vi "Laundry Tool (Commecial2) Main.vi"() -> ()   [LabVIEW 2021]
uses:
  Common/LabVIEW GEA2 Toolkit/GEA3/type defs/Data In.ctl
  Common/LabVIEW GEA2 Toolkit/GEA3/type defs/Source_Destination.ctl
  Common/LabVIEW GEA2 Toolkit/GEA3/type defs/Data Type.ctl
  Common/LabVIEW GEA2 Toolkit/GEA3/type defs/ERD Read Data In.ctl
  Laundry Tool Support/type defs/Programming.ctl
  Laundry Tool Support/type defs/Flash_Results.ctl
  Laundry Tool Support/type defs/Valves.ctl
  Laundry Tool Support/type defs/Cycle Control.ctl
  Laundry Tool Support/type defs/Motor Control.ctl
  Laundry Tool Support/type defs/MotorProfile.ctl
  Laundry Tool Support/type defs/Relays.ctl
  Laundry Tool Support/type defs/Select _Graph.ctl
  Laundry Tool Support/type defs/ERD_Graph.ctl
  Laundry Tool Support/type defs/ERD_Always_Show.ctl
  Laundry Tool Support/type defs/Redundant.ctl
  Laundry Tool Support/type defs/Algorithms.ctl
  Laundry Tool Support/type defs/ATC_Data.ctl
  Laundry Tool Support/type defs/OOB_Kicks_Brass.ctl
  Laundry Tool Support/type defs/Fault_Buffer_Status.ctl
  Common/GEA2 Script/typedefs/Script Info.ctl
  Laundry Tool Support/type defs/Diagnostics_Table.ctl
  Laundry Tool Support/type defs/Cycle_Diag_Buffer_Status.ctl
  Automation/Product Specific/Clothes Care/TL27/Product Testcode/VALEW/Fault Codes/subVIs/Snap_Input.ctl
  Automation/Product Specific/Clothes Care/TL27/Product Testcode/VALEW/Fault Codes/subVIs/Snap_Selection.ctl
  Dryer Tool (Commercial 2)/JL Dryer Tool Support/type defs/ERD_RJ45.ctl
  Dryer Tool (Commercial 2)/JL Dryer Tool Support/type defs/ERD_Commercial_Laundry.ctl
  Laundry Tool Support/type defs/BootloaderVersion.ctl
  Laundry Tool Support/type defs/Version.ctl
  Laundry Tool Support/type defs/ERD_Data_Loop_Control.ctl
  Laundry Tool Support/type defs/ERD_Loop_States.ctl
  Laundry Tool Support/type defs/Error_Command.ctl
  Laundry Tool Support/type defs/DAQ_States.ctl
  Common/GExplorer Support/typedefs/GExplorer_Data_Cluster.ctl
  Laundry Tool Support/type defs/Cont_Send_States.ctl
  Common/LabVIEW GEA2 Toolkit/GEA3/type defs/Data Out.ctl
  Laundry Tool Support/type defs/All_Bundled_Data.ctl
  Laundry Tool Support/type defs/Brass Matrix.ctl
  Laundry Tool Support/type defs/CSV_File_String_Arrays.ctl
  Laundry Tool Support/type defs/Fault Table Array.ctl
  Laundry Tool Support/type defs/Fault_Table_Info.ctl
  Common/LabVIEW GEA2 Toolkit/GEA3/type defs/ERD Write Data In.ctl
  Laundry Tool Support/type defs/DAQ_Control_Command.ctl
  Laundry Tool Support/type defs/ERD_Loop_Control_Command.ctl
  Laundry Tool Support/type defs/GEA2_Control_Command.ctl
  <vilib>/DAQmx/read.llb/DAQmx Read (Digital 1D Bool NChan 1Samp 1Line).vi
  <vilib>/DAQmx/read.llb/DAQmx Read (Digital 1D U8 1Chan NSamp).vi
  <vilib>/DAQmx/write.llb/DAQmx Write (Digital Bool 1Line 1Point).vi
  <vilib>/DAQmx/read.llb/DAQmx Read (Counter U32 1Chan 1Samp).vi
  <vilib>/DAQmx/write.llb/DAQmx Write (Analog 1D DBL NChan 1Samp).vi
  <vilib>/DAQmx/write.llb/DAQmx Write (Digital 1D Bool NChan 1Samp 1Line).vi
  Common/LabVIEW GEA2 Toolkit/GEA3/advanced/GEA2 Message Received Event Handler.vi
  <vilib>/DAQmx/create/channels.llb/DAQmx Create Channel (DO-Digital Output).vi
  <vilib>/DAQmx/create/channels.llb/DAQmx Create Channel (DI-Digital Input).vi
  <vilib>/DAQmx/configure/timing.llb/DAQmx Timing (Sample Clock).vi
  <vilib>/DAQmx/create/channels.llb/DAQmx Create Channel (CO-Pulse Generation-Frequency).vi
  <vilib>/DAQmx/configure/timing.llb/DAQmx Timing (Implicit).vi
  <vilib>/DAQmx/create/channels.llb/DAQmx Create Channel (CI-Count Edges).vi
  <vilib>/DAQmx/create/channels.llb/DAQmx Create Channel (AO-Voltage-Basic).vi
  <vilib>/DAQmx/miscellaneous.llb/DAQmx Fill In Error Info.vi
  D:/Common/LabVIEW GEA2 Toolkit/source/GEA3 DLL Source/GeaCommunication.dll
  Common/LabVIEW GEA2 Toolkit/source/GEA3 DLL Source/GeaCommunication.dll
  <resource>/objmgr/daqmx.rc
  Common/LabVIEW GEA2 Toolkit/GEA3/library/GEA2_Toolkit.lvlib
  Automation/Product Specific/Clothes Care/TLMB 2019/Projects/TLMB.lvlib
panel:
  in  "EndofCycle":bool
  in  "Board Index":u8=1 max=3 step=1
  in  "Rate":u32
  out "Boolean":bool
  out "String":string="Shutdown"
  in  "Data ON":bool=TRUE
  out "ERD_Always Show":T1
  in  "Stop":bool
  out "Fault Status":bool
  out "Log Rate (ms)":u32=68
  in  "Reset":bool
  in  "LEUI Launch":bool
  in  "HEUI Launch":bool
  in  "Tab Control":T2(tab)=enum."Scripting"
  in  "Phase.Authorized":bool
  in  "Phase.Reserved":bool
  in  "Phase.Idle":bool
  out "Personality Set":u8=1
  in  "?":u8
  in  "Set Personality":bool
  out "CSV File Log Path":path=path "D:/Laundry/FilesTemp/vvxc_[02_11_22_p. m.] [11_30_2021].csv"
  out "RJ45":T3
  out "Commercial_Laundry":T4
  out "Boot Loader Version":T5
  out "Application Version":T6
  in  "Write ERD List":T8(array[cluster])=[{"ERD Number"=0, "Data Type"=enum."string", "Data"=""}] {"ERD Number" format="%.0x"}
  in  "Write ERD":bool
  in  "Read ERD":bool
  in  "Read ERD List":T9[](array[typedef])=[{"ERD Number"=0, "Data Type"=enum."string"}] {"ERD Number" format="%.0x"}
  out "Read ERD Data Out":cluster{"ERD Number":u16, "Data":string}[](array[cluster]) {"ERD Number" format="%.0x"}
  in  "GEA Inputs":T10={"Source"=228, "Destination"=192} {"Destination" format="%.0x"; "Source" format="%.0x"}
  in  "IncrementPrice":T11 {"SANITIZE" min=0.0 max=9.75 step=0.25; "TOWELS" min=0.0 max=9.75 step=0.25; "COLORS" min=0.0 max=9.75 step=0.25; "WHITES" min=0.0 max=9.75 step=0.25; "DELICATES" min=0.0 max=9.75 step=0.25; "SPEED WASH" min=0.0 max=9.75 step=0.25}
  in  "SetIncrementPrices":bool
  in  "BasePrices":T11 {"SANITIZE" min=0.0 max=9.75 step=0.25; "TOWELS" min=0.0 max=9.75 step=0.25; "COLORS" min=0.0 max=9.75 step=0.25; "WHITES" min=0.0 max=9.75 step=0.25; "DELICATES" min=0.0 max=9.75 step=0.25; "SPEED WASH" min=0.0 max=9.75 step=0.25}
  in  "Set Price":bool
  in  "Send Button":bool
  in  "GEA2 Send":T12={"Source"=228, "Destination"=192, "Command"=0, "Message"=""} {"Command" format="%02x"; "Destination" format="%02x"; "Source" format="%02x"}
  in  "Msg Rate (ms)":u32=1000 min=50 step=50
  in  "Start Send":bool
  in  "Save Log":bool
  in  "GEA2 Log Length":i32=100000
  out "GEA2 Log":string
  in  "Clear":bool
  in  "Filter Log":bool
  in  "Cmd":string
  in  "Filter Data":bool
  in  "Programming":T13={"Program"=FALSE, "File Path"=path "", "Program Ind"=FALSE, "Result"=9, "Reset Board"=FALSE, "Enter Bootloader"=FALSE} {"Result" items=["ImageRejected", "BoardNotFound", "UnableToGetGeaConfiguration", "WriteToFlashNotAllowed", "ImageDownloadedSuccessfully", "ImagePresent", "WriteToFlashFailed", "EraseFailed", "CrcFailed", ""]}
  in  "Programming Destination Address":u8=35 format="%.0x"
  in  "ERD Graphing ON":bool
  out "ERD Graph  Ind":T15
  in  "ERD Graph Cntrl":T17={"ERD 3"={"ERD #"=61636, "Data Type"=enum."uint16_t", "Scaler"=32}, "ERD 2"={"ERD #"=61636, "Data Type"=enum."uint16_t", "Scaler"=32}, "ERD 1, ERD 2, & ERD3"={"ERD #"=61636, "Data Type"=enum."uint16_t", "Scaler"=32}} {"ERD 1, ERD 2, & ERD3"."Scaler" min=1; "ERD 1, ERD 2, & ERD3"."ERD #" format="%.0x"; "ERD 2"."Scaler" min=1; "ERD 2"."ERD #" format="%.0x"; "ERD 3"."Scaler" min=1; "ERD 3"."ERD #" format="%.0x"}
  in  "Graphing ON":bool
  in  "Select Graph":T18=enum."All Loads"
  out "Motor Current 2":dbl(graph)
  out "ERD 3":dbl(graph)
  out "ERD 2":dbl(graph)
  out "ERD 1":dbl(graph)
  out "Basket Speed 2":u16[][](graph)
  out "Temp 2":dbl(graph)
  out "Tub Gallons 2":dbl(graph)
  out "Pressure 3":dbl(graph)
  in  "OOB Kicks":T19
  out "All Loads":u16[][](graph)=[[0, 100, 200, 300, 400, 500, 600, 700, 800]]
  in  "Save Fault Log":bool
  in  "Clear Fault Table Buffer":bool
  in  "Clear Fault Seq Buffer":bool
  in  "Fault ON":bool
  out "Fault Table Buffer":string[][](table)
  out "Fault Sequence Buffer":string
  out "Seq Buffer Status":T20
  out "Table Buffer Status":T20
  in  "Clear Snapshots":bool
  in  "Get Snapshot Status":bool
  in  "Get Snapshot":bool
  in  "Select Snapshot":T21
  out "Fault Snapshots":T22
  out "Current Index":u16
  out "Count":u16
  out "Overwrite Count":u16
  out "Board Serial":string
  out "Board SKU":string
  in  "Get Board SKU and Serial":bool
  in  "Value":string
  in  "Register":string
  out "Value":string
  in  "Get Accel Reg":bool
  in  "Register":string
  in  "Set Accel Reg":bool
  in  "Relays":T23
  in  "Motor Profile":T24={"Start Profile"=FALSE, "Profile Selection"=14, "Stop Profile"=FALSE, "Pause Profile"=FALSE, "Resume Profile"=FALSE, "Select Profile"=FALSE}
  in  "Test Mode":cluster{"Exit Test Mode":bool}
  in  "LED Control":T25
  in  "Motor Control":T26 {"Amplitude (%)\n-CCW +CW" min=-100 max=100 step=5; "Acceleration" min=-400 max=400 step=10; "Motor Profile Mode" items=["Closed Loop", "Not Implemented", "Open Loop ", "Open Loop Angle ", "Coasting", "Braking", "Idle"]; "Speed (RPM)" min=-800 max=800 step=10}
  in  "Mode Shift":T27
  in  "Recirculation Pump":T28
  in  "Drain Pump":T29
  in  "Lid Lock":T30
  in  "Cycle Control":T31
  in  "Valve Control":T32
  in  "Save Cycle History Log":bool
  in  "Clear Cycle Buffer":bool
  out "Cycle Buffer Status":T33
  in  "Get Cycle History":bool
  out "Diagnostics Table":T34
  out "Redundant Micro":T35
  out "Algorithm Data":T36
  out "ATC Data":T37
  in  "ADC Info Button":bool
  out "Motor Current ADC":u16
  out "Pressure ADC":u16
  out "Temp ADC":u16
  in  "HE/LE ?":enum16{"HE", "LE"}(ring)
  in  "LL (M - A)":bool=TRUE
  in  "Lid Lock Feedback":bool
  in  "MS (M - A)":bool=TRUE
  out "DAQ Status":string="Exit"
  out "Drain Pump":bool
  out "Mode Shift":bool
  out "Recirc Pump":bool
  out "Cold Valve":bool
  out "Hot Valve":bool
  out "Spray/Rinse Valve":bool
  out "Fabric SoftValve":bool
  in  "AC Power":bool=TRUE
  in  "Mode Shift FB":bool
  in  "Lid Status":bool
  in  "Pressure":dbl(slide) min=0.0 max=5.0 step=0.5 scale=0.0..5.0 scale format="%#_3g"
  in  "Motor Current":dbl(slide)=2.5 min=0.0 max=5.0 step=0.5 scale=0.0..5.0 scale format="%#_3g"
  in  "Turn On DAQ":bool
  out "DAQ On?":bool
  in  "Basket RPM":dbl=1.0 min=1.0 max=800.0 step=5.0
  in  "Temperature":dbl(slide)=2.5 min=0.0 max=5.0 step=0.5 scale=0.0..5.0 scale format="%#_3g"
  out "Triac CW":bool
  out "Traic CCW":bool
  out "CCW":u32
  out "CW":u32
  in  "Script Log Path":path
  in  "Run Script":bool
  out "Script Pass/Fail?":bool
  out "Script Report Text":string
  in  "stop script":bool
  in  "Script Path":path
  out "Script Info":T38 {"Overall Script File Progress" scale=0.0..1.0; "Elapsed time (s)" format="%#.1f"; "Current Script Progress" scale=0.0..1.0}
  out "Script Error Out":errorcluster
  in  "ERD always show":T39(array[cluster])=[{"Boolean"=TRUE, "ERD Number"=61596, "ERD Name"="Erd_MC_WaterValvesActualState", "Data Type"=enum."string"}, {"Boolean"=TRUE, "ERD Number"=61551, "ERD Name"="Erd_MC_LidSwitchState", "Data Type"=enum."string"}, {"Boolean"=TRUE, "ERD Number"=61594, "ERD Name"="Erd_MC_DrainPumpActualState", "Data Type"=enum."string"}, {"Boolean"=TRUE, "ERD Number"=8236, "ERD Name"="Erd_Drive_SpeedSensorBasket", "Data Type"=enum."string"}, {"Boolean"=TRUE, "ERD Number"=8235, "ERD Name"="Erd_Drive_MotorTargetBasketSpeed", "Data Type"=enum."string"}, {"Boolean"=TRUE, "ERD Number"=65314, "ERD Name"="Erd_Drive_ModeShiftActualState", "Data Type"=enum."string"}, {"Boolean"=TRUE, "ERD Number"=61636, "ERD Name"="Erd_Drive_DCBusVoltageAd", "Data Type"=enum."string"}, {"Boolean"=TRUE, "ERD Number"=61546, "ERD Name"="Erd_CurrentCalibratedPressureInchesH2o", "Data Type"=enum."string"}, {"Boolean"=TRUE, "ERD Number"=61549, "ERD Name"="Erd_MC_TargetInGallonsx100", "Data Type"=enum."string"}, {"Boolean"=TRUE, "ERD Number"=61545, "ERD Name"="Erd_MC_CurrentTubInGallonsx100", "Data Type"=enum."string"}, {"Boolean"=TRUE, "ERD Number"=61611, "ERD Name"="Erd_Drive_LoadCurrentRms", "Data Type"=enum."string"}, {"Boolean"=TRUE, "ERD Number"=61544, "ERD Name"="Erd_MC_WetLoadGallons", "Data Type"=enum."string"}, {"Boolean"=TRUE, "ERD Number"=61555, "ERD Name"="Erd_MC_LidLockActualState", "Data Type"=enum."string"}, {"Boolean"=TRUE, "ERD Number"=61617, "ERD Name"="Erd_Drive_MotorMode", "Data Type"=enum."string"}, {"Boolean"=TRUE, "ERD Number"=61623, "ERD Name"="Erd_Drive_CycleEngineActualState", "Data Type"=enum."string"}, {"Boolean"=TRUE, "ERD Number"=8379, "ERD Name"="Erd_WaterTemperatureOption", "Data Type"=enum."string"}, {"Boolean"=TRUE, "ERD Number"=8382, "ERD Name"="Erd_SoilLevelOption", "Data Type"=enum."string"}, {"Boolean"=TRUE, "ERD Number"=8213, "ERD Name"="Erd_Remote_SoilLevelOption", "Data Type"=enum."string"}] {"ERD Number" format="%x"}
  in  "Basic ERDs":T39(array[cluster])=[{"Boolean"=FALSE, "ERD Number"=56, "ERD Name"="Erd_BootLoaderVersion", "Data Type"=enum."string"}, {"Boolean"=TRUE, "ERD Number"=8192, "ERD Name"="Erd_Remote_MachineState", "Data Type"=enum."string"}, {"Boolean"=TRUE, "ERD Number"=65280, "ERD Name"="Erd_Personality", "Data Type"=enum."string"}, {"Boolean"=TRUE, "ERD Number"=65356, "ERD Name"="Erd_Rj45LockedAtLeastOnce", "Data Type"=enum."string"}, {"Boolean"=TRUE, "ERD Number"=2, "ERD Name"="Erd_UnitSerialNumber", "Data Type"=enum."string"}, {"Boolean"=TRUE, "ERD Number"=8350, "ERD Name"="Erd_CommercialLaundryStatusExternal", "Data Type"=enum."string"}, {"Boolean"=TRUE, "ERD Number"=8351, "ERD Name"="Erd_CommercialLaundryStatus", "Data Type"=enum."string"}, {"Boolean"=TRUE, "ERD Number"=8397, "ERD Name"="Erd_RJ45WriteAccessReques", "Data Type"=enum."string"}, {"Boolean"=TRUE, "ERD Number"=8398, "ERD Name"="Erd_RJ45WriteAccessActual", "Data Type"=enum."string"}] {"ERD Number" format="%x"}
  in  "GEA Inputs 2":T10={"Source"=229, "Destination"=192} {"Destination" format="%.0x"; "Source" format="%.0x"}
  in  "Wifi State":T40(ring)
  in  "Set Wifi State(ERD 6003)":bool
  in  "Turn on Wifi":bool
  in  "Turn off Wifi":bool
  out "Wifi Network State":string
  out "Wifi Password":string
  out "Wifi Network Name":string
  out "Mac Address":string
  in  "Get Wifi Data":bool
  out "Error Out":errorcluster
  in  "Error In":errorcluster
  # "Ver. 1.2"
  # "Simular pago con aplicación 209E phase"
  # "Personality"
  # "Set Base Prices"
  # "Set Increment Prices"
  # "Must input a valid ERD# and Data Type\nDO NOT Leave Blank \nIf no scaler use value of 01"
  # "Accelermeter Registers"
  # "Wet Load Size"
  # "Dry Load Size"
  # "OOB"
  # "Wifi State is Writing to ERD 6003 and communicating with the wifi board directly.  It will remain in the state you wrote it to until another command is recieved. \n\nOnly Write to invalid if you are testing the board in Invalid state."
  # "After turning on Wifi , wait about 30 seconds and press the Get Wifi Data button.  Network state should be 1, apmode.\n\nAll this is doing is Writing the ERD 0xF115 Service Request to request connect, or disconnect."
  # "Contact:\n\nChris Schwalm\nChristopher.Schwalm@geappliances.com"
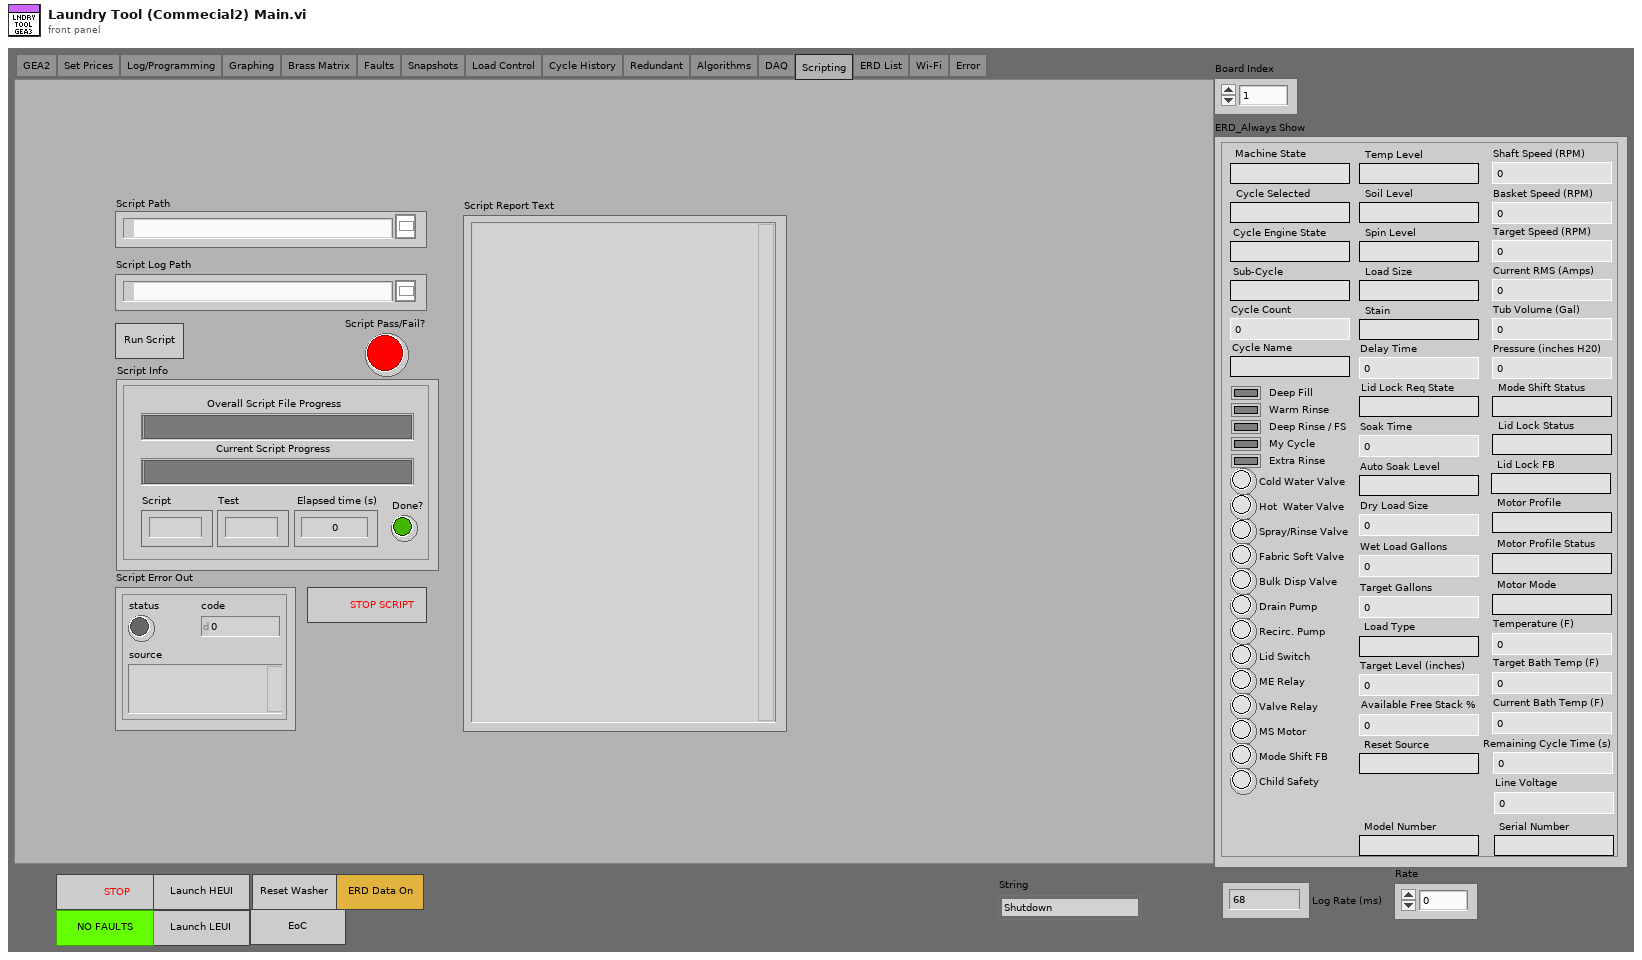
[diagram p1: front panel]
types:
  T1 = typedef "ERD_Always_Show.ctl" = cluster{"Basket Speed (RPM)":u16, "Machine State":string, "Tub Volume (Gal)":dbl, "Pressure (inches H20)":dbl, "Lid Switch ":bool, "Current RMS (Amps)":dbl, "Cycle Selected":string, "Lid Lock Status":string, "Mode Shift Status":string, "Spray/Rinse Valve":bool, "Fabric Soft Valve":bool, "Drain Pump":bool, "Recirc. Pump":bool, "Cycle Engine State":string, "Hot  Water Valve":bool, "Cold Water Valve":bool, "Motor Profile":string, "Motor Profile Status":string, "Motor Mode":string, "ME Relay":bool, "Cycle Count":u32, "Deep Rinse / FS":bool, "My Cycle":bool, "Soil Level":string, "Spin Level":string, "Stain":string, "Temp Level":string, "Load Size":string, "Delay Time":u16, "Soak Time":u16, "Deep Fill":bool, "Warm Rinse":bool, "Auto Soak Level":string, "Extra Rinse":bool, "Wet Load Gallons":dbl, "Target Gallons":dbl, "Sub-Cycle":string, "Load Type":string, "Target Level (inches)":dbl, "Valve Relay":bool, "Dry Load Size":dbl, "Shaft Speed (RPM) ":u16, "MS Motor":bool, "Mode Shift FB":bool, "Target Bath Temp (F)":dbl, "Temperature (F)":dbl, "Current Bath Temp (F)":dbl, "Lid Lock FB":string, "Lid Lock Req State":string, "Remaining Cycle Time (s)":u32, "Available Free Stack %":u8, "Child Safety":bool, "Target Speed (RPM)":u16, "Reset Source":string, "Line Voltage":dbl, "Cycle Name":string, "Bulk Disp Valve":bool, "Model Number":string, "Serial Number":string}
  T2 = enum32{"GEA2", "Set Prices", "Log/Programming", "Graphing", "Brass Matrix", "Faults", "Snapshots", "Load Control", "Cycle History", "Redundant", "Algorithms", "DAQ", "Scripting", "ERD List", "Wi-Fi", "Error"}
  T3 = typedef "ERD_RJ45.ctl" = cluster{"Write Access Actual":string, "Write Access Request":string, "LockedAtLeastOnce":string}
  T4 = typedef "ERD_Commercial_Laundry.ctl" = cluster{"Session":string, "Phase":string, "Appliance Type":string, "Cycle Selected":string, "Platform Type":string, "Retry Signal":string, "Session Ext":string, "Phase Ext":string, "Appliance Type Ext":string, "Cycle Selected Ext":string, "Platform Type Ext":string, "Retry Signal Ext":string}
  T5 = typedef "BootloaderVersion.ctl" = cluster{"UI BL Version":string, "MC BL Version":string}
  T6 = typedef "Version.ctl" = cluster{"Build Number":string, "Build Hash ":string, "Application Version":string, "Parametric Version":string, "UI App Version":string}
  T7 = typedef "Data Type.ctl" = enum16{"string", "boolean", "uint8_t", "uint16_t", "uint32_t", "uint64_t", "int8_t", "int16_t", "int32_t", "int64_t"}
  T8 = cluster{"ERD Number":u16, "Data Type":T7, "Data":string}[]
  T9 = typedef "ERD Read Data In.ctl" = cluster{"ERD Number":u16, "Data Type":enum16{"string", "boolean", "uint8_t", "uint16_t", "uint32_t", "uint64_t", "int8_t", "int16_t", "int32_t", "int64_t"}}
  T10 = typedef "Source_Destination.ctl" = cluster{"Source":u8, "Destination":u8}
  T11 = cluster{"SPEED WASH":dbl, "DELICATES":dbl, "WHITES":dbl, "COLORS":dbl, "TOWELS":dbl, "SANITIZE":dbl}
  T12 = typedef "Data In.ctl" = cluster{"Source":u8, "Destination":u8, "Command":u8, "Message":string}
  T13 = typedef "Programming.ctl" = cluster{"Program":bool, "File Path":path, "Program Ind":bool, "Result":T14, "Reset Board":bool, "Enter Bootloader":bool}
  T14 = typedef "Flash_Results.ctl" = i32
  T15 = cluster{"ERD Value 1":dbl, "ERD Value 2":dbl, "ERD Value 3":dbl}
  T16 = typedef "ERD_Graph.ctl" = cluster{"ERD #":u16, "Data Type":T7, "Scaler":u32}
  T17 = cluster{"ERD 3":T16, "ERD 2":T16, "ERD 1, ERD 2, & ERD3":T16}
  T18 = typedef "Select _Graph.ctl" = enum16{"Temperature (F)", "Basket Speed (RPM)", "Tub Volume (Gal)", "Pressure (in H2O)", "Current RMS (Amps)", "ERD 1", "ERD 2", "ERD 3", "All Loads"}
  T19 = typedef "OOB_Kicks_Brass.ctl" = cluster{"OOB in Accel":bool, "OOB in S-S":bool, "Redist Req":bool, "Suds Abtmt Req":bool}
  T20 = typedef "Fault_Buffer_Status.ctl" = cluster{"Current Index":u16, "Count":u16, "Overwrite Count":u16}
  T21 = typedef "Snap_Selection.ctl" = enum16{"SnapShot Record 0 - E10F", "Snapshot Record 1 - E110", "Snapshot Record 2 - E111", "Snapshot Record 3 - E112", "Snapshot Record 4 - E113", "Snapshot Record 5 - E114", "Snapshot Record 6 - E115", "Snapshot Record 7 - E116", "Snapshot Record 8 - E117", "Snapshot Record 9 - E118"}
  T22 = typedef "Snap_Input.ctl" = cluster{"Fault ID":string, "Cycle Count":u32, "Cycle ID":string, "Time Stamp":u32, "Stuck Key Mask":string, "Machine State":string, "Subcycle State":string, "Hot Valve":string, "Cold Valve":string, "Spray Valve":string, "Fabric Softener Valve":string, "Bulk Valve":string, "Drain Pump State":string, "Lid Lock Actual":string, "Lid Lock Request":string, "Lid Switch State":string, "ModeShift Feeback":string, "Recirc Pump State":string, "Modeshift Requested":string, "Modeshift Actual":string, "Motor Mode":string, "Target Speed":u16, "Target Accel":u16, "Current RMS(AMPS)":dbl, "Line Voltage":dbl, "Target Gallons":dbl, "Tub Volume (Gal)":dbl, "Hot Gallons":dbl, "Cold Gallons":dbl, "Target Level (Inches)":dbl, "Pressure (Inches H20) ":dbl, "Pressure Calibration":dbl, "OOB Accel":i32, "OOB Jerk":i32, "OOB SS":i32, "OOB Folding":i32, "Accelerometer Peak":i16, "Accelerometer Base":i16, "Accel Points":u8, "SS Points":u8, "Deep Fill Option":string, "WoD Option":string, "Basket Speed":u16}
  T23 = typedef "Relays.ctl" = cluster{"Relays ON":bool, "Relays OFF":bool}
  T24 = typedef "MotorProfile.ctl" = cluster{"Start Profile":bool, "Profile Selection":u8, "Stop Profile":bool, "Pause Profile":bool, "Resume Profile":bool, "Select Profile":bool}
  T25 = cluster{"ALL LEDs ON":bool, "ALL LEDs OFF":bool, "Reset LEDs":bool}
  T26 = typedef "Motor Control.ctl" = cluster{"Speed (RPM)":i16, "Motor Profile Mode":u16, "Acceleration":i16, "Angle (Degrees)":i16, "Amplitude (%)\n-CCW +CW":i16, "Start Motor":bool, "Stop Motor":bool}
  T27 = cluster{"Shift to Agitate":bool, "Shift to Spin":bool, "Disable":bool}
  T28 = cluster{"Recirc Pump ON":bool, "Recirc Pump OFF":bool, "Reset Recirc Pump":bool}
  T29 = cluster{"Drain Pump ON":bool, "Drain Pump OFF":bool, "Reset Drain Pump":bool}
  T30 = cluster{"Lock Lid":bool, "Unlock Lid":bool, "Reset Lock":bool}
  T31 = typedef "Cycle Control.ctl" = cluster{"Start Cycle":bool, "Cycle Selection":u8, "Stop Cycle":bool, "Pause Cycle":bool, "Resume Cycle":bool, "Select Cycle":bool}
  T32 = typedef "Valves.ctl" = cluster{"Cold Valve":bool, "SprayRinse Valve":bool, "FabricSoftener Valve":bool, "Valves ON":bool, "Valves OFF":bool, "Hot Valve ":bool, "Bulk Dispense Valve":bool}
  T33 = typedef "Cycle_Diag_Buffer_Status.ctl" = cluster{"Current Index":u16, "Count":u16, "Overwrite Count":u16}
  T34 = typedef "Diagnostics_Table.ctl" = string[][]
  T35 = typedef "Redundant.ctl" = cluster{"Version":string, "Personality":u8, "Pressure ":dbl, "Shaft Speed":u16, "Modeshift Feedback":string, "Lid Switch":bool, "Lid Lock":bool, "Triac Enable":bool, "Drain Pump":bool, "Lid Lock Motor Speed Safety Interlock":bool, "Flood Condition State":bool, "Lid Open Fault State":bool, "Access To Moving Parts State":bool, "Heartbeat":bool, "Motor Enable":bool, "Lid Unlock Fault State":bool}
  T36 = typedef "Algorithms.ctl" = cluster{"Wet Load Gal":dbl, "Target Gallons":dbl, "Load Type":string, "Load Size":string, "Coast Time":u16, "Ramp Time":u16, "Ramp  Speed":u16, "Ramp Avg Current":dbl, "OOB Redist Req":bool, "OOB Detected in S-S":bool, "Folding in Accel":i32, "Max Jerk in Accel":i32, "Max Jerk in S-S":i32, "OOB Detected in Accel":bool, "Partial Coast Time":u16, "Dry Load Size":dbl, "Ramp Line Voltage ":dbl, "Coast Line Voltage":dbl, "Suds Abatement Req ":bool}
  T37 = typedef "ATC_Data.ctl" = cluster{"Current Tub Gallons":dbl, "Hot Gallons":dbl, "Cold Gallons":dbl, "Target Gallons":dbl, "Current Water Temp":dbl, "Target Level":dbl, "Target Bath Temp":dbl, "Current Bath Temp ":dbl, "Cold Inlet Temp":dbl, "Hot Inlet Temp":dbl, "Warm Inlet Temp":dbl, "Hot Seg Valve Time":u16, "Cold Seg Valve Time ":u16, "User Temp Level":string, "Segment Gallons":dbl}
  T38 = typedef "Script Info.ctl" = cluster{"Overall Script File Progress":dbl, "Current Script Progress":dbl, "Script":string, "Test":string, "Elapsed time (s)":dbl, "Done?":bool}
  T39 = cluster{"Boolean":bool, "ERD Number":u16, "ERD Name":string, "Data Type":enum16{"string", "boolean", "uint8_t", "uint16_t", "uint32_t", "uint64_t"}}[]
  T40 = enum16{"0 - OFF", "1 - App Mode", "2 - Connecting", "3 - Connected", "4 - Connected Off", "5 - Scanning", "6 - Reconnecting", "255 - Invalid"}
  T41 = typedef "All_Bundled_Data.ctl" = cluster{"Software MC":T6, "ERD_Always Show":T1, "Personality Set":u8, "Brass Matrix":T42, "CSV File String Arrays":T43, "Redundant Micro":T35, "Algorithm Data":T36, "ATC Data":T37, "Fault Table Array ":T44, "RJ45":T3, "Commercial_Laundry":T4, "Boot Loader Version":T5}
  T42 = typedef "Brass Matrix.ctl" = cluster{"Shaft Speed":u16, "Folding":i32, "Jerk":i32, "Basket Speed":u16, "Target Speed":u16, "Peak Signal":u8, " Peak Magnitude":dbl, "Folding in Accel":i32, "Max Jerk in Accel":i32, "Max Jerk in S-S":i32, "Motor Profile Status":string, "Motor Profile":string, "OOB Redist Req":bool, "OOB Detected in S-S":bool, "OOB Detected in Accel":bool, "Suds Abatement Req ":bool, "Peak Dir":bool, "Peak Vector":dbl, "S-S Points":u8, "Points":u8, "Jerk Delta":i32}
  T43 = typedef "CSV_File_String_Arrays.ctl" = cluster{"ERD Number Array":string[], "ERD Name Array":string[], "ERD Converted String Data":string[]}
  T44 = typedef "Fault Table Array.ctl" = T45[]
  T45 = typedef "Fault_Table_Info.ctl" = cluster{"Cycle Count":u32, " Runtime (min) ":u32, "Fault Status":string, "Fault ID":string, "Fault Count":u16}
  T46 = typedef "Cont_Send_States.ctl" = enum16{"Run", "Shutdown"}
  T47 = typedef "GExplorer_Data_Cluster.ctl" = cluster{"Data":variant, "State":enum16{"Add to Log", "Clear", "Shutdown"}}
  T48 = typedef "DAQ_States.ctl" = enum16{"Wait for Init", "Rename Devices", "Verify Hardware", "Initialize", "Run", "Shutdown", "Exit"}
  T49 = typedef "ERD_Data_Loop_Control.ctl" = cluster{"Data":variant, "State":T50}
  T50 = typedef "ERD_Loop_States.ctl" = enum16{"Init", "Get Version", "Build ERD Read List", "Read ERDs", "Update UI", "Update Graphs", "Read Faults", "Log Data", "Pause", "Brass Logging", "Shutdown"}
  T51 = typedef "Error_Command.ctl" = enum16{"Initialize", "Handle Errors", "Report Errors"}
  T52 = typedef "ERD Write Data In.ctl" = cluster{"ERD Number":u16, "Data Type":T7, "Data":string}
  T53 = enum8{"Enabled", "Disabled", "Disabled and Grayed Out"}
  T54 = typedef "GEA2_Control_Command.ctl" = enum16{"Initialize", "Shutdown"}
  T55 = typedef "ERD_Loop_Control_Command.ctl" = enum16{"Initialize", "Shutdown"}
  T56 = typedef "DAQ_Control_Command.ctl" = enum16{"Initialize", "Shutdown", "Exit"}
  T57 = typedef "Data Out.ctl" = cluster{"Source":u8, "Destination":u8, "Command":u8, "Length":u8, "CRC":u16, "Message":string}
  T58 = cluster{"ERD Data Out[0]":cluster{"ERD Number":u16, "Data":string}, "ERD Data Out[1]":cluster{"ERD Number":u16, "Data":string}, "ERD Data Out[2]":cluster{"ERD Number":u16, "Data":string}, "ERD Data Out[3]":cluster{"ERD Number":u16, "Data":string}, "ERD Data Out[4]":cluster{"ERD Number":u16, "Data":string}, "ERD Data Out[5]":cluster{"ERD Number":u16, "Data":string}, "ERD Data Out[6]":cluster{"ERD Number":u16, "Data":string}, "ERD Data Out[7]":cluster{"ERD Number":u16, "Data":string}, "ERD Data Out[8]":cluster{"ERD Number":u16, "Data":string}}
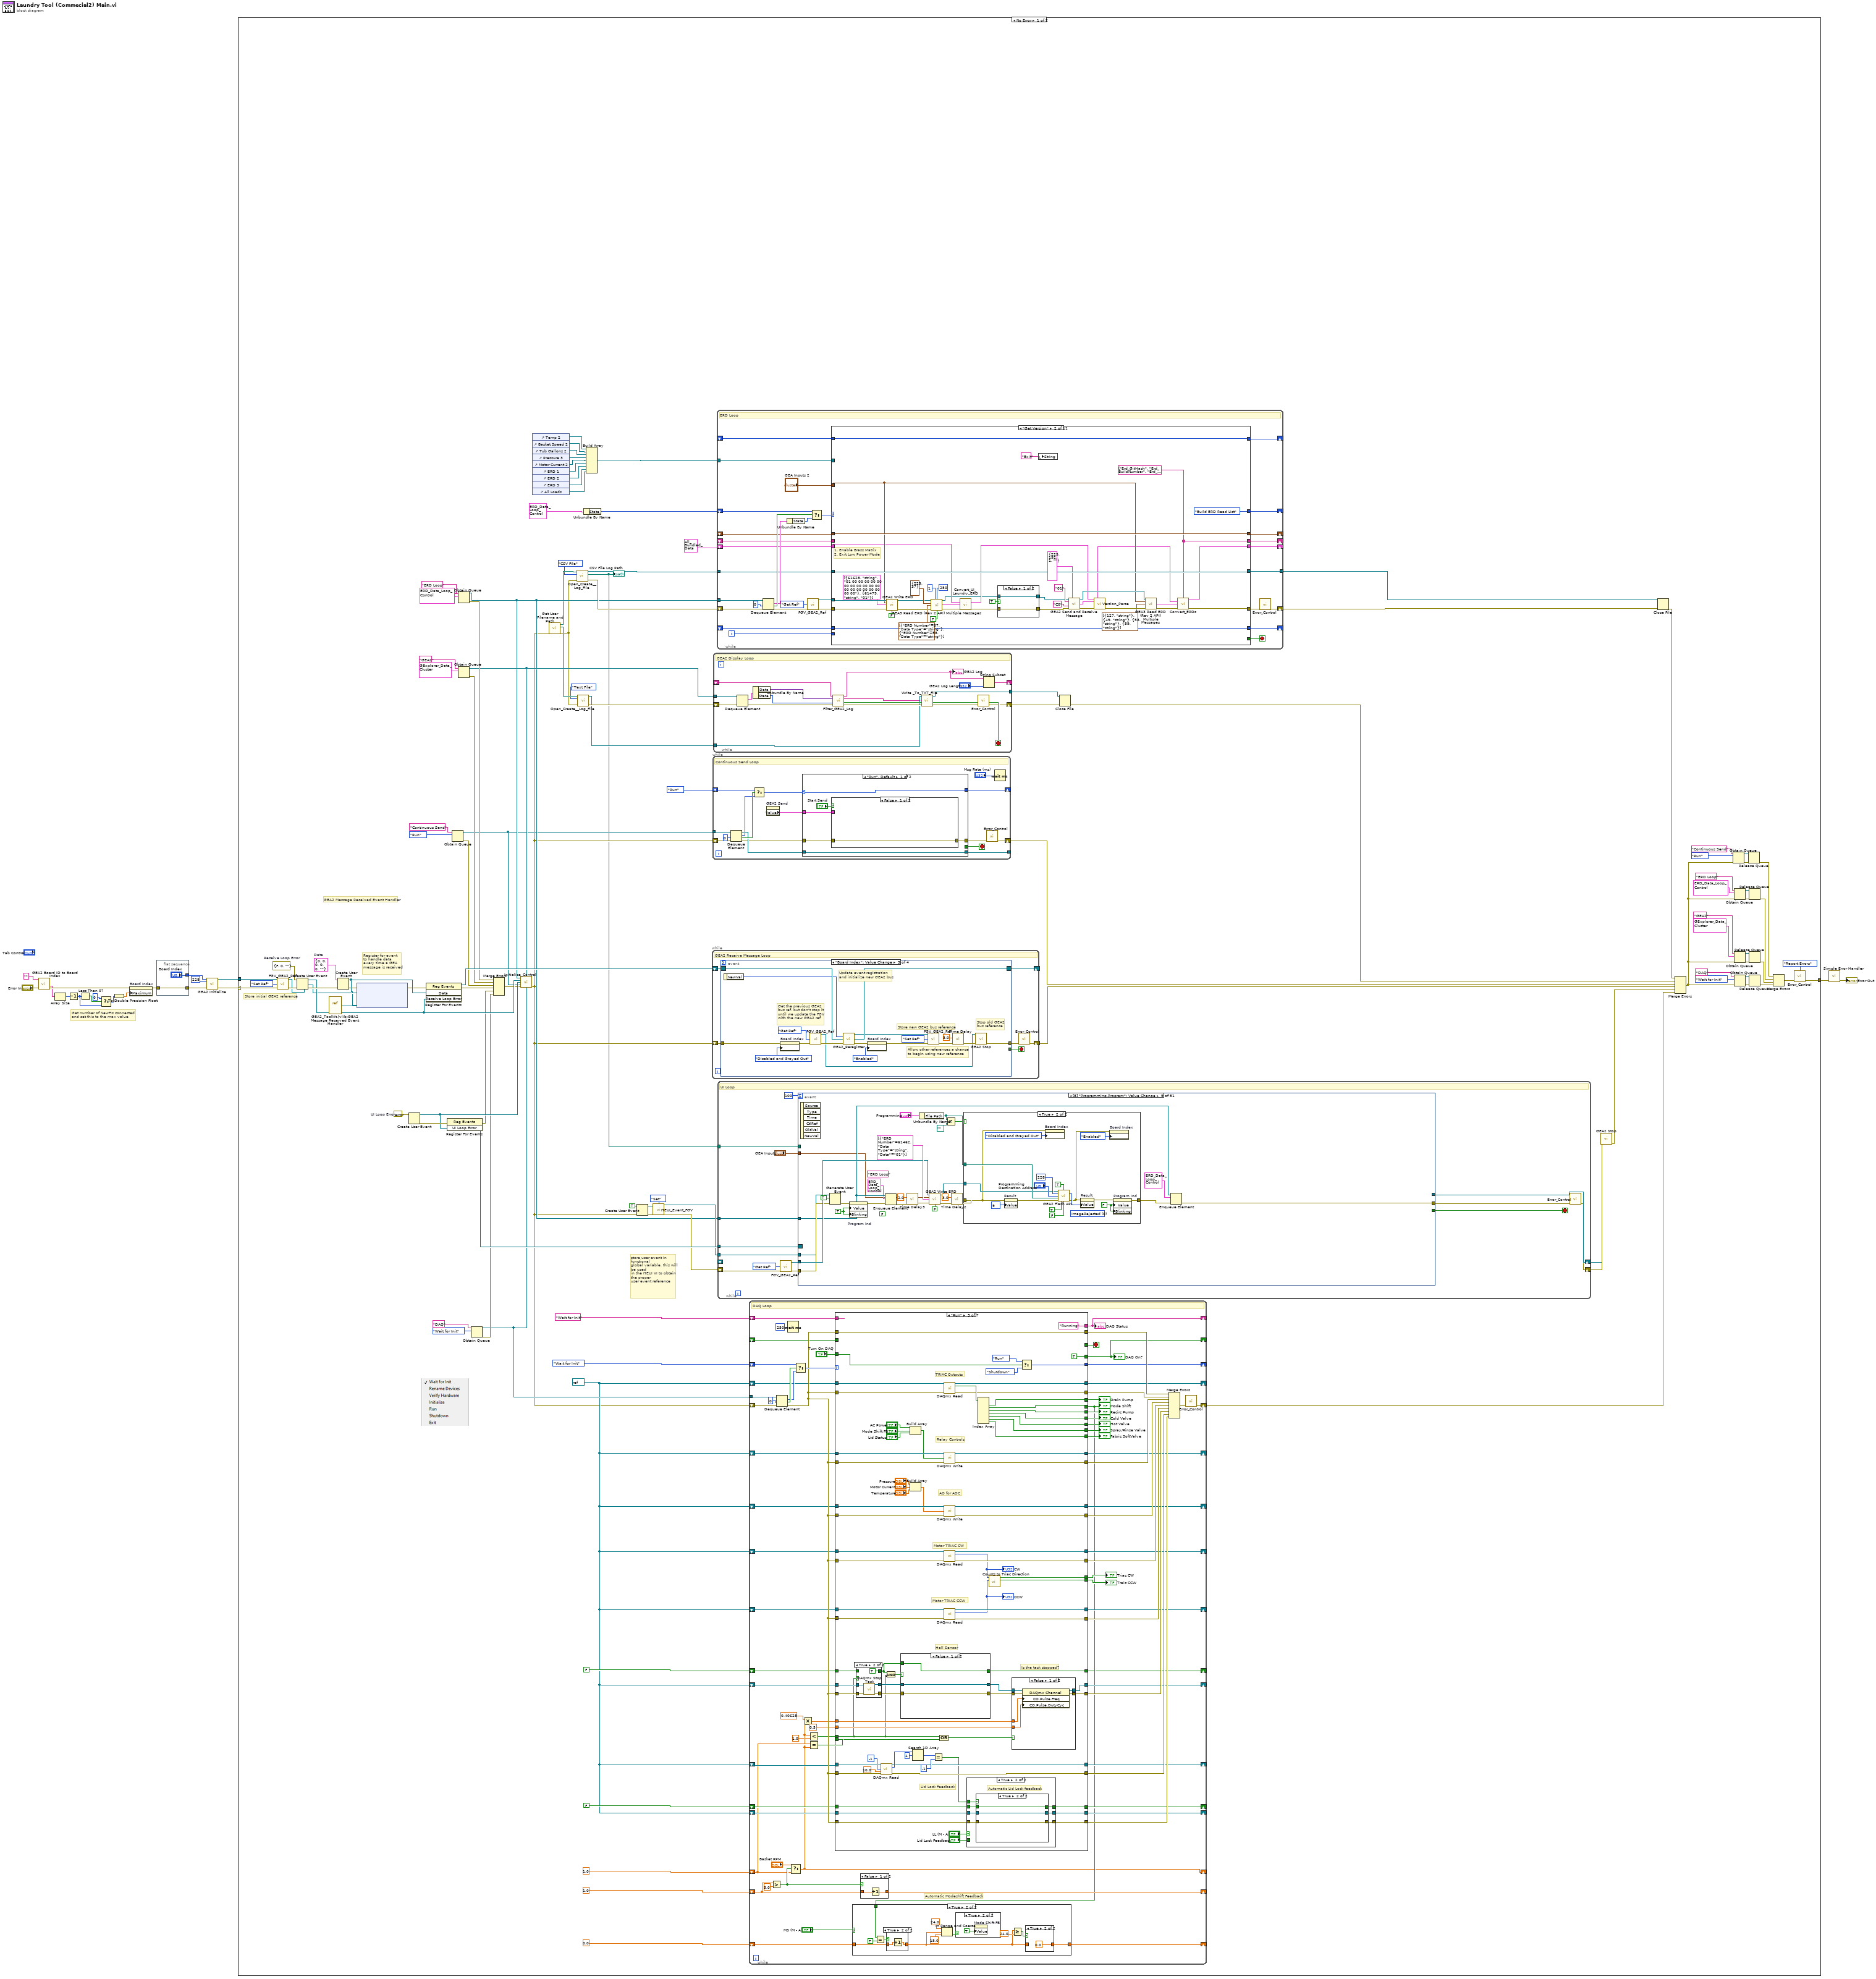
[diagram p0: block diagram]
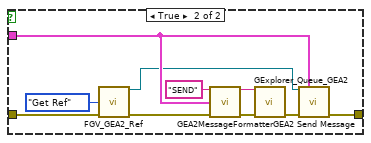
[diagram p2: hidden frame]
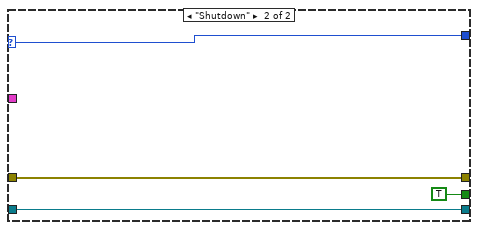
[diagram p3: hidden frame]
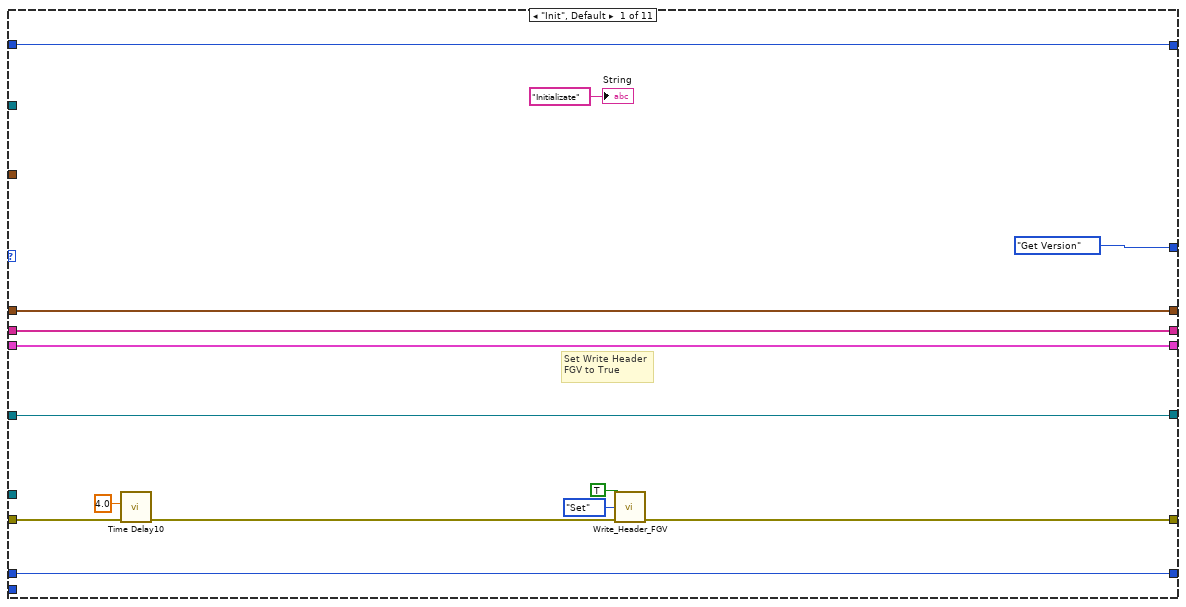
[diagram p4: hidden frame]
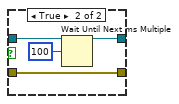
[diagram p5: hidden frame]
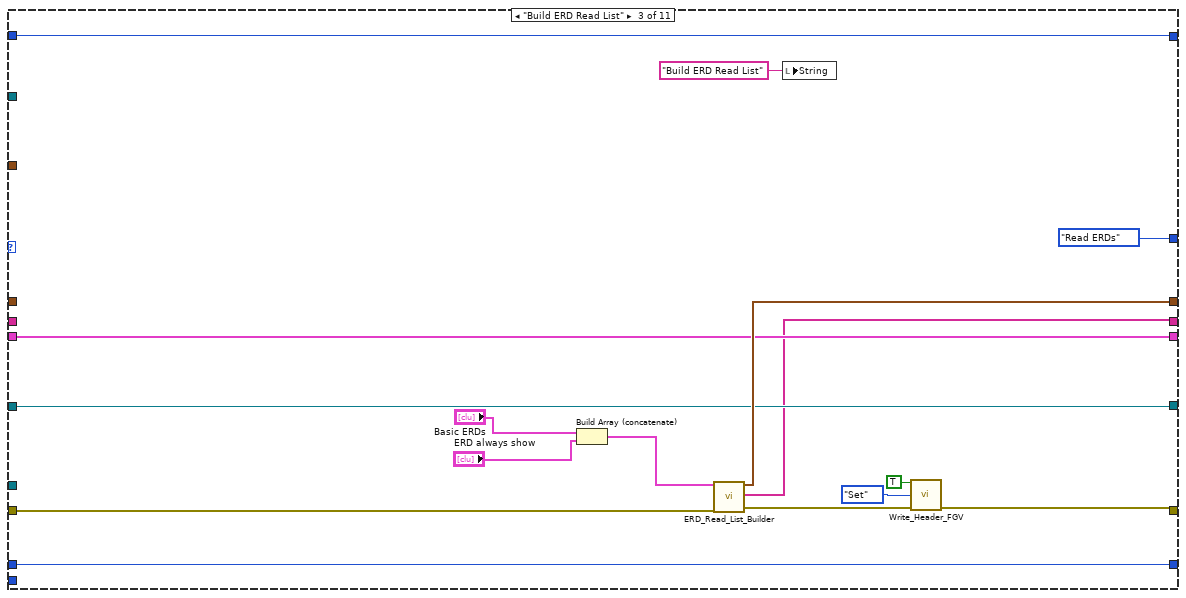
[diagram p6: hidden frame]
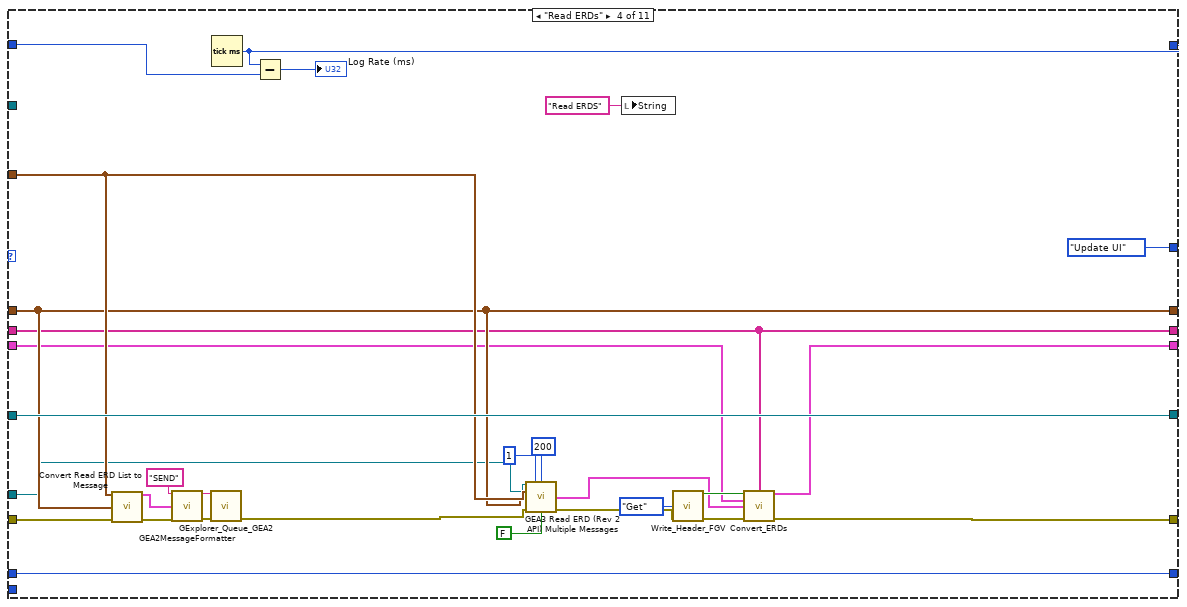
[diagram p7: hidden frame]
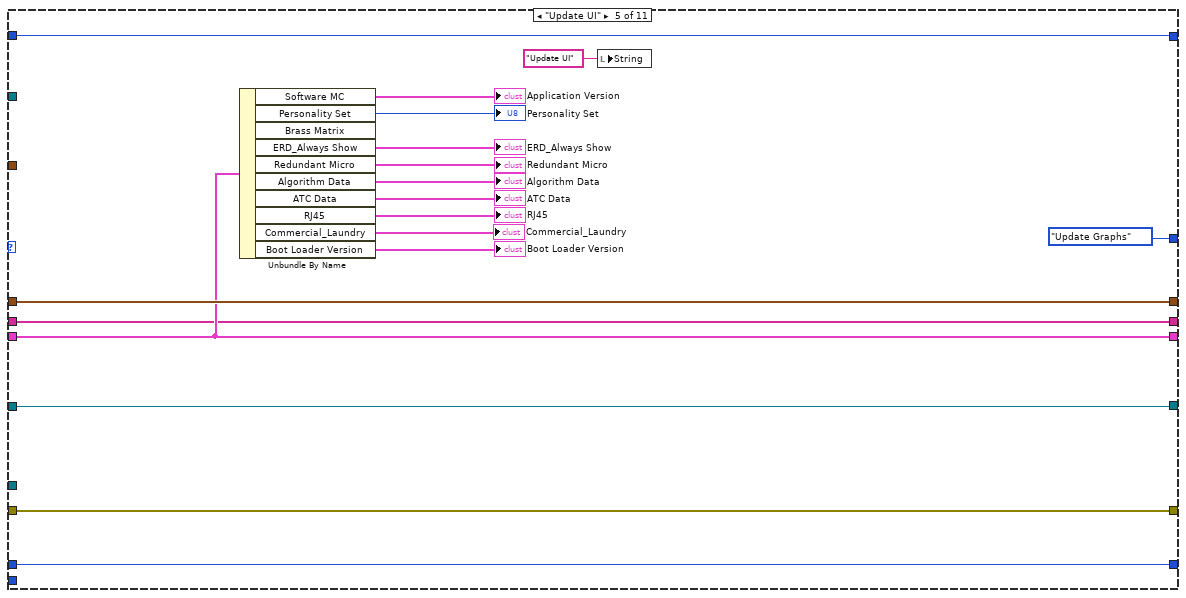
[diagram p8: hidden frame]
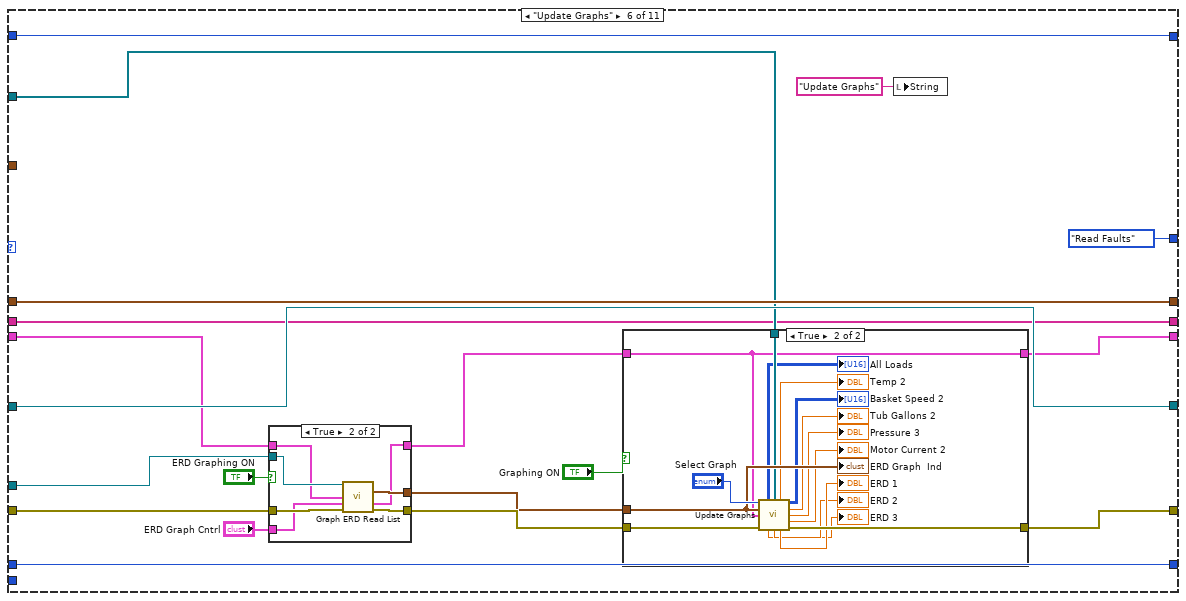
[diagram p9: hidden frame]
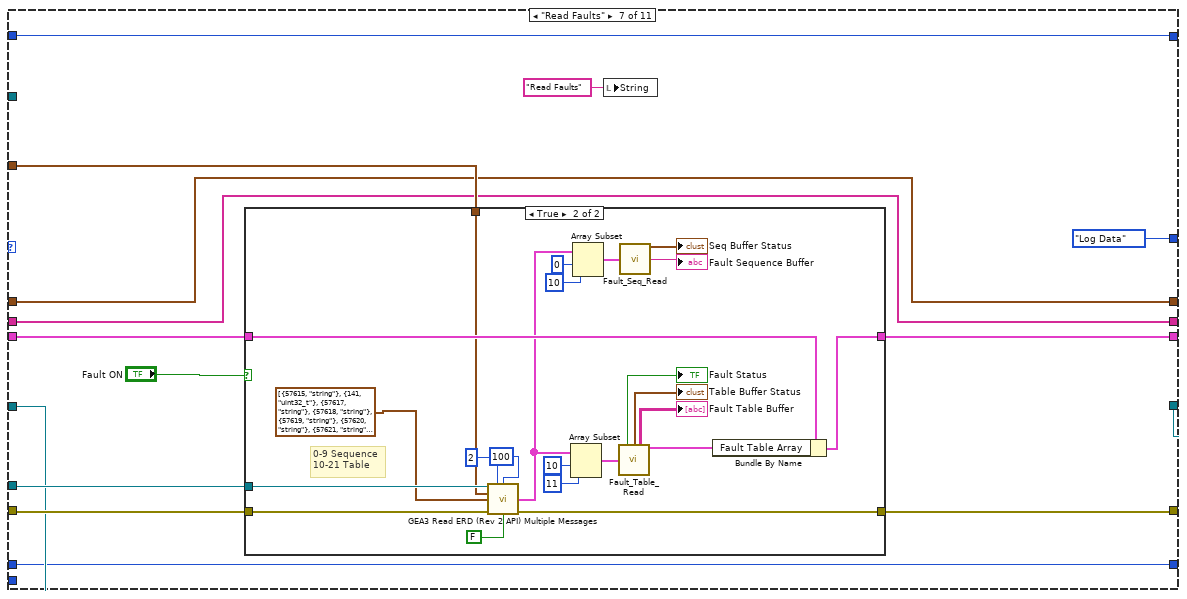
[diagram p12: hidden frame]
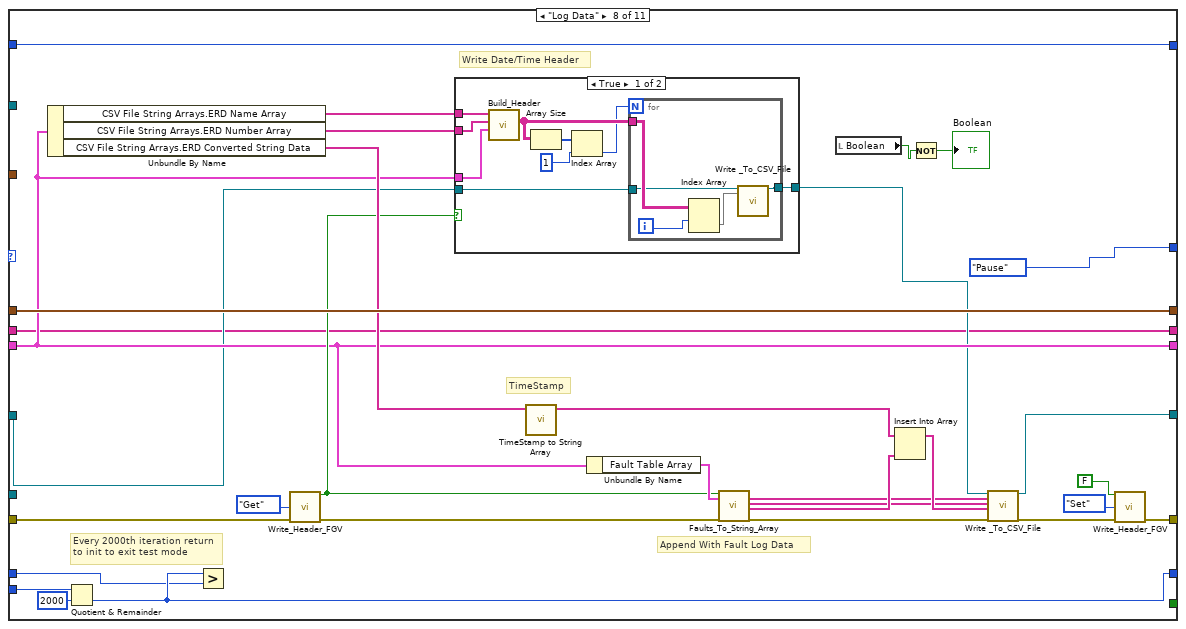
[diagram p14: hidden frame]
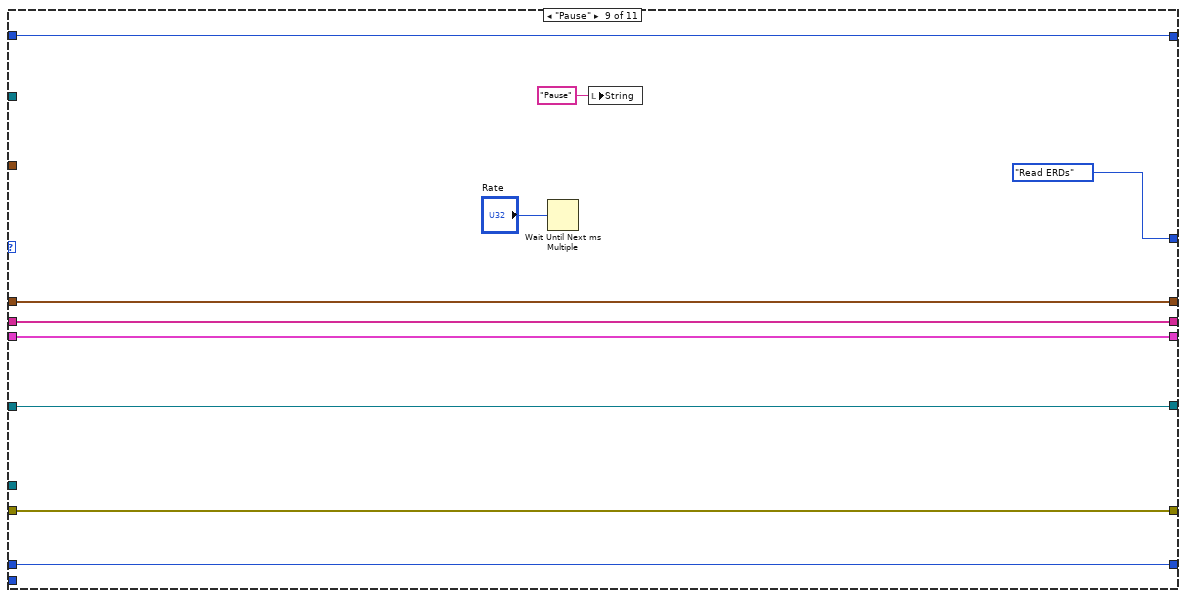
[diagram p16: hidden frame]
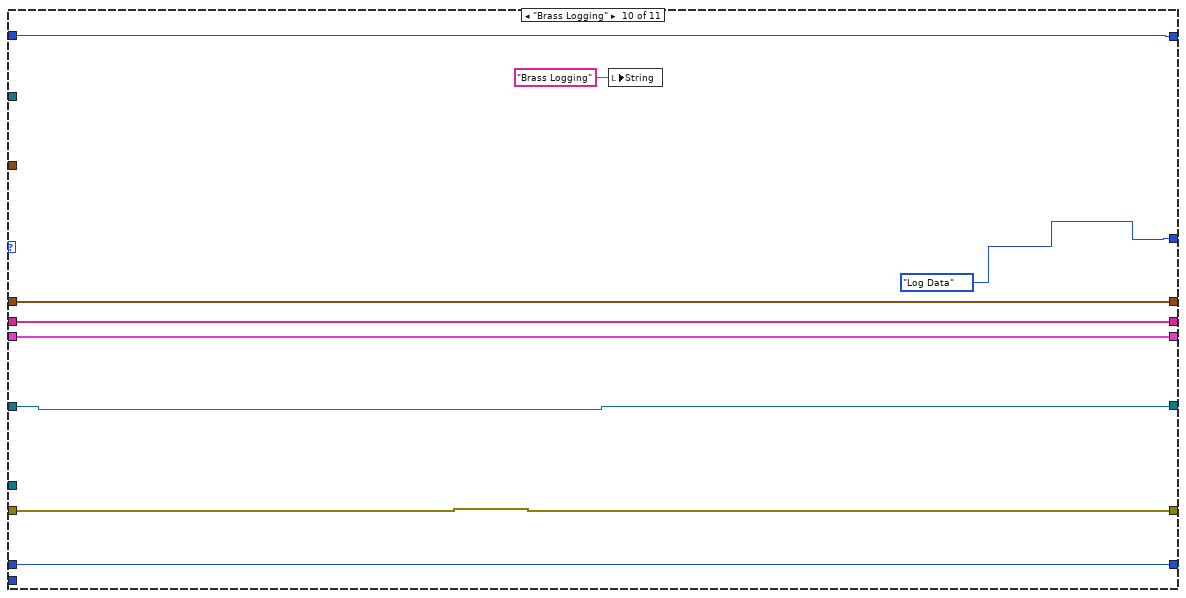
[diagram p17: hidden frame]
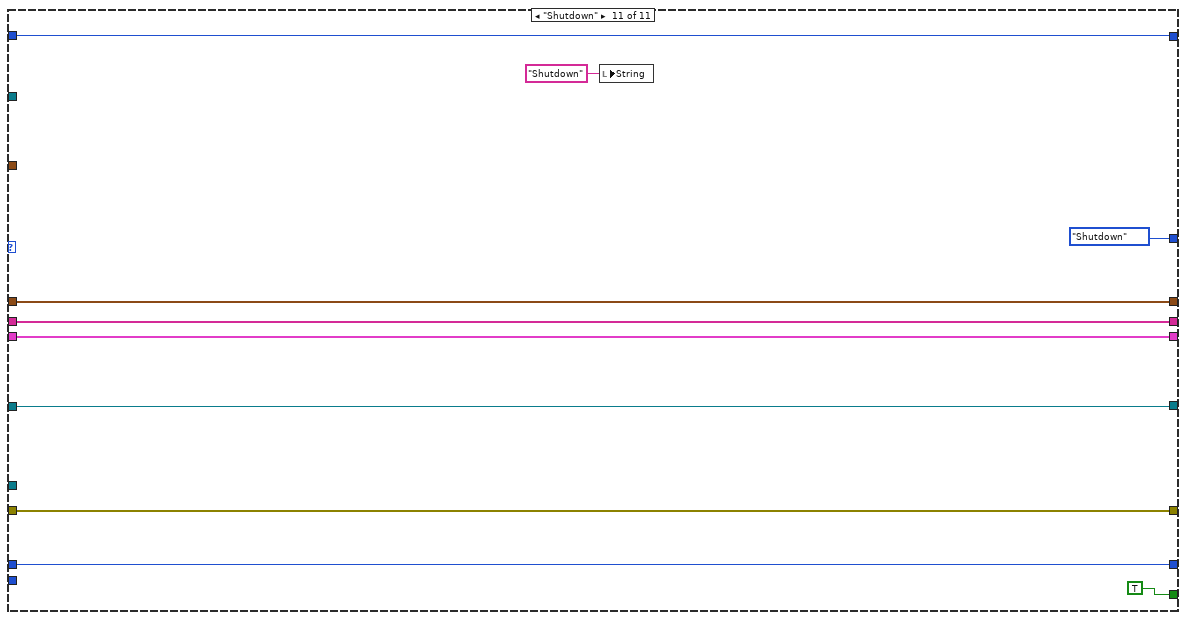
[diagram p18: hidden frame]
diagram:
  # "Get number of NewFIs connected\nand set this to the max value"
  n1 = call "GEA2 Board ID to Board Index.vi"("Board ID"="", "Error In"="Error In") -> ("Boards Found"=w5:string[], "Error Out"=w14:errorcluster)  [unwired: 9 in, 3 out]
  n2 = Array Size(array=w5) -> (size(s)=w10:i32)
  n3 = Decrement(x=w10) -> (x-1=w8:i32)
  n4 = Less Than 0?(x=w8) -> (x < 0?=w9:bool)
  n5 = Select(t=0, s=w9, f=w8) -> (s? t:f=w6:i32)
  n6 = To Double Precision Float(number=w6) -> (double precision float=w4:dbl)
  n7 = property on="Board Index" class="DigNum (strict)"(error in=w14, "Maximum"=w4) -> (error out=w12:errorcluster)  [unwired: 1 in, 1 out]
  n8 = flat-sequence {
    tunnel: ["Board Index"] -> w1
    tunnel: w12 -> [w19]
    tunnel: [w19] -> w11
    frame #0 {
    }
  }
  n9 = call "GEA2 Initialize.vi"("Board Index"=w1, "Source Address"=u8 228, "error in"=w11) -> ("GEA2 Reference Out"=w17:refnum<k24>, "error out"=w16:errorcluster)  [unwired: 10 in, 1 out]
  n10 = case shown="No Error" w16 {
    selector: w16 -> [w90 w2695]
    tunnel: w17 -> [w88 _]
    tunnel: [w92 w2695] -> w3
    frame No Error {
      w41 = errorcluster {"status"=FALSE, "code"=0, "source"=""}  # Receive Loop Error
      w42 = T57 {"Source"=0, "Destination"=0, "Command"=0, "Length"=0, "CRC"=0, "Message"=""}  # Data
      w57 = refnum<k21> refnum ("task out")
      w126 = errorcluster {"status"=FALSE, "code"=0, "source"=""}  # UI Loop Error
      # "GEA2 Message Received Event Handler"
      # "store user event in functional\nglobal variable, this will be used\nin the HEUI VI to obtain the proper\nuser event reference"
      # "Store initial GEA2 reference"
      # "Register for event\nto handle data\nevery time a GEA\nmessage is received"
      n11 = call "FGV_GEA2_Ref.vi"("GEA2 Reference In"=w88, "Action"=enum16{"Set Ref", "Get Ref"}."Set Ref", "Error In"=w90) -> ("GEA2 Reference Out"=w28:refnum<k24>, "Error Out"=w89:errorcluster)  [unwired: 11 in]
      n12 = Create User Event(user event datatype=w41, error in=w89) -> (user event=w127:refnum<user-event>, error out=w128:errorcluster)
      n13 = vi-ref "GEA2_Toolkit.lvlib:GEA2 Message Received Event Handler.vi"() -> (w27:refnum<vi>)
      n14 = Create User Event(user event datatype=w42, error in=w128) -> (user event=w26:refnum<user-event>, error out=w24:errorcluster)
      n15 = node(w24, w28, w27, w26) -> (w25:errorcluster)  [unwired: 1 in, 1 out]
      n16 = Create User Event(user event datatype=w126) -> (user event=w115:refnum<user-event>, error out=w125:errorcluster)  [unwired: 1 in]
      n17 = register-events(error in=w25, w26, w127) -> (reference out=w124:refnum<event-registration>, error out=w97:errorcluster)  [unwired: 1 in]
      n18 = register-events(error in=w125, w115) -> (reference out=w106:refnum<event-registration>, error out=w96:errorcluster)  [unwired: 1 in]
      n19 = Obtain Queue(name (unnamed)="Continuous Send", element data type=Cont_Send_States."Run" ("State")) -> (queue out=w43:refnum<queue>, error out=w48:errorcluster)  [unwired: 3 in, 1 out]
      n20 = Obtain Queue(name (unnamed)="ERD Loop", element data type=T49 {"Data"=variant, "State"=enum."Read ERDs"} ("Data")) -> (queue out=w77:refnum<queue>, error out=w93:errorcluster)  [unwired: 3 in, 1 out]
      n21 = Obtain Queue(name (unnamed)="GEA2", element data type=T47 {"Data"=variant, "State"=enum."Add to Log"} ("Data")) -> (queue out=w78:refnum<queue>, error out=w98:errorcluster)  [unwired: 3 in, 1 out]
      n22 = Obtain Queue(name (unnamed)="DAQ", element data type=DAQ_States."Wait for Init" ("States")) -> (queue out=w65:refnum<queue>, error out=w95:errorcluster)  [unwired: 3 in, 1 out]
      n23 = Merge Errors(w93, w98, w48, w97, w96, w95) -> (w94:errorcluster)
      n24 = call "Initialize_Control.vi"("ERD Loop"=w77, "GEA2"=w78, "Receive Loop"=w127, "UI Loop Error"=w115, "Cont Send"=w43, "Error In"=w94, "DAQ"=w65) -> ("Error Out"=w29:errorcluster)  [unwired: 8 in]
      n25 = control-ref of="Temp 2"() -> (w67:refnum<vi>)
      n26 = control-ref of="Basket Speed 2"() -> (w68:refnum<vi>)
      n27 = control-ref of="Tub Gallons 2"() -> (w69:refnum<vi>)
      n28 = control-ref of="Pressure 3"() -> (w70:refnum<vi>)
      n29 = control-ref of="Motor Current 2"() -> (w74:refnum<vi>)
      n30 = control-ref of="ERD 1"() -> (w73:refnum<vi>)
      n31 = control-ref of="ERD 2"() -> (w71:refnum<vi>)
      n32 = control-ref of="ERD 3"() -> (w72:refnum<vi>)
      n33 = control-ref of="All Loads"() -> (w30:refnum<vi>)
      n34 = call "Get User Filename and Path.vi"("error in (no error)"=w29) -> ("error out"=w32:errorcluster, "TXT File Path"=w38:path, "CSV File Path"=w40:path)  [unwired: 8 in]
      n35 = call "Open_Create__Log_File.vi"("File Path Control"=w40, "Enum"=enum16{"CSV File", "Text File"}."CSV File", "Error In"=w32) -> ("refnum out"=w75:refnum<file>, "File Path"=w22:path, "Error Out"=w86:errorcluster)  [unwired: 10 in]
      "CSV File Log Path" <- w22
      n36 = call "Open_Create__Log_File.vi"("File Path Control"=w38, "Enum"=enum16{"CSV File", "Text File"}."Text File", "Error In"=w32) -> ("refnum out"=w37:refnum<file>, "Error Out"=w39:errorcluster)  [unwired: 10 in, 1 out]
      n37 = Unbundle By Name(T49 {"Data"=variant, "State"=enum."Init"} ("Data")) -> ("State"=w21:T50)
      n38 = Build Array(w67, w68, w69, w70, w74, w73, w71, w72, w30) -> (w66:refnum<vi>[])
      n39 = Create User Event(user event datatype=TRUE ("Bool"), error in=w29) -> (user event=w83:refnum<user-event>, error out=w84:errorcluster)
      n40 = call "HEUI_Event_FGV.vi"("Event In"=w83, "Action"=enum16{"Get", "Set"}."Set", "Error In"=w84) -> ("Event Out"=w80:refnum<user-event>, "Error Out"=w81:errorcluster)  [unwired: 11 in]
      n41 = while "GEA2 Receive Message Loop" {
        shift-right: [w2651] -> w131
        shift-left: w29 -> [w2652]
        shift-right: [w2648] -> _
        shift-left: w124 -> [w2653]
        stop <- w2650 stop-if-true
        # "GEA2 Receive Message Loop"
        n42 = event shown="[2] \"Board Index\": Value Change" {
          selector: w2653 -> [w2666 w2671 w2686 w2692]
          dyn-events: [w2666 w2671 w2682 w2692] -> w2648
          timeout: _ -> [_ _ _ _]
          tunnel: w2652 -> [w2656 w2673 w2689 w2694]
          tunnel: [w2655 w2673 w2675 w2694] -> w2649
          tunnel: [FALSE TRUE _ TRUE] -> w2650
          event User Event {
            n43 = event-data() -> ("Source"=w2669:u8, "Destination"=w2665:u8, "Command"=w2664:u8, "Message"=w2668:string)  [unwired: 1 in]
            n44 = Bundle By Name(cluster=T12 {"Source"=0, "Destination"=0, "Command"=0, "Message"=""} ("GEA2 Data In"), "Source"=w2669, "Destination"=w2665, "Command"=w2664, "Message"=w2668) -> (w2654:T12)
            n45 = call "GEA2 Log Filter.vi"("Filter Log"="Filter Log", "Filter Data"="Filter Data", "GEA2 Msg"=w2654, "Cmd to Filter"="Cmd", "error in (no error)"=w2656) -> ("error out"=w2662:errorcluster)  [unwired: 10 in]
            n46 = call "FGV_GEA2_Ref.vi"("Action"=enum16{"Set Ref", "Get Ref"}."Get Ref", "Error In"=w2662) -> ("GEA2 Reference Out"=w2660:refnum<k24>, "Error Out"=w2661:errorcluster)  [unwired: 12 in]
            n47 = call "ACK Subscriptions Publications.vi"("GEA2 Reference In"=w2660, "GEA2 Msg"=w2654, "error in (no error)"=w2661) -> ("error out"=w2655:errorcluster)  [unwired: 11 in, 1 out]
          }
          event User Event {
            n48 = event-data() -> ()  [unwired: 1 in, 1 out]
          }
          event "Board Index": Value Change {
            # "Stop old GEA2\nbus reference"
            # "Allow other references a chance\nto begin using new reference"
            # "Store new GEA2 bus reference"
            # "Update event registration\nand initialize new GEA2 bus"
            # "Get the previous GEA2\nbus ref, but don't stop it\nuntil we update the FGV\nwith the new GEA2 ref"
            n49 = event-data() -> ("NewVal"=w2685:u8)  [unwired: 1 in]
            n50 = property on="Board Index" class="DigNum (strict)"(error in=w2689, "DisabledEnum"=T53."Disabled and Grayed Out" ("Disabled")) -> (error out=w2690:errorcluster)  [unwired: 1 in, 1 out]
            n51 = call "FGV_GEA2_Ref.vi"("Action"=enum16{"Set Ref", "Get Ref"}."Get Ref", "Error In"=w2690) -> ("GEA2 Reference Out"=w2674:refnum<k24>, "Error Out"=w2687:errorcluster)  [unwired: 12 in]
            n52 = call "GEA2_Reregister.vi"("Board Index"=w2685, "Event Registration In"=w2686, "Error In"=w2687) -> ("GEA2 Reference Out"=w2680:refnum<k24>, "Event Registration Out"=w2682:refnum<event-registration>, "Error Out"=w2683:errorcluster)  [unwired: 9 in, 1 out]
            n53 = property on="Board Index" class="DigNum (strict)"(error in=w2683, "DisabledEnum"=T53."Enabled" ("Disabled")) -> (error out=w2681:errorcluster)  [unwired: 1 in, 1 out]
            n54 = call "FGV_GEA2_Ref.vi"("GEA2 Reference In"=w2680, "Action"=enum16{"Set Ref", "Get Ref"}."Set Ref", "Error In"=w2681) -> ("Error Out"=w2677:errorcluster)  [unwired: 11 in, 1 out]
            n55 = call "Time Delay"("error in (no error)"=w2677, "Delay Time (s)"=3.0) -> ("error out"=w2676:errorcluster)  [unwired: 9 in]
            n56 = call "GEA2 Stop.vi"("GEA2 Reference In"=w2674, "Error In"=w2676) -> ("Error Out"=w2675:errorcluster)  [unwired: 13 in]
          }
          event "Stop": Value Change {
            n57 = event-data() -> ()  [unwired: 1 in, 6 out]
          }
        }
        n58 = call "Error_Control.vi"("Error In"=w2649) -> ("Error Out"=w2651:errorcluster)  [unwired: 14 in]
      }
      n59 = while "Continuous Send Loop" {
        shift-right: [w145] -> _
        shift-left: Cont_Send_States."Run" ("State") -> [w144]
        tunnel: w43 -> [w146]
        tunnel: [w139] -> _
        shift-right: [w137] -> w47
        shift-left: w29 -> [w148]
        stop <- w147 stop-if-true
        # "Continuous Send Loop"
        n60 = Dequeue Element(queue=w146, timeout in ms (-1)=0, error in (no error)=w148) -> (queue out=w140:refnum<queue>, element=w133:T46, timed out?=w141:bool, error out=w136:errorcluster)
        n61 = Select(t=w144, s=w141, f=w133) -> (s? t:f=w143:T46)
        n62 = property on="GEA2 Send" class="Clust (strict)"() -> ("Value"=w135:T12)  [unwired: 2 in, 2 out]
        n63 = case shown="\"Run\", Default" w143 {
          selector: w143 -> [w152 w167]
          tunnel: w136 -> [w154 w169]
          tunnel: [w153 w169] -> w138
          tunnel: [_ TRUE] -> w147
          tunnel: [w152 w167] -> w145
          tunnel: w140 -> [w151 w166]
          tunnel: [w151 w166] -> w139
          tunnel: w135 -> [w150 _]
          frame "Run", Default {
            n64 = case shown="False" "Start Send" {
              tunnel: w154 -> [w155 w158]
              tunnel: [w155 w162] -> w153
              tunnel: w150 -> [_ w160]
              frame False {
              }
              frame True {
                n65 = call "FGV_GEA2_Ref.vi"("Action"=enum16{"Set Ref", "Get Ref"}."Get Ref", "Error In"=w158) -> ("GEA2 Reference Out"=w156:refnum<k24>, "Error Out"=w157:errorcluster)  [unwired: 12 in]
                n66 = call "GEA2MessageFormatter.vi"("Prefix(Send/Recv)"="SEND", "GEA2 Data In"=w160, "Error In"=w157) -> ("Output String"=w161:string, "Error Out"=w165:errorcluster)  [unwired: 11 in]
                n67 = call "GExplorer_Queue_GEA2.vi"("Output String"=w161, "error in (no error)"=w165) -> ("error out"=w163:errorcluster)  [unwired: 13 in]
                n68 = call "GEA2 Send Message.vi"("GEA2 Reference In"=w156, "Input Data"=w160, "Error In"=w163) -> ("Error Out"=w162:errorcluster)  [unwired: 11 in, 1 out]
              }
            }
          }
          frame "Shutdown" {
          }
        }
        n69 = call "Error_Control.vi"("Error In"=w138) -> ("Error Out"=w137:errorcluster)  [unwired: 14 in]
        n70 = Wait (ms)(milliseconds to wait="Msg Rate (ms)") -> ()  [unwired: 1 out]
      }
      n71 = while "GEA2 Display Loop" {
        tunnel: w78 -> [w493]
        shift-right: [w491] -> _
        shift-left: _ -> [w496]
        shift-right: [w492] -> w105
        shift-left: w39 -> [w500]
        tunnel: w37 -> [w487]
        tunnel: [w485] -> w35
        stop <- w494 stop-if-true
        # "GEA2 Display Loop"
        n72 = Dequeue Element(queue=w493, error in (no error)=w500) -> (element=w499:T47, error out=w495:errorcluster)  [unwired: 1 in, 2 out]
        n73 = Unbundle By Name(w499) -> ("Data"=w497:variant, "State"=w498:enum16{"Add to Log", "Clear", "Shutdown"})
        n74 = call "Filter_GEA2_Log.vi"("GEA2 Log"=w496, "Data"=w497, "State"=w498, "error in (no error)"=w495) -> ("GEA2 Log"=w484:string, "Latest Message"=w486:string, "Shutdown"=w494:bool, "error out"=w488:errorcluster)  [unwired: 8 in]
        "GEA2 Log" <- w484
        n75 = call "Write _To_TXT_File.vi"("refnum"=w487, "text"=w486, "error in"=w488) -> ("refnum out"=w485:refnum<file>, "error out"=w489:errorcluster)  [unwired: 10 in, 1 out]
        n76 = call "Error_Control.vi"("Error In"=w489) -> ("Error Out"=w492:errorcluster)  [unwired: 14 in]
        n77 = String Subset(string=w484, length (rest)="GEA2 Log Length") -> (substring=w491:string)  [unwired: 1 in]
      }
      n78 = while "Periodic ERD Query Loop" {
        shift-right: [w196] -> w55
        shift-left: w86 -> [w198]
        tunnel: w77 -> [w199]
        shift-right: [w193] -> _
        shift-left: _ -> [w192]
        shift-right: [w186] -> _
        shift-left: _ -> [w185]
        tunnel: w75 -> [w184]
        tunnel: [w183] -> w53
        shift-right: [w182] -> _
        shift-left: T41 {"Software MC"={"Build Number"="", "Build Hash "="", "Application Version"="", "Parametric Version"="", "UI App Version"=""}, "ERD_Always Show"={"Basket Speed (RPM)"=0, "Machine State"="", "Tub Volume (Gal)"=0.0, "Pressure (inches H20)"=0.0, "Lid Switch "=FALSE, "Current RMS (Amps)"=0.0, "Cycle Selected"="", "Lid Lock Status"="", "Mode Shift Status"="", "Spray/Rinse Valve"=FALSE, "Fabric Soft Valve"=FALSE, "Drain Pump"=FALSE, "Recirc. Pump"=FALSE, "Cycle Engine State"="", "Hot  Water Valve"=FALSE, "Cold Water Valve"=FALSE, "Motor Profile"="", "Motor Profile Status"="", "Motor Mode"="", "ME Relay"=FALSE, "Cycle Count"=0, "Deep Rinse / FS"=FALSE, "My Cycle"=FALSE, "Soil Level"="", "Spin Level"="", "Stain"="", "Temp Level"="", "Load Size"="", "Delay Time"=0, "Soak Time"=0, "Deep Fill"=FALSE, "Warm Rinse"=FALSE, "Auto Soak Level"="", "Extra Rinse"=FALSE, "Wet Load Gallons"=0.0, "Target Gallons"=0.0, "Sub-Cycle"="", "Load Type"="", "Target Level (inches)"=0.0, "Valve Relay"=FALSE, "Dry Load Size"=0.0, "Shaft Speed (RPM) "=0, "MS Motor"=FALSE, "Mode Shift FB"=FALSE, "Target Bath Temp (F)"=0.0, "Temperature (F)"=0.0, "Current Bath Temp (F)"=0.0, "Lid Lock FB"="", "Lid Lock Req State"="", "Remaining Cycle Time (s)"=0, "Available Free Stack %"=0, "Child Safety"=FALSE, "Target Speed (RPM)"=0, "Reset Source"="", "Line Voltage"=0.0, "Cycle Name"="", "Bulk Disp Valve"=FALSE, "Model Number"="", "Serial Number"=""}, "Personality Set"=0, "Brass Matrix"={"Shaft Speed"=0, "Folding"=0, "Jerk"=0, "Basket Speed"=0, "Target Speed"=0, "Peak Signal"=0, " Peak Magnitude"=0.0, "Folding in Accel"=0, "Max Jerk in Accel"=0, "Max Jerk in S-S"=0, "Motor Profile Status"="", "Motor Profile"="", "OOB Redist Req"=FALSE, "OOB Detected in S-S"=FALSE, "OOB Detected in Accel"=FALSE, "Suds Abatement Req "=FALSE, "Peak Dir"=FALSE, "Peak Vector"=0.0, "S-S Points"=0, "Points"=0, "Jerk Delta"=0}, "CSV File String Arrays"={"ERD Number Array"=[], "ERD Name Array"=[], "ERD Converted String Data"=[]}, "Redundant Micro"={"Version"="", "Personality"=0, "Pressure "=0.0, "Shaft Speed"=0, "Modeshift Feedback"="", "Lid Switch"=FALSE, "Lid Lock"=FALSE, "Triac Enable"=FALSE, "Drain Pump"=FALSE, "Lid Lock Motor Speed Safety Interlock"=FALSE, "Flood Condition State"=FALSE, "Lid Open Fault State"=FALSE, "Access To Moving Parts State"=FALSE, "Heartbeat"=FALSE, "Motor Enable"=FALSE, "Lid Unlock Fault State"=FALSE}, "Algorithm Data"={"Wet Load Gal"=0.0, "Target Gallons"=0.0, "Load Type"="", "Load Size"="", "Coast Time"=0, "Ramp Time"=0, "Ramp  Speed"=0, "Ramp Avg Current"=0.0, "OOB Redist Req"=FALSE, "OOB Detected in S-S"=FALSE, "Folding in Accel"=0, "Max Jerk in Accel"=0, "Max Jerk in S-S"=0, "OOB Detected in Accel"=FALSE, "Partial Coast Time"=0, "Dry Load Size"=0.0, "Ramp Line Voltage "=0.0, "Coast Line Voltage"=0.0, "Suds Abatement Req "=FALSE}, "ATC Data"={"Current Tub Gallons"=0.0, "Hot Gallons"=0.0, "Cold Gallons"=0.0, "Target Gallons"=0.0, "Current Water Temp"=0.0, "Target Level"=0.0, "Target Bath Temp"=0.0, "Current Bath Temp "=0.0, "Cold Inlet Temp"=0.0, "Hot Inlet Temp"=0.0, "Warm Inlet Temp"=0.0, "Hot Seg Valve Time"=0, "Cold Seg Valve Time "=0, "User Temp Level"="", "Segment Gallons"=0.0}, "Fault Table Array "=[], "RJ45"={"Write Access Actual"="", "Write Access Request"="", "LockedAtLeastOnce"=""}, "Commercial_Laundry"={"Session"="", "Phase"="", "Appliance Type"="", "Cycle Selected"="", "Platform Type"="", "Retry Signal"="", "Session Ext"="", "Phase Ext"="", "Appliance Type Ext"="", "Cycle Selected Ext"="", "Platform Type Ext"="", "Retry Signal Ext"=""}, "Boot Loader Version"={"UI BL Version"="", "MC BL Version"=""}} ("All_Bundled_Data_Brass Out") -> [w181]
        tunnel: w66 -> [w180]
        shift-right: [w178] -> _
        shift-left: _ -> [w177]
        shift-right: [w174] -> _
        shift-left: _ -> [w173]
        shift-right: [w171] -> _
        shift-left: w21 -> [w170]
        i -> [w179]
        stop <- w195 stop-if-true
        # "ERD Loop"
        n79 = Dequeue Element(queue=w199, timeout in ms (-1)=0, error in (no error)=w198) -> (element=w187:T49, timed out?=w190:bool, error out=w197:errorcluster)  [unwired: 1 out]
        n80 = Unbundle By Name(w187) -> ("State"=w189:T50)
        n81 = call "FGV_GEA2_Ref.vi"("Action"=enum16{"Set Ref", "Get Ref"}."Get Ref", "Error In"=w197) -> ("GEA2 Reference Out"=w176:refnum<k24>, "Error Out"=w175:errorcluster)  [unwired: 12 in]
        n82 = Select(t=w170, s=w190, f=w189) -> (s? t:f=w172:T50)
        n83 = case shown="\"Get Version\"" w172 {
          tunnel: w175 -> [w206 w255 w276 w297 w316 w338 w382 w433 w455 w465 w483]
          tunnel: [w208 w239 w266 w289 w316 w336 w381 w430 w455 w465 w483] -> w194
          tunnel: [_ _ _ _ _ _ _ _ _ _ TRUE] -> w195
          tunnel: [w214 w253 w274 w291 w319 w342 w375 w439 w464 w473 w481] -> w193
          tunnel: w192 -> [w214 w253 w274 w304 w319 w342 w375 w439 w464 w473 w481]
          tunnel: "GEA Inputs 2" -> [_ w237 _ w285 _ _ w379 _ _ _ _]
          tunnel: [ERD_Loop_States."Get Version" ("State") ERD_Loop_States."Build ERD Read List" ("State") ERD_Loop_States."Read ERDs" ("State") ERD_Loop_States."Update UI" ("State") ERD_Loop_States."Update Graphs" ("State") ERD_Loop_States."Read Faults" ("State") ERD_Loop_States."Log Data" ("State") ERD_Loop_States."Pause" ("State") ERD_Loop_States."Read ERDs" ("State") ERD_Loop_States."Log Data" ("State") ERD_Loop_States."Shutdown" ("State")] -> w171
          tunnel: w176 -> [_ w254 _ w283 _ w331 w380 _ _ _ _]
          tunnel: [w213 w250 w275 w284 w321 w340 w376 w438 w463 w469 w479] -> w186
          tunnel: w185 -> [w213 w250 _ w284 w321 w340 w376 w438 w463 w469 w479]
          tunnel: w184 -> [w212 w249 w272 w296 w317 w339 w374 w415 w462 w470 w478]
          tunnel: [w212 w249 w272 w296 w317 w339 w374 w437 w462 w470 w478] -> w183
          tunnel: [w211 w234 w271 w292 w318 w330 w377 w416 w461 w471 w477] -> w182
          tunnel: w181 -> [w211 w222 w271 w278 w318 w327 w378 w416 w461 w471 w477]
          tunnel: w180 -> [_ _ _ _ _ w332 _ _ _ _ _]
          tunnel: w179 -> [_ _ _ _ _ _ _ w420 _ _ _]
          tunnel: [w207 w248 w270 w290 w313 w328 w371 w419 w460 w472 w476] -> w178
          tunnel: w177 -> [w207 w248 w270 w290 w313 w328 w371 w418 w460 w472 w476]
          tunnel: [w202 w232 w268 w277 w306 w324 w369 w410 w457 w467 w474] -> w174
          tunnel: w173 -> [w202 _ _ w277 w306 w324 w369 w410 w457 w467 w474]
          frame "Init", Default {
            # "Set Write Header\nFGV to True"
            n84 = call "Time Delay10"("error in (no error)"=w206, "Delay Time (s)"=4.0) -> ("error out"=w205:errorcluster)  [unwired: 9 in]
            n85 = call "Write_Header_FGV.vi"("Write Header ? In"=TRUE, "Action"=enum16{"Get", "Set"}."Set", "Error In"=w205) -> ("Error Out"=w208:errorcluster)  [unwired: 11 in, 1 out]
            "String" <- "Initializate" ("String")
          }
          frame "Get Version" {
            w232 = string[] ["Erd_GitHash", "Erd_BuildNumber", "Erd_ApplicationVersion", "Erd_ParametricVersion"] ("ERD Name")
            # "1. Enable Brass Matrix\n2. Exit Low Power Mode"
            n86 = call "GEA2 Write ERD.vi"("GEA2 Reference In"=w254, "GEA Inputs"=w237, "Write ERD List"=T52[] [{"ERD Number"=61628, "Data Type"=enum."string", "Data"="01 00 00 00 00 00 00 00 00 00 00 00 00 00 00 00 00 00 00 00"}, {"ERD Number"=61479, "Data Type"=enum."string", "Data"="01"}], "Error In"=w255, "Verify ERD Response?"=FALSE) -> ("GEA2 Reference Out"=w225:refnum<k24>, "Error Out"=w224:errorcluster)  [unwired: 8 in, 1 out]
            n87 = call "GEA3 Read ERD (Rev 2 API) Multiple Messages.vi"("GEA2 Reference In"=w225, "Retry Count"=1 ("# of Iterations (Should be 2 except JL)"), "Read Timeout (ms)"=u32 250, "GEA Inputs"=cluster{"Source":u8, "Destination":u8} {"Source"=229, "Destination"=37}, "Read ERD List"=T9[] [{"ERD Number"=57, "Data Type"=enum."string"}, {"ERD Number"=58, "Data Type"=enum."string"}] ("Read ERD List MC"), "Error In"=w224, "Verify ERD Response?"=FALSE) -> ("GEA2 Reference Out"=w220:refnum<k24>, "ERD Data Out"=w223:cluster{"ERD Number":u16, "Data":string}[], "Error Out"=w215:errorcluster)  [unwired: 5 in, 1 out]
            n88 = call "Convert_UI_Laundry_ERD.vi"("All_ERD_Data_Bundled_Brass In"=w222, "Array"=w223, "Error In"=w215) -> ("All_ERD_Data_Bundled_Brass"=w221:T41, "Error Out"=w218:errorcluster)  [unwired: 11 in]
            n89 = case shown="False" TRUE {
              tunnel: [w257 w260] -> w219
              tunnel: w220 -> [w257 w260]
              tunnel: w218 -> [w256 w258]
              tunnel: [w256 w258] -> w217
              frame False {
              }
              frame True {
                n90 = Wait Until Next ms Multiple(millisecond multiple=u32 100) -> ()  [unwired: 1 out]
              }
            }
            n91 = local write "String"("Exit" ("String")) -> ()
            n92 = call "GEA2 Send and Receive Message.vi"("GEA2 Reference In"=w219, "Input Data"=T12 {"Source"=229, "Destination"=192, "Command"=1, "Message"=""}, "Expected Command"="01", "Expected Source"="C0", "Error In"=w217) -> ("GEA2 Reference Out"=w238:refnum<k24>, "Converted Data Out"=w243:T57, "Error Out"=w242:errorcluster)  [unwired: 7 in, 1 out]
            n93 = call "Version_Parse.vi"("All_ERD_Data_Bundled_Brass in"=w221, "Converted Data Out"=w243, "Error In"=w242) -> ("All_ERD_Data_Bundled_Brass out"=w235:T41, "Error Out"=w241:errorcluster)  [unwired: 11 in]
            n94 = call "GEA3 Read ERD (Rev 2 API) Multiple Messages.vi"("GEA2 Reference In"=w238, "GEA Inputs"=w237, "Read ERD List"=cluster{"ERD Number":u16, "Data Type":T7}[] [{"ERD Number"=127, "Data Type"=enum."string"}, {"ERD Number"=49, "Data Type"=enum."string"}, {"ERD Number"=58, "Data Type"=enum."string"}, {"ERD Number"=59, "Data Type"=enum."string"}], "Error In"=w241) -> ("ERD Data Out"=w233:cluster{"ERD Number":u16, "Data":string}[], "Error Out"=w240:errorcluster)  [unwired: 8 in, 2 out]
            n95 = call "Convert_ERDs.vi"("ERD Name"=w232, "All_ERD_Data_Bundled_Brass In"=w235, "Array"=w233, "Error In"=w240) -> ("All_ERD_Data_Bundled_Brass"=w234:T41, "Error Out"=w239:errorcluster)  [unwired: 10 in]
          }
          frame "Build ERD Read List" {
            n96 = Build Array (concatenate)("Basic ERDs", "ERD always show") -> (w261:T39)
            n97 = call "ERD_Read_List_Builder.vi"("Array"=w261, "Error In"=w276) -> ("Read ERD List"=w275:T9[], "ERD Name"=w268:string[], "Error Out"=w267:errorcluster)  [unwired: 15 in]
            n98 = local write "String"("Build ERD Read List" ("String")) -> ()
            n99 = call "Write_Header_FGV.vi"("Write Header ? In"=TRUE, "Action"=enum16{"Get", "Set"}."Set", "Error In"=w267) -> ("Error Out"=w266:errorcluster)  [unwired: 11 in, 1 out]
          }
          frame "Read ERDs" {
            n100 = call "Convert Read ERD List to Message.vi"("GEA Inputs"=w285, "Read ERD List"=w284, "Error In"=w297) -> ("GEA Message"=w301:T12, "Error Out"=w302:errorcluster)  [unwired: 11 in]
            n101 = call "GEA2MessageFormatter.vi"("Prefix(Send/Recv)"="SEND", "GEA2 Data In"=w301, "Error In"=w302) -> ("Output String"=w300:string, "Error Out"=w299:errorcluster)  [unwired: 11 in]
            n102 = call "GExplorer_Queue_GEA2.vi"("Output String"=w300, "error in (no error)"=w299) -> ("error out"=w282:errorcluster)  [unwired: 13 in]
            n103 = Tick Count (ms)() -> (millisecond timer value=w291:u32)
            n104 = Subtract(x=w291, y=w304) -> (x-y=→"Log Rate (ms)":u32)
            n105 = call "GEA3 Read ERD (Rev 2 API) Multiple Messages.vi"("GEA2 Reference In"=w283, "Retry Count"=1, "Read Timeout (ms)"=u32 200, "GEA Inputs"=w285, "Read ERD List"=w284, "Error In"=w282, "Verify ERD Response?"=FALSE) -> ("ERD Data Out"=w287:cluster{"ERD Number":u16, "Data":string}[], "Error Out"=w286:errorcluster)  [unwired: 5 in, 2 out]
            n106 = local write "String"("Read ERDS" ("String")) -> ()
            n107 = call "Write_Header_FGV.vi"("Action"=enum16{"Get", "Set"}."Get", "Error In"=w286) -> ("Write Header ? Out"=w293:bool, "Error Out"=w295:errorcluster)  [unwired: 12 in]
            n108 = call "Convert_ERDs.vi"("New Header?"=w293, "ERD Name"=w277, "All_ERD_Data_Bundled_Brass In"=w278, "Array"=w287, "Error In"=w295) -> ("All_ERD_Data_Bundled_Brass"=w292:T41, "Error Out"=w289:errorcluster)  [unwired: 9 in]
          }
          frame "Update UI" {
            n109 = Unbundle By Name(w318) -> ("Software MC"=→"Application Version":T6, "Personality Set"=→"Personality Set":u8, "ERD_Always Show"=→"ERD_Always Show":T1, "Redundant Micro"=→"Redundant Micro":T35, "Algorithm Data"=→"Algorithm Data":T36, "ATC Data"=→"ATC Data":T37, "RJ45"=→"RJ45":T3, "Commercial_Laundry"=→"Commercial_Laundry":T4, "Boot Loader Version"=→"Boot Loader Version":T5)  [unwired: 1 out]
            n110 = local write "String"("Update UI" ("String")) -> ()
          }
          frame "Update Graphs" {
            n111 = case shown="True" "ERD Graphing ON" {
              tunnel: w338 -> [w361 w368]
              tunnel: [w361 w367] -> w337
              tunnel: "ERD Graph Cntrl" -> [_ w366]
              tunnel: [_ w365] -> w333
              tunnel: w331 -> [_ w364]
              tunnel: w327 -> [w360 w363]
              tunnel: [w360 w362] -> w326
              frame False {
              }
              frame True {
                n112 = call "Graph ERD Read List.vi"("GEA2 Reference In"=w364, "All_Bundled_Data_In"=w363, "ERD Graph Cntrl"=w366, "Error In"=w368) -> ("ERD Graph  Ind"=w365:T15, "All_Bundled_Data_Brass Out"=w362:T41, "Error Out"=w367:errorcluster)  [unwired: 8 in, 1 out]
              }
            }
            n113 = case shown="True" "Graphing ON" {
              tunnel: w337 -> [w343 w359]
              tunnel: [w343 w358] -> w336
              tunnel: w333 -> [_ w356]
              tunnel: w332 -> [_ w355]
              tunnel: w326 -> [w344 w346]
              tunnel: [w344 w346] -> w330
              frame False {
              }
              frame True {
                n114 = call "Update Graphs.vi"("Select Graph"="Select Graph", "appended array"=w355, "ERD Graph  Ind 2"=w356, "ERD_Data_Bundled_In"=w346, "Error In"=w359) -> ("All Loads"=→"All Loads":u16[][], "Water Temperature"=→"Temp 2":dbl, "Basket Speed"=→"Basket Speed 2":u16[][], "Tub Gallons"=→"Tub Gallons 2":dbl, "Pressure"=→"Pressure 3":dbl, "Motor Current"=→"Motor Current 2":dbl, "ERD 3"=→"ERD 3":dbl, "ERD 2"=→"ERD 2":dbl, "ERD 1"=→"ERD 1":dbl, "Error Out"=w358:errorcluster)  [unwired: 1 in]
                "ERD Graph  Ind" <- w356
              }
            }
            n115 = local write "String"("Update Graphs" ("String")) -> ()
          }
          frame "Read Faults" {
            n116 = case shown="True" "Fault ON" {
              tunnel: w382 -> [w383 w393]
              tunnel: [w383 w392] -> w381
              tunnel: w380 -> [_ w390]
              tunnel: w379 -> [_ w389]
              tunnel: w378 -> [w384 w396]
              tunnel: [w384 w395] -> w377
              frame False {
              }
              frame True {
                # "0-9 Sequence\n10-21 Table"
                n117 = call "GEA3 Read ERD (Rev 2 API) Multiple Messages.vi"("GEA2 Reference In"=w390, "Retry Count"=2, "Read Timeout (ms)"=u32 100, "GEA Inputs"=w389, "Read ERD List"=T9[] [{"ERD Number"=57615, "Data Type"=enum."string"}, {"ERD Number"=141, "Data Type"=enum."uint32_t"}, {"ERD Number"=57617, "Data Type"=enum."string"}, {"ERD Number"=57618, "Data Type"=enum."string"}, {"ERD Number"=57619, "Data Type"=enum."string"}, {"ERD Number"=57620, "Data Type"=enum."string"}, {"ERD Number"=57621, "Data Type"=enum."string"}, {"ERD Number"=57622, "Data Type"=enum."string"}, {"ERD Number"=57623, "Data Type"=enum."string"}, {"ERD Number"=57624, "Data Type"=enum."string"}, {"ERD Number"=57603, "Data Type"=enum."string"}, {"ERD Number"=57605, "Data Type"=enum."string"}, {"ERD Number"=57606, "Data Type"=enum."string"}, {"ERD Number"=57607, "Data Type"=enum."string"}, {"ERD Number"=57608, "Data Type"=enum."string"}, {"ERD Number"=57609, "Data Type"=enum."string"}, {"ERD Number"=57610, "Data Type"=enum."string"}, {"ERD Number"=57611, "Data Type"=enum."string"}, {"ERD Number"=57612, "Data Type"=enum."string"}, {"ERD Number"=57613, "Data Type"=enum."string"}, {"ERD Number"=57614, "Data Type"=enum."string"}], "Error In"=w393, "Verify ERD Response?"=FALSE) -> ("ERD Data Out"=w391:cluster{"ERD Number":u16, "Data":string}[], "Error Out"=w392:errorcluster)  [unwired: 5 in, 2 out]
                n118 = Array Subset(array=w391, index=10, length=11) -> (w399:cluster{"ERD Number":u16, "Data":string}[])
                n119 = Array Subset(array=w391, index=0, length=10) -> (w398:cluster{"ERD Number":u16, "Data":string}[])
                n120 = call "Fault_Table_Read.vi"("ERD Data Out"=w399) -> ("Fault Set?"=→"Fault Status":bool, "Table Buffer Status"=→"Table Buffer Status":T20, "Fault Table String Out"=→"Fault Table Buffer":string[][], "Fault Table Array Out"=w394:T44)  [unwired: 11 in]
                n121 = call "Fault_Seq_Read.vi"("Seq ERD In"=w398) -> ("Seq Buffer Status"=→"Seq Buffer Status":T20, "String"=→"Fault Sequence Buffer":string)  [unwired: 13 in]
                n122 = Bundle By Name(cluster=w396, "Fault Table Array"=w394) -> (w395:T41)
              }
            }
            n123 = local write "String"("Read Faults" ("String")) -> ()
          }
          frame "Log Data" {
            # "TimeStamp"
            # "Every 2000th iteration return\nto init to exit test mode"
            # "Append With Fault Log Data"
            # "Write Date/Time Header"
            n124 = Unbundle By Name(w416) -> ("CSV File String Arrays.ERD Name Array"=w436:string[], "CSV File String Arrays.ERD Number Array"=w435:string[], "CSV File String Arrays.ERD Converted String Data"=w428:string[])
            n125 = Quotient & Remainder(x=w420, y=2000) -> (floor(x/y)=w419:i32)  [unwired: 1 out]
            n126 = Greater?(x=w419, y=w418) -> ()  [unwired: 1 out]
            n127 = call "Write_Header_FGV.vi"("Action"=enum16{"Get", "Set"}."Get", "Error In"=w433) -> ("Write Header ? Out"=w417:bool, "Error Out"=w427:errorcluster)  [unwired: 12 in]
            n128 = case shown="True" w417 {
              tunnel: w436 -> [w448 _]
              tunnel: w435 -> [w447 _]
              tunnel: w416 -> [w446 _]
              tunnel: [w441 w454] -> w414
              tunnel: w415 -> [w440 w454]
              frame True {
                n129 = call "Build_Header.vi"("All_Bundled_Data_Brass Out"=w446, "ERD Number Array In"=w447, "ERD Name Array In"=w448) -> ("ERD Name Array out 2"=w445:string[][])  [unwired: 8 in]
                n130 = Array Size(array=w445) -> (size(s)=w444:i32[])
                n131 = Index Array(array=w444, index=1) -> (element=w442:i32)
                n132 = for {
                  N: w442 -> [_]
                  tunnel: w445 -> [w453]
                  tunnel: [w451] -> w441
                  tunnel: w440 -> [w450]
                  i -> [w452]
                  n133 = Index Array(array=w453, index (row)=w452) -> (element=w449:string[])  [unwired: 1 in]
                  n134 = call "Write _To_CSV_File.vi"("Refnum In"=w450, "String Array 1"=w449) -> ("Refnum Out"=w451:refnum<file>)  [unwired: 15 in, 2 out]
                }
              }
              frame False {
              }
            }
            n135 = call "TimeStamp to String Array.vi"("String Array In"=w428) -> ("String Array Out"=w426:string[])  [unwired: 10 in]
            n136 = Unbundle By Name(w416) -> ("Fault Table Array"=w422:T44)
            n137 = call "Faults_To_String_Array.vi"("Write Header ?"=w417, "Fault Table Entry"=w422, "Error In"=w427) -> ("Fault Header String Array"=w413:string[], "Fault ERD Number String Array"=w412:string[], "Fault Data String Array"=w425:string[], "Error Out"=w423:errorcluster)  [unwired: 13 in]
            n138 = local read "Boolean"() -> (w409:bool)
            n139 = Insert Into Array(array=w426, new element=w425) -> (w424:string[])  [unwired: 1 in]
            n140 = Not(x=w409) -> (.not. x?=→"Boolean":bool)
            n141 = call "Write _To_CSV_File.vi"("Refnum In"=w414, "String Array 1"=w413, "String Array 2"=w412, "String Array 3"=w424, "Error In"=w423) -> ("Refnum Out"=w437:refnum<file>, "Error Out"=w431:errorcluster)  [unwired: 12 in, 1 out]
            n142 = call "Write_Header_FGV.vi"("Write Header ? In"=FALSE, "Action"=enum16{"Get", "Set"}."Set", "Error In"=w431) -> ("Error Out"=w430:errorcluster)  [unwired: 11 in, 1 out]
          }
          frame "Pause" {
            n143 = Wait Until Next ms Multiple(millisecond multiple="Rate") -> ()  [unwired: 1 out]
            n144 = local write "String"("Pause" ("String")) -> ()
          }
          frame "Brass Logging" {
            n145 = local write "String"("Brass Logging" ("String")) -> ()
          }
          frame "Shutdown" {
            n146 = local write "String"("Shutdown" ("String")) -> ()
          }
        }
        n147 = call "Error_Control.vi"("Error In"=w194) -> ("Error Out"=w196:errorcluster)  [unwired: 14 in]
      }
      n148 = while "UI Loop" {
        shift-right: [w1099] -> w130
        shift-left: w81 -> [w1093]
        shift-right: [w1101] -> w129
        shift-left: _ -> [_]
        tunnel: w106 -> [w1100]
        tunnel: w80 -> [w1091]
        tunnel: w77 -> [w1090]
        tunnel: w22 -> [w1089]
        stop <- w1098 stop-if-true
        # "UI Loop"
        n149 = call "FGV_GEA2_Ref.vi"("Action"=enum16{"Set Ref", "Get Ref"}."Get Ref", "Error In"=w1093) -> ("GEA2 Reference Out"=w1088:refnum<k24>, "Error Out"=w1094:errorcluster)  [unwired: 12 in]
        n150 = event shown="[8] \"Programming.Program\": Value Change" {
          selector: w1100 -> [_ _ _ _ _ _ _ _ _ _ _ _ _ _ _ _ _ _ _ _ _ _ _ _ _ _ _ _ _ _ _ _ _ _ _ _ _ _ _ _ _ _ _ _ _ _ _ _ _ _ _]
          dyn-events: _ -> [_ _ _ _ _ _ _ _ _ _ _ _ _ _ _ _ _ _ _ _ _ _ _ _ _ _ _ _ _ _ _ _ _ _ _ _ _ _ _ _ _ _ _ _ _ _ _ _ _ _ _]
          timeout: 100 -> [_ _ _ _ _ _ _ _ _ _ _ _ _ _ _ _ _ _ _ _ _ _ _ _ _ _ _ _ _ _ _ _ _ _ _ _ _ _ _ _ _ _ _ _ _ _ _ _ _ _ _]
          tunnel: [w1107 w1117 w1119 w1139 w1146 w1161 w1174 w1192 w1209 w1251 w1265 w1272 w1291 w1305 w1369 w1444 w1488 w1551 w1675 w1740 w1801 w1922 w1992 w2049 w2085 w2201 w2217 w2228 w2242 w2253 w2265 w2298 w2321 w2331 w2353 w2376 w2397 w2408 w2427 w2463 w2469 w2519 w2526 w2531 _ w2574 w2585 w2596 w2606 w2614 w2639] -> w1097
          tunnel: w1094 -> [w1104 w1114 w1125 w1139 w1148 w1165 w1173 w1189 w1219 w1257 w1266 w1288 w1295 w1304 w1368 w1441 w1496 w1555 w1673 w1738 w1803 w1924 w1996 w2052 w2088 w2203 w2215 w2225 w2243 w2255 w2266 w2304 w2324 w2336 w2359 w2379 w2398 w2415 w2434 w2465 w2476 w2521 w2528 w2536 w2542 w2582 w2588 w2600 w2609 w2620 w2646]
          tunnel: [_ _ _ _ _ _ _ _ _ _ _ _ _ _ _ _ _ _ _ _ _ _ _ _ _ _ _ _ _ _ _ _ _ _ _ _ _ TRUE _ _ _ _ _ _ _ _ _ _ _ _ _] -> w1098
          tunnel: w1088 -> [w1102 w1116 w1124 w1140 w1145 w1158 _ _ w1220 w1256 w1264 w1287 _ w1301 w1365 w1453 w1490 w1553 w1677 w1742 w1804 w1925 w1997 w2053 w2089 w2200 _ w2224 w2238 w2249 w2264 w2303 w2317 w2335 w2349 w2367 _ w2418 w2424 w2466 w2477 w2520 w2529 w2533 w2543 w2584 w2589 w2599 w2610 w2621 w2647]
          tunnel: [w1109 w1116 _ w1140 w1147 w1157 _ _ _ _ w1263 w1275 _ w1300 w1364 _ w1489 w1552 w1676 w1741 w1800 w1921 w1993 w2050 w2086 w2202 _ _ w2237 w2254 _ _ _ _ _ w2371 _ w2418 w2420 w2464 w2470 w2518 w2527 w2532 _ w2575 w2586 w2597 w2607 w2615 w2640] -> w1101
          tunnel: "GEA Inputs" -> [_ _ w1123 _ w1143 w1159 _ _ w1206 _ _ w1277 _ w1302 w1366 _ w1491 w1554 w1678 w1743 w1805 w1926 w1998 w2054 w2090 w2199 _ w2220 w2239 w2250 _ w2301 w2312 w2337 w2350 w2366 _ _ w2423 _ w2468 _ _ w2534 _ w2577 w2587 w2598 w2608 w2617 w2634]
          tunnel: w1091 -> [_ _ _ _ _ _ _ _ w1216 _ _ _ _ _ _ w1438 _ _ _ _ _ _ _ _ _ _ _ _ _ _ _ _ _ _ _ _ _ _ _ _ _ _ _ _ _ _ _ _ _ _ _]
          tunnel: w1090 -> [_ _ w1118 _ _ _ _ _ w1210 w1250 _ w1285 _ _ _ w1439 _ _ _ _ _ _ _ _ _ _ w2213 _ _ _ _ _ _ _ _ _ w2395 _ _ _ _ _ _ _ _ _ _ _ _ _ _]
          tunnel: w1089 -> [_ _ _ _ _ _ _ _ _ _ _ _ _ _ _ _ _ _ _ _ _ _ _ _ _ _ _ w2219 _ _ _ _ _ _ _ _ _ _ _ _ _ _ _ _ _ _ _ _ _ _ _]
          event "Send Button": Value Change {
            n151 = event-data() -> ()  [unwired: 1 in, 1 out]
            n152 = call "GEA2MessageFormatter.vi"("Prefix(Send/Recv)"="SEND", "GEA2 Data In"="GEA2 Send", "Error In"=w1104) -> ("Output String"=w1106:string, "Error Out"=w1105:errorcluster)  [unwired: 11 in]
            n153 = call "GExplorer_Queue_GEA2.vi"("Output String"=w1106, "error in (no error)"=w1105) -> ("error out"=w1108:errorcluster)  [unwired: 13 in]
            n154 = call "GEA2 Send Message.vi"("GEA2 Reference In"=w1102, "Input Data"="GEA2 Send", "Error In"=w1108) -> ("GEA2 Reference Out"=w1109:refnum<k24>, "Error Out"=w1107:errorcluster)  [unwired: 11 in]
          }
          event "Clear": Value Change {
            w1111 = T47 {"Data"=variant, "State"=enum."Clear"} ("element")
            n155 = event-data() -> ()  [unwired: 1 in, 6 out]
            n156 = Obtain Queue(name (unnamed)="GEA2", element data type=w1111, error in (no error)=w1114) -> (queue out=w1112:refnum<queue>, error out=w1115:errorcluster)  [unwired: 2 in, 1 out]
            n157 = Enqueue Element(queue=w1112, element=w1111, error in (no error)=w1115) -> (error out=w1117:errorcluster)  [unwired: 1 in, 2 out]
          }
          event "Set Personality": Value Change {
            n158 = event-data() -> ()  [unwired: 1 in, 6 out]
            n159 = Index Array(array=T52[] [{"ERD Number"=65280, "Data Type"=enum."string", "Data"=""}] ("Write ERD List")) -> (element=w1130:T52)  [unwired: 1 in]
            n160 = Number To Hexadecimal String(1:i16 2 ("width (-)"), 2:"?") -> (0:w1129:string)
            n161 = Bundle By Name(cluster=w1130, "Data"=w1129) -> (w1128:T52)
            n162 = Build Array(w1128) -> (w1127:T52[])
            n163 = call "Convert Write ERD List to Message.vi"("GEA Inputs"=w1123, "Write ERD List"=w1127, "Error In"=w1125) -> ("GEA Message"=w1135:T12, "Error Out"=w1136:errorcluster)  [unwired: 11 in]
            n164 = call "GEA2MessageFormatter.vi"("Prefix(Send/Recv)"="SEND", "GEA2 Data In"=w1135, "Error In"=w1136) -> ("Output String"=w1137:string, "Error Out"=w1138:errorcluster)  [unwired: 11 in]
            n165 = call "GExplorer_Queue_GEA2.vi"("Output String"=w1137, "error in (no error)"=w1138) -> ("error out"=w1133:errorcluster)  [unwired: 13 in]
            n166 = call "GEA2 Write ERD.vi"("GEA2 Reference In"=w1124, "GEA Inputs"=w1123, "Write ERD List"=w1127, "Error In"=w1133, "Verify ERD Response?"=FALSE) -> ("Error Out"=w1120:errorcluster)  [unwired: 8 in, 2 out]
            n167 = Enqueue Element(queue=w1118, element=T49 {"Data"=variant, "State"=enum."Init"} ("Data"), error in (no error)=w1120) -> (error out=w1119:errorcluster)  [unwired: 1 in, 2 out]
          }
          event Timeout {
            # "Must have timeout case to give GEA2 FGV a chance to update\nthe GEA2 reference. Otherwise, when we receive an event it may\nbe using a reference that is no longer valid."
            n168 = event-data() -> ()  [unwired: 1 in, 3 out]
          }
          event "Write ERD": Value Change {
            n169 = event-data() -> ()  [unwired: 1 in, 1 out]
            n170 = call "Convert Write ERD List to Message.vi"("GEA Inputs"=w1143, "Write ERD List"="Write ERD List", "Error In"=w1148) -> ("GEA Message"=w1150:T12, "Error Out"=w1151:errorcluster)  [unwired: 11 in]
            n171 = call "GEA2MessageFormatter.vi"("Prefix(Send/Recv)"="SEND", "GEA2 Data In"=w1150, "Error In"=w1151) -> ("Output String"=w1152:string, "Error Out"=w1153:errorcluster)  [unwired: 11 in]
            n172 = call "GExplorer_Queue_GEA2.vi"("Output String"=w1152, "error in (no error)"=w1153) -> ("error out"=w1142:errorcluster)  [unwired: 13 in]
            n173 = call "GEA3 Write ERD (Rev 2 API) Multiple Messages.vi"("GEA2 Reference In"=w1145, "GEA Inputs"=w1143, "Write ERD List"="Write ERD List", "Error In"=w1142, "Verify ERD Response?"=FALSE) -> ("GEA2 Reference Out"=w1147:refnum<k24>, "Error Out"=w1146:errorcluster)  [unwired: 8 in, 1 out]
          }
          event "Read ERD": Value Change {
            n174 = event-data() -> ()  [unwired: 1 in, 6 out]
            n175 = call "Convert Read ERD List to Message.vi"("GEA Inputs"=w1159, "Read ERD List"="Read ERD List", "Error In"=w1165) -> ("GEA Message"=w1169:T12, "Error Out"=w1164:errorcluster)  [unwired: 11 in]
            n176 = call "GEA2MessageFormatter.vi"("Prefix(Send/Recv)"="SEND", "GEA2 Data In"=w1169, "Error In"=w1164) -> ("Output String"=w1167:string, "Error Out"=w1166:errorcluster)  [unwired: 11 in]
            n177 = call "GExplorer_Queue_GEA2.vi"("Output String"=w1167, "error in (no error)"=w1166) -> ("error out"=w1162:errorcluster)  [unwired: 13 in]
            n178 = call "GEA3 Read ERD (Rev 2 API) Multiple Messages.vi"("GEA2 Reference In"=w1158, "Retry Count"=2, "Read Timeout (ms)"=u32 200, "GEA Inputs"=w1159, "Read ERD List"="Read ERD List", "Error In"=w1162, "Verify ERD Response?"=FALSE) -> ("GEA2 Reference Out"=w1157:refnum<k24>, "ERD Data Out"=→"Read ERD Data Out":cluster{"ERD Number":u16, "Data":string}[], "Error Out"=w1161:errorcluster)  [unwired: 5 in, 1 out]
          }
          event "HEUI Launch": Value Change {
            n179 = event-data() -> ()  [unwired: 1 in, 6 out]
            n180 = call "HEUI_Running_FGV.vi"("Action"=enum16{"Get", "Set"}."Get", "Error In"=w1173) -> ("Running?"=w1170:bool, "Error Out"=w1172:errorcluster)  [unwired: 12 in]
            n181 = case shown="False" w1170 {
              tunnel: w1172 -> [w1180 w1187]
              tunnel: [w1179 w1187] -> w1174
              frame False {
                w1186 = 128  # options
                n182 = Current VI's Path() -> (path=w1178:path)
                n183 = Strip Path(path=w1178) -> (stripped path=w1177:path)  [unwired: 1 out]
                n184 = Build Path(base path=w1177, name or relative path="HEUI.vi") -> (appended path=w1175:path)
                n185 = Open VI Reference(type specifier VI Refnum (for type only)=refnum<vi> refnum ("reference"), vi path=w1175, options=w1186, error in (no error)=w1180) -> (vi reference=w1183:refnum<vi>, error out=w1185:errorcluster)  [unwired: 2 in]
                n186 = call-by-ref "Start Asynchronous Call"(reference=w1183, error in=w1185) -> (reference out=w1181:refnum<vi>, error out=w1182:errorcluster)  [unwired: 14 in, 2 out]
                n187 = Close Reference(reference=w1181, error in (no error)=w1182) -> (error out=w1179:errorcluster)
              }
              frame True {
              }
            }
          }
          event "LEUI Launch": Value Change {
            n188 = event-data() -> ()  [unwired: 1 in, 6 out]
            n189 = call "HEUI_Running_FGV.vi"("Action"=enum16{"Get", "Set"}."Get", "Error In"=w1189) -> ("Running?"=w1188:bool, "Error Out"=w1190:errorcluster)  [unwired: 12 in]
            n190 = case shown="False" w1188 {
              tunnel: w1190 -> [w1198 w1205]
              tunnel: [w1197 w1205] -> w1192
              frame False {
                w1204 = 128  # options
                n191 = Current VI's Path() -> (path=w1196:path)
                n192 = Strip Path(path=w1196) -> (stripped path=w1195:path)  [unwired: 1 out]
                n193 = Build Path(base path=w1195, name or relative path="LEUI.vi") -> (appended path=w1193:path)
                n194 = Open VI Reference(type specifier VI Refnum (for type only)=refnum<vi> refnum ("reference"), vi path=w1193, options=w1204, error in (no error)=w1198) -> (vi reference=w1201:refnum<vi>, error out=w1203:errorcluster)  [unwired: 2 in]
                n195 = call-by-ref "Start Asynchronous Call"(reference=w1201, error in=w1203) -> (reference out=w1199:refnum<vi>, error out=w1200:errorcluster)  [unwired: 15 in, 1 out]
                n196 = Close Reference(reference=w1199, error in (no error)=w1200) -> (error out=w1197:errorcluster)
              }
              frame True {
              }
            }
          }
          event Value Change {
            (unwired) "ERD Loop" ("name (unnamed)")
            w1212 = TRUE ("Blinking")
            (unwired) FALSE ("Data On")
            n197 = event-data() -> ()  [unwired: 1 in, 6 out]
            n198 = Generate User Event(user event=w1216, event data cluster=TRUE ("event data"), error in=w1219) -> (error out=w1217:errorcluster)  [unwired: 1 in, 1 out]
            n199 = property on="Program Ind" class="Bool (strict)"(error in=w1217, "Value"=w1212, "Blinking"=w1212) -> (error out=w1213:errorcluster)  [unwired: 1 in, 1 out]
            n200 = Enqueue Element(queue=w1210, element=T49 {"Data"=variant, "State"=enum."Pause"} ("Data"), error in (no error)=w1213) -> (error out=w1215:errorcluster)  [unwired: 1 in, 2 out]
            n201 = call "Time Delay3"("error in (no error)"=w1215, "Delay Time (s)"=2.0) -> ("error out"=w1214:errorcluster)  [unwired: 9 in]
            n202 = Unbundle By Name("Programming") -> ("File Path"=w1223:path)
            n203 = call "GEA2 Write ERD.vi"("GEA2 Reference In"=w1220, "GEA Inputs"=w1206, "Write ERD List"=T52[] [{"ERD Number"=61462, "Data Type"=enum."string", "Data"="01"}], "Error In"=w1214, "Verify ERD Response?"=FALSE) -> ("GEA2 Reference Out"=w1231:refnum<k24>, "Error Out"=w1229:errorcluster)  [unwired: 8 in, 1 out]
            n204 = Not Equal?(x=w1223, y=path "") -> (x != y?=w1222:bool)
            n205 = call "Time Delay2"("error in (no error)"=w1229, "Delay Time (s)"=3.0) -> ("error out"=w1225:errorcluster)  [unwired: 9 in]
            n206 = case shown="True" w1222 {
              tunnel: w1225 -> [w1232 w1237]
              tunnel: [w1232 w1240] -> w1211
              tunnel: w1223 -> [_ w1249]
              tunnel: w1231 -> [_ w1243]
              frame False {
              }
              frame True {
                w1233 = T14 9 items=["ImageRejected", "BoardNotFound", "UnableToGetGeaConfiguration", "WriteToFlashNotAllowed", "ImageDownloadedSuccessfully", "ImagePresent", "WriteToFlashFailed", "EraseFailed", "CrcFailed", ""] ("Result")
                (unwired) 0 items=["ImageRejected", "BoardNotFound", "UnableToGetGeaConfiguration", "WriteToFlashNotAllowed", "ImageDownloadedSuccessfully", "ImagePresent", "WriteToFlashFailed", "EraseFailed", "CrcFailed"] ("Result")
                w1238 = FALSE ("Blinking")
                n207 = property on="Result" class="Ring (strict)"(error in=w1237, "Value"=w1233) -> (error out=w1242:errorcluster)  [unwired: 1 in, 1 out]
                n208 = property on="Board Index" class="DigNum (strict)"(error in=w1237, "DisabledEnum"=T53."Disabled and Grayed Out" ("Disabled")) -> ()  [unwired: 1 in, 2 out]
                n209 = call "GEA2 Flash APL.vi"("GEA2 Reference In"=w1243, "Force Update?"=TRUE, "Source Address"=u8 228, "Destination Address"="Programming Destination Address", "File Path"=w1249, "Error In"=w1242, "Broadcast"=TRUE, "Reset?"=FALSE ("Reset Board?")) -> ("Result"=w1241:i32, "Error Out"=w1234:errorcluster)  [unwired: 3 in, 3 out]
                n210 = property on="Result" class="Ring (strict)"(error in=w1234, "Value"=w1241) -> (error out=w1239:errorcluster)  [unwired: 1 in, 1 out]
                n211 = property on="Board Index" class="DigNum (strict)"(error in=w1234, "DisabledEnum"=T53."Enabled" ("Disabled")) -> ()  [unwired: 1 in, 2 out]
                n212 = property on="Program Ind" class="Bool (strict)"(error in=w1239, "Value"=w1238, "Blinking"=w1238) -> (error out=w1240:errorcluster)  [unwired: 1 in, 1 out]
              }
            }
            n213 = Enqueue Element(queue=w1210, element=T49 {"Data"=variant, "State"=enum."Init"} ("Data"), error in (no error)=w1211) -> (error out=w1209:errorcluster)  [unwired: 1 in, 2 out]
          }
          event Value Change {
            w1260 = T12 {"Source"=228, "Destination"=255, "Command"=221, "Message"="F401"} ("Input Data")
            n214 = event-data() -> ()  [unwired: 1 in, 6 out]
            n215 = call "GEA2 Send Message.vi"("GEA2 Reference In"=w1256, "Input Data"=w1260, "Error In"=w1257) -> ("Error Out"=w1262:errorcluster)  [unwired: 11 in, 1 out]
            n216 = call "GEA2MessageFormatter.vi"("Prefix(Send/Recv)"="SEND", "GEA2 Data In"=w1260, "Error In"=w1262) -> ("Output String"=w1259:string, "Error Out"=w1258:errorcluster)  [unwired: 11 in]
            n217 = call "GExplorer_Queue_GEA2.vi"("Output String"=w1259, "error in (no error)"=w1258) -> ("error out"=w1252:errorcluster)  [unwired: 13 in]
            n218 = call "Time Delay5"("error in (no error)"=w1252, "Delay Time (s)"=3.0) -> ("error out"=w1253:errorcluster)  [unwired: 9 in]
            n219 = Enqueue Element(queue=w1250, element=T49 {"Data"=variant, "State"=enum."Init"} ("Data"), error in (no error)=w1253) -> (error out=w1251:errorcluster)  [unwired: 1 in, 2 out]
          }
          event Value Change {
            w1269 = T12 {"Source"=228, "Destination"=35, "Command"=221, "Message"="07"} ("Input Data")
            n220 = event-data() -> ()  [unwired: 1 in, 6 out]
            n221 = call "GEA2 Send Message.vi"("GEA2 Reference In"=w1264, "Input Data"=w1269, "Error In"=w1266) -> ("GEA2 Reference Out"=w1263:refnum<k24>, "Error Out"=w1271:errorcluster)  [unwired: 11 in]
            n222 = call "GEA2MessageFormatter.vi"("Prefix(Send/Recv)"="SEND", "GEA2 Data In"=w1269, "Error In"=w1271) -> ("Output String"=w1268:string, "Error Out"=w1267:errorcluster)  [unwired: 11 in]
            n223 = call "GExplorer_Queue_GEA2.vi"("Output String"=w1268, "error in (no error)"=w1267) -> ("error out"=w1265:errorcluster)  [unwired: 13 in]
          }
          event "Reset": Value Change {
            w1278 = T52[] [{"ERD Number"=61462, "Data Type"=enum."string", "Data"="01"}] ("Write ERD List")
            n224 = event-data() -> ()  [unwired: 1 in, 6 out]
            n225 = call "GEA2 Write ERD.vi"("GEA2 Reference In"=w1287, "GEA Inputs"=w1277, "Write ERD List"=w1278, "Error In"=w1288, "Verify ERD Response?"=FALSE) -> ("GEA2 Reference Out"=w1275:refnum<k24>, "Error Out"=w1279:errorcluster)  [unwired: 8 in, 1 out]
            n226 = call "Convert Write ERD List to Message.vi"("GEA Inputs"=w1277, "Write ERD List"=w1278, "Error In"=w1279) -> ("GEA Message"=w1281:T12, "Error Out"=w1282:errorcluster)  [unwired: 11 in]
            n227 = call "GEA2MessageFormatter.vi"("Prefix(Send/Recv)"="SEND", "GEA2 Data In"=w1281, "Error In"=w1282) -> ("Output String"=w1283:string, "Error Out"=w1284:errorcluster)  [unwired: 11 in]
            n228 = call "GExplorer_Queue_GEA2.vi"("Output String"=w1283, "error in (no error)"=w1284) -> ("error out"=w1276:errorcluster)  [unwired: 13 in]
            n229 = Enqueue Element(queue=w1285, element=T49 {"Data"=variant, "State"=enum."Init"} ("Data"), error in (no error)=w1276) -> (error out=w1273:errorcluster)  [unwired: 1 in, 2 out]
            n230 = call "Time Delay9"("error in (no error)"=w1273, "Delay Time (s)"=3.0) -> ("error out"=w1272:errorcluster)  [unwired: 9 in]
          }
          event "Save Log": Value Change {
            n231 = event-data() -> ()  [unwired: 1 in, 6 out]
            n232 = property on="GEA2 Log" class="Str"(error in=w1295) -> (error out=w1297:errorcluster, "Value"=w1296:string)  [unwired: 1 in, 1 out]
            n233 = Write to Text File(prompt (Choose or enter file path)="Choose filename and path to save txt file to ", text=w1296, error in=w1297) -> (refnum out=w1294:refnum<file>, error out=w1293:errorcluster)  [unwired: 1 in, 1 out]
            n234 = Close File(refnum=w1294, error in=w1293) -> (error out=w1292:errorcluster)  [unwired: 1 out]
            n235 = call <vilib>:"Clear Errors.vi"("error in (no error)"=w1292, "specific error code to clear (0: all)"=43) -> ("error out"=w1291:errorcluster)  [unwired: 4 in, 1 out]
          }
          event "Lid Lock.Lock Lid", "Lid Lock.Unlock Lid", "Lid Lock.Reset Lock": Value Change {
            n236 = event-data() -> ("CtlRef"=w1303:refnum<vi>)  [unwired: 1 in, 5 out]
            n237 = property class="Bool"(reference=w1303, error in=w1304) -> (reference out=w1307:refnum<vi>, error out=w1308:errorcluster, "Label.Text"=w1309:string)
            n238 = Close Reference(reference=w1307, error in (no error)=w1308) -> (error out=w1306:errorcluster)
            n239 = case shown="\"Reset Lid\", Default" w1309 {
              tunnel: [w1316 w1333 w1351] -> w1305
              tunnel: w1301 -> [w1313 w1331 w1349]
              tunnel: w1306 -> [w1318 w1336 w1354]
              tunnel: w1302 -> [w1312 w1330 w1348]
              tunnel: [w1310 w1334 w1352] -> w1300
              tunnel: T52 {"ERD Number"=61554, "Data Type"=enum."string", "Data"=""} ("ERD Read Data In") -> [w1317 w1335 w1353]
              frame "Unlock Lid" {
                n240 = Concatenate Strings("01" ("string"), "00" ("string")) -> (w1326:string)
                n241 = Bundle By Name(cluster=w1317, "Data"=w1326) -> (w1325:T52)
                n242 = Build Array(w1325) -> (w1311:T52[])
                n243 = call "Convert Write ERD List to Message.vi"("GEA Inputs"=w1312, "Write ERD List"=w1311, "Error In"=w1318) -> ("GEA Message"=w1320:T12, "Error Out"=w1321:errorcluster)  [unwired: 11 in]
                n244 = call "GEA2MessageFormatter.vi"("Prefix(Send/Recv)"="SEND", "GEA2 Data In"=w1320, "Error In"=w1321) -> ("Output String"=w1322:string, "Error Out"=w1323:errorcluster)  [unwired: 11 in]
                n245 = call "GExplorer_Queue_GEA2.vi"("Output String"=w1322, "error in (no error)"=w1323) -> ("error out"=w1315:errorcluster)  [unwired: 13 in]
                n246 = call "GEA3 Write ERD (Rev 2 API) Multiple Messages.vi"("GEA2 Reference In"=w1313, "GEA Inputs"=w1312, "Write ERD List"=w1311, "Error In"=w1315, "Verify ERD Response?"=FALSE) -> ("GEA2 Reference Out"=w1310:refnum<k24>, "Error Out"=w1316:errorcluster)  [unwired: 8 in, 1 out]
              }
              frame "Reset Lid", Default {
                n247 = Concatenate Strings("00" ("string"), "00" ("string")) -> (w1344:string)
                n248 = Bundle By Name(cluster=w1335, "Data"=w1344) -> (w1343:T52)
                n249 = Build Array(w1343) -> (w1329:T52[])
                n250 = call "Convert Write ERD List to Message.vi"("GEA Inputs"=w1330, "Write ERD List"=w1329, "Error In"=w1336) -> ("GEA Message"=w1338:T12, "Error Out"=w1339:errorcluster)  [unwired: 11 in]
                n251 = call "GEA2MessageFormatter.vi"("Prefix(Send/Recv)"="SEND", "GEA2 Data In"=w1338, "Error In"=w1339) -> ("Output String"=w1340:string, "Error Out"=w1341:errorcluster)  [unwired: 11 in]
                n252 = call "GExplorer_Queue_GEA2.vi"("Output String"=w1340, "error in (no error)"=w1341) -> ("error out"=w1332:errorcluster)  [unwired: 13 in]
                n253 = call "GEA3 Write ERD (Rev 2 API) Multiple Messages.vi"("GEA2 Reference In"=w1331, "GEA Inputs"=w1330, "Write ERD List"=w1329, "Error In"=w1332, "Verify ERD Response?"=FALSE) -> ("GEA2 Reference Out"=w1334:refnum<k24>, "Error Out"=w1333:errorcluster)  [unwired: 8 in, 1 out]
              }
              frame "Lock Lid" {
                n254 = Concatenate Strings("01" ("string"), "01" ("string")) -> (w1362:string)
                n255 = Bundle By Name(cluster=w1353, "Data"=w1362) -> (w1361:T52)
                n256 = Build Array(w1361) -> (w1347:T52[])
                n257 = call "Convert Write ERD List to Message.vi"("GEA Inputs"=w1348, "Write ERD List"=w1347, "Error In"=w1354) -> ("GEA Message"=w1356:T12, "Error Out"=w1357:errorcluster)  [unwired: 11 in]
                n258 = call "GEA2MessageFormatter.vi"("Prefix(Send/Recv)"="SEND", "GEA2 Data In"=w1356, "Error In"=w1357) -> ("Output String"=w1358:string, "Error Out"=w1359:errorcluster)  [unwired: 11 in]
                n259 = call "GExplorer_Queue_GEA2.vi"("Output String"=w1358, "error in (no error)"=w1359) -> ("error out"=w1350:errorcluster)  [unwired: 13 in]
                n260 = call "GEA3 Write ERD (Rev 2 API) Multiple Messages.vi"("GEA2 Reference In"=w1349, "GEA Inputs"=w1348, "Write ERD List"=w1347, "Error In"=w1350, "Verify ERD Response?"=FALSE) -> ("GEA2 Reference Out"=w1352:refnum<k24>, "Error Out"=w1351:errorcluster)  [unwired: 8 in, 1 out]
              }
            }
          }
          event Value Change {
            n261 = event-data() -> ("CtlRef"=w1367:refnum<vi>)  [unwired: 1 in, 5 out]
            n262 = property class="Bool"(reference=w1367, error in=w1368) -> (reference out=w1371:refnum<vi>, error out=w1372:errorcluster, "Label.Text"=w1373:string)
            n263 = Close Reference(reference=w1371, error in (no error)=w1372) -> (error out=w1370:errorcluster)
            n264 = case shown="\"Redist Req\"" w1373 {
              tunnel: [w1387 w1403 w1419 w1435] -> w1369
              tunnel: w1365 -> [w1386 w1402 w1418 w1434]
              tunnel: w1370 -> [w1378 w1394 w1410 w1426]
              tunnel: w1366 -> [w1377 w1393 w1409 w1425]
              tunnel: [w1376 w1392 w1408 w1424] -> w1364
              frame "OOB in Accel", Default {
                n265 = Bundle By Name(cluster=T52 {"ERD Number"=61619, "Data Type"=enum."string", "Data"=""} ("ERD Read Data In"), "Data"="01") -> (w1388:T52)
                n266 = Build Array(w1388) -> (w1380:T52[])
                n267 = call "Convert Write ERD List to Message.vi"("GEA Inputs"=w1377, "Write ERD List"=w1380, "Error In"=w1378) -> ("GEA Message"=w1382:T12, "Error Out"=w1383:errorcluster)  [unwired: 11 in]
                n268 = call "GEA2MessageFormatter.vi"("Prefix(Send/Recv)"="SEND", "GEA2 Data In"=w1382, "Error In"=w1383) -> ("Output String"=w1384:string, "Error Out"=w1385:errorcluster)  [unwired: 11 in]
                n269 = call "GExplorer_Queue_GEA2.vi"("Output String"=w1384, "error in (no error)"=w1385) -> ("error out"=w1381:errorcluster)  [unwired: 13 in]
                n270 = call "GEA2 Write ERD.vi"("GEA2 Reference In"=w1386, "GEA Inputs"=w1377, "Write ERD List"=w1380, "Error In"=w1381, "Verify ERD Response?"=FALSE) -> ("GEA2 Reference Out"=w1376:refnum<k24>, "Error Out"=w1387:errorcluster)  [unwired: 8 in, 1 out]
              }
              frame "OOB in S-S" {
                n271 = Bundle By Name(cluster=T52 {"ERD Number"=61620, "Data Type"=enum."string", "Data"=""} ("ERD Read Data In"), "Data"="01") -> (w1404:T52)
                n272 = Build Array(w1404) -> (w1396:T52[])
                n273 = call "Convert Write ERD List to Message.vi"("GEA Inputs"=w1393, "Write ERD List"=w1396, "Error In"=w1394) -> ("GEA Message"=w1398:T12, "Error Out"=w1399:errorcluster)  [unwired: 11 in]
                n274 = call "GEA2MessageFormatter.vi"("Prefix(Send/Recv)"="SEND", "GEA2 Data In"=w1398, "Error In"=w1399) -> ("Output String"=w1400:string, "Error Out"=w1401:errorcluster)  [unwired: 11 in]
                n275 = call "GExplorer_Queue_GEA2.vi"("Output String"=w1400, "error in (no error)"=w1401) -> ("error out"=w1397:errorcluster)  [unwired: 13 in]
                n276 = call "GEA2 Write ERD.vi"("GEA2 Reference In"=w1402, "GEA Inputs"=w1393, "Write ERD List"=w1396, "Error In"=w1397, "Verify ERD Response?"=FALSE) -> ("GEA2 Reference Out"=w1392:refnum<k24>, "Error Out"=w1403:errorcluster)  [unwired: 8 in, 1 out]
              }
              frame "Redist Req" {
                n277 = Bundle By Name(cluster=T52 {"ERD Number"=61621, "Data Type"=enum."string", "Data"=""} ("ERD Read Data In"), "Data"="01") -> (w1420:T52)
                n278 = Build Array(w1420) -> (w1412:T52[])
                n279 = call "Convert Write ERD List to Message.vi"("GEA Inputs"=w1409, "Write ERD List"=w1412, "Error In"=w1410) -> ("GEA Message"=w1414:T12, "Error Out"=w1415:errorcluster)  [unwired: 11 in]
                n280 = call "GEA2MessageFormatter.vi"("Prefix(Send/Recv)"="SEND", "GEA2 Data In"=w1414, "Error In"=w1415) -> ("Output String"=w1416:string, "Error Out"=w1417:errorcluster)  [unwired: 11 in]
                n281 = call "GExplorer_Queue_GEA2.vi"("Output String"=w1416, "error in (no error)"=w1417) -> ("error out"=w1413:errorcluster)  [unwired: 13 in]
                n282 = call "GEA2 Write ERD.vi"("GEA2 Reference In"=w1418, "GEA Inputs"=w1409, "Write ERD List"=w1412, "Error In"=w1413, "Verify ERD Response?"=FALSE) -> ("GEA2 Reference Out"=w1408:refnum<k24>, "Error Out"=w1419:errorcluster)  [unwired: 8 in, 1 out]
              }
              frame "Suds Abtmt Req" {
                n283 = Bundle By Name(cluster=T52 {"ERD Number"=61641, "Data Type"=enum."string", "Data"=""} ("ERD Read Data In"), "Data"="01") -> (w1436:T52)
                n284 = Build Array(w1436) -> (w1428:T52[])
                n285 = call "Convert Write ERD List to Message.vi"("GEA Inputs"=w1425, "Write ERD List"=w1428, "Error In"=w1426) -> ("GEA Message"=w1430:T12, "Error Out"=w1431:errorcluster)  [unwired: 11 in]
                n286 = call "GEA2MessageFormatter.vi"("Prefix(Send/Recv)"="SEND", "GEA2 Data In"=w1430, "Error In"=w1431) -> ("Output String"=w1432:string, "Error Out"=w1433:errorcluster)  [unwired: 11 in]
                n287 = call "GExplorer_Queue_GEA2.vi"("Output String"=w1432, "error in (no error)"=w1433) -> ("error out"=w1429:errorcluster)  [unwired: 13 in]
                n288 = call "GEA2 Write ERD.vi"("GEA2 Reference In"=w1434, "GEA Inputs"=w1425, "Write ERD List"=w1428, "Error In"=w1429, "Verify ERD Response?"=FALSE) -> ("GEA2 Reference Out"=w1424:refnum<k24>, "Error Out"=w1435:errorcluster)  [unwired: 8 in, 1 out]
              }
            }
          }
          event "Run Script": Value Change {
            w1465 = T38 {"Overall Script File Progress"=0.0, "Current Script Progress"=0.0, "Script"="", "Test"="", "Elapsed time (s)"=0.0, "Done?"=FALSE}  # Script Info
            w1457 = T12 {"Source"=228, "Destination"=35, "Command"=1, "Message"=""}  # Version Query (for log header)
            n289 = event-data() -> ()  [unwired: 1 in, 6 out]
            n290 = Generate User Event(user event=w1438, event data cluster=TRUE ("event data"), error in=w1441) -> (error out=w1442:errorcluster)  [unwired: 1 in, 1 out]
            n291 = Enqueue Element(queue=w1439, element=T49 {"Data"=variant, "State"=enum."Pause"} ("Data"), error in (no error)=w1442) -> (error out=w1440:errorcluster)  [unwired: 1 in, 2 out]
            n292 = Obtain Queue(name (unnamed)="Script_Stop", element data type=FALSE, error in (no error)=w1440) -> (queue out=w1461:refnum<queue>, error out=w1464:errorcluster)  [unwired: 2 in, 1 out]
            n293 = Obtain Queue(name (unnamed)="Script_Info", element data type=w1465, error in (no error)=w1464) -> (queue out=w1467:refnum<queue>, error out=w1458:errorcluster)  [unwired: 2 in, 1 out]
            n294 = while {
              tunnel: w1467 -> [w1479]
              shift-right: [w1472] -> w1455
              shift-left: w1458 -> [w1475]
              tunnel: [w1478] -> w1466
              tunnel: w1461 -> [w1476]
              tunnel: [w1471] -> w1459
              stop <- w1477 stop-if-true
              n295 = Dequeue Element(queue=w1479, error in (no error)=w1475) -> (queue out=w1478:refnum<queue>, element=w1470:T38, error out=w1474:errorcluster)  [unwired: 1 in, 1 out]
              "Script Info" <- w1470
              n296 = Unbundle By Name(w1470) -> ("Done?"=w1477:bool)
              n297 = case shown="False" "stop script" {
                selector: "stop script" -> [_ w1482]
                tunnel: w1476 -> [w1481 w1486]
                tunnel: w1475 -> [w1480 w1485]
                tunnel: [w1480 w1484] -> w1473
                tunnel: [w1481 w1483] -> w1471
                frame False {
                }
                frame True {
                  n298 = Enqueue Element(queue=w1486, element=w1482, error in (no error)=w1485) -> (queue out=w1483:refnum<queue>, error out=w1484:errorcluster)  [unwired: 1 in, 1 out]
                }
              }
              n299 = Merge Errors(w1473, w1474) -> (w1472:errorcluster)
            }
            n300 = call "GEA2 Script Test SLB.vi"("GEA2 Reference In"=w1453, "Version Query (for log header)"=w1457, "Enqueue Sends?"=TRUE, "Standalone"=FALSE, "Script path"="Script Path", "Log File Path (empty for prompt)"="Script Log Path", "Error In"=w1458) -> ("Pass/Fail?"=→"Script Pass/Fail?":bool, "Report Text"=→"Script Report Text":string, "Error Out"=→"Script Error Out":errorcluster)  [unwired: 5 in, 1 out]
            n301 = Release Queue(queue=w1466, error in (no error)=w1455) -> (error out=w1460:errorcluster)  [unwired: 1 in, 2 out]
            n302 = Release Queue(queue=w1459, error in (no error)=w1460) -> (error out=w1445:errorcluster)  [unwired: 1 in, 2 out]
            n303 = Enqueue Element(queue=w1439, element=T49 {"Data"=variant, "State"=enum."Init"} ("Data"), error in (no error)=w1445) -> (error out=w1444:errorcluster)  [unwired: 1 in, 2 out]
          }
          event "Mode Shift.Shift to Spin", "Mode Shift.Disable", "Mode Shift.Shift to Agitate": Value Change {
            n304 = event-data() -> ("CtlRef"=w1497:refnum<vi>)  [unwired: 1 in, 5 out]
            n305 = property class="Bool"(reference=w1497, error in=w1496) -> (reference out=w1492:refnum<vi>, error out=w1494:errorcluster, "Label.Text"=w1495:string)
            n306 = Close Reference(reference=w1492, error in (no error)=w1494) -> (error out=w1493:errorcluster)
            n307 = case shown="\"Disable\", Default" w1495 {
              tunnel: w1493 -> [w1506 w1523 w1540]
              tunnel: w1491 -> [w1499 w1518 w1534]
              tunnel: w1490 -> [w1501 w1519 w1532]
              tunnel: [w1500 w1516 w1538] -> w1489
              tunnel: [w1504 w1521 w1537] -> w1488
              tunnel: T52 {"ERD Number"=61627, "Data Type"=enum."string", "Data"=""} ("ERD Read Data In") -> [w1505 w1522 w1539]
              frame "Shift to Spin" {
                n308 = Concatenate Strings("02" ("string")) -> (w1514:string)
                n309 = Bundle By Name(cluster=w1505, "Data"=w1514) -> (w1513:T52)
                n310 = Build Array(w1513) -> (w1498:T52[])
                n311 = call "Convert Write ERD List to Message.vi"("GEA Inputs"=w1499, "Write ERD List"=w1498, "Error In"=w1506) -> ("GEA Message"=w1508:T12, "Error Out"=w1509:errorcluster)  [unwired: 11 in]
                n312 = call "GEA2MessageFormatter.vi"("Prefix(Send/Recv)"="SEND", "GEA2 Data In"=w1508, "Error In"=w1509) -> ("Output String"=w1510:string, "Error Out"=w1511:errorcluster)  [unwired: 11 in]
                n313 = call "GExplorer_Queue_GEA2.vi"("Output String"=w1510, "error in (no error)"=w1511) -> ("error out"=w1503:errorcluster)  [unwired: 13 in]
                n314 = call "GEA3 Write ERD (Rev 2 API) Multiple Messages.vi"("GEA2 Reference In"=w1501, "GEA Inputs"=w1499, "Write ERD List"=w1498, "Error In"=w1503, "Verify ERD Response?"=FALSE) -> ("GEA2 Reference Out"=w1500:refnum<k24>, "Error Out"=w1504:errorcluster)  [unwired: 8 in, 1 out]
              }
              frame "Shift to Agitate" {
                n315 = Concatenate Strings("01" ("string")) -> (w1531:string)
                n316 = Bundle By Name(cluster=w1522, "Data"=w1531) -> (w1530:T52)
                n317 = Build Array(w1530) -> (w1517:T52[])
                n318 = call "Convert Write ERD List to Message.vi"("GEA Inputs"=w1518, "Write ERD List"=w1517, "Error In"=w1523) -> ("GEA Message"=w1525:T12, "Error Out"=w1526:errorcluster)  [unwired: 11 in]
                n319 = call "GEA2MessageFormatter.vi"("Prefix(Send/Recv)"="SEND", "GEA2 Data In"=w1525, "Error In"=w1526) -> ("Output String"=w1527:string, "Error Out"=w1528:errorcluster)  [unwired: 11 in]
                n320 = call "GExplorer_Queue_GEA2.vi"("Output String"=w1527, "error in (no error)"=w1528) -> ("error out"=w1520:errorcluster)  [unwired: 13 in]
                n321 = call "GEA3 Write ERD (Rev 2 API) Multiple Messages.vi"("GEA2 Reference In"=w1519, "GEA Inputs"=w1518, "Write ERD List"=w1517, "Error In"=w1520, "Verify ERD Response?"=FALSE) -> ("GEA2 Reference Out"=w1516:refnum<k24>, "Error Out"=w1521:errorcluster)  [unwired: 8 in, 1 out]
              }
              frame "Disable", Default {
                n322 = Concatenate Strings("00" ("string")) -> (w1548:string)
                n323 = Bundle By Name(cluster=w1539, "Data"=w1548) -> (w1547:T52)
                n324 = Build Array(w1547) -> (w1533:T52[])
                n325 = call "Convert Write ERD List to Message.vi"("GEA Inputs"=w1534, "Write ERD List"=w1533, "Error In"=w1540) -> ("GEA Message"=w1542:T12, "Error Out"=w1543:errorcluster)  [unwired: 11 in]
                n326 = call "GEA2MessageFormatter.vi"("Prefix(Send/Recv)"="SEND", "GEA2 Data In"=w1542, "Error In"=w1543) -> ("Output String"=w1544:string, "Error Out"=w1545:errorcluster)  [unwired: 11 in]
                n327 = call "GExplorer_Queue_GEA2.vi"("Output String"=w1544, "error in (no error)"=w1545) -> ("error out"=w1535:errorcluster)  [unwired: 13 in]
                n328 = call "GEA3 Write ERD (Rev 2 API) Multiple Messages.vi"("GEA2 Reference In"=w1532, "GEA Inputs"=w1534, "Write ERD List"=w1533, "Error In"=w1535, "Verify ERD Response?"=FALSE) -> ("GEA2 Reference Out"=w1538:refnum<k24>, "Error Out"=w1537:errorcluster)  [unwired: 8 in, 1 out]
              }
            }
          }
          event Value Change {
            n329 = event-data() -> ("CtlRef"=w1550:refnum<vi>)  [unwired: 1 in, 5 out]
            n330 = property class="Bool"(reference=w1550, error in=w1555) -> (reference out=w1556:refnum<vi>, error out=w1558:errorcluster, "Label.Text"=w1559:string)
            n331 = Close Reference(reference=w1556, error in (no error)=w1558) -> (error out=w1557:errorcluster)
            n332 = case shown="\"Select Profile\"" w1559 {
              tunnel: w1557 -> [w1568 w1590 w1611 w1633 w1655]
              tunnel: w1554 -> [w1560 w1583 w1604 w1626 w1649]
              tunnel: w1553 -> [w1562 w1585 w1606 w1625 w1650]
              tunnel: [w1563 w1588 w1609 w1631 w1651] -> w1552
              tunnel: [w1565 w1587 w1608 w1630 w1652] -> w1551
              tunnel: T52 {"ERD Number"=61624, "Data Type"=enum."string", "Data"=""} ("ERD Read Data In") -> [w1567 w1589 w1610 w1632 w1654]
              frame "Start Profile" {
                n333 = property on="Profile Selection" class="DigNum (strict)"(error in=w1568) -> (error out=w1570:errorcluster, "Value"=w1569:u8)  [unwired: 1 in, 1 out]
                n334 = Number To Hexadecimal String(1:i16 2 ("width (-)"), 2:w1569) -> (0:w1571:string)
                n335 = Concatenate Strings("01" ("string"), w1571, "01" ("string")) -> (w1573:string)
                n336 = Bundle By Name(cluster=w1567, "Data"=w1573) -> (w1574:T52)
                n337 = Build Array(w1574) -> (w1561:T52[])
                n338 = call "Convert Write ERD List to Message.vi"("GEA Inputs"=w1560, "Write ERD List"=w1561, "Error In"=w1570) -> ("GEA Message"=w1576:T12, "Error Out"=w1580:errorcluster)  [unwired: 11 in]
                n339 = call "GEA2MessageFormatter.vi"("Prefix(Send/Recv)"="SEND", "GEA2 Data In"=w1576, "Error In"=w1580) -> ("Output String"=w1578:string, "Error Out"=w1579:errorcluster)  [unwired: 11 in]
                n340 = call "GExplorer_Queue_GEA2.vi"("Output String"=w1578, "error in (no error)"=w1579) -> ("error out"=w1564:errorcluster)  [unwired: 13 in]
                n341 = call "GEA3 Write ERD (Rev 2 API) Multiple Messages.vi"("GEA2 Reference In"=w1562, "GEA Inputs"=w1560, "Write ERD List"=w1561, "Error In"=w1564, "Verify ERD Response?"=FALSE) -> ("GEA2 Reference Out"=w1563:refnum<k24>, "Error Out"=w1565:errorcluster)  [unwired: 8 in, 1 out]
              }
              frame "Stop Profile", Default {
                n342 = property on="Profile Selection" class="DigNum (strict)"(error in=w1590) -> (error out=w1592:errorcluster, "Value"=w1591:u8)  [unwired: 1 in, 1 out]
                n343 = Number To Hexadecimal String(1:i16 2 ("width (-)"), 2:w1591) -> (0:w1593:string)
                n344 = Concatenate Strings("01" ("string"), w1593, "02" ("string")) -> (w1595:string)
                n345 = Bundle By Name(cluster=w1589, "Data"=w1595) -> (w1596:T52)
                n346 = Build Array(w1596) -> (w1584:T52[])
                n347 = call "Convert Write ERD List to Message.vi"("GEA Inputs"=w1583, "Write ERD List"=w1584, "Error In"=w1592) -> ("GEA Message"=w1598:T12, "Error Out"=w1602:errorcluster)  [unwired: 11 in]
                n348 = call "GEA2MessageFormatter.vi"("Prefix(Send/Recv)"="SEND", "GEA2 Data In"=w1598, "Error In"=w1602) -> ("Output String"=w1600:string, "Error Out"=w1601:errorcluster)  [unwired: 11 in]
                n349 = call "GExplorer_Queue_GEA2.vi"("Output String"=w1600, "error in (no error)"=w1601) -> ("error out"=w1586:errorcluster)  [unwired: 13 in]
                n350 = call "GEA3 Write ERD (Rev 2 API) Multiple Messages.vi"("GEA2 Reference In"=w1585, "GEA Inputs"=w1583, "Write ERD List"=w1584, "Error In"=w1586, "Verify ERD Response?"=FALSE) -> ("GEA2 Reference Out"=w1588:refnum<k24>, "Error Out"=w1587:errorcluster)  [unwired: 8 in, 1 out]
              }
              frame "Pause Profile" {
                n351 = property on="Profile Selection" class="DigNum (strict)"(error in=w1611) -> (error out=w1613:errorcluster, "Value"=w1612:u8)  [unwired: 1 in, 1 out]
                n352 = Number To Hexadecimal String(1:i16 2 ("width (-)"), 2:w1612) -> (0:w1614:string)
                n353 = Concatenate Strings("01" ("string"), w1614, "03" ("string")) -> (w1616:string)
                n354 = Bundle By Name(cluster=w1610, "Data"=w1616) -> (w1617:T52)
                n355 = Build Array(w1617) -> (w1605:T52[])
                n356 = call "Convert Write ERD List to Message.vi"("GEA Inputs"=w1604, "Write ERD List"=w1605, "Error In"=w1613) -> ("GEA Message"=w1619:T12, "Error Out"=w1623:errorcluster)  [unwired: 11 in]
                n357 = call "GEA2MessageFormatter.vi"("Prefix(Send/Recv)"="SEND", "GEA2 Data In"=w1619, "Error In"=w1623) -> ("Output String"=w1621:string, "Error Out"=w1622:errorcluster)  [unwired: 11 in]
                n358 = call "GExplorer_Queue_GEA2.vi"("Output String"=w1621, "error in (no error)"=w1622) -> ()  [unwired: 13 in, 1 out]
                n359 = call "GEA3 Write ERD (Rev 2 API) Multiple Messages.vi"("GEA2 Reference In"=w1606, "GEA Inputs"=w1604, "Write ERD List"=w1605, "Verify ERD Response?"=FALSE) -> ("GEA2 Reference Out"=w1609:refnum<k24>, "Error Out"=w1608:errorcluster)  [unwired: 9 in, 1 out]
              }
              frame "Resume Profile" {
                n360 = property on="Profile Selection" class="DigNum (strict)"(error in=w1633) -> (error out=w1635:errorcluster, "Value"=w1634:u8)  [unwired: 1 in, 1 out]
                n361 = Number To Hexadecimal String(1:i16 2 ("width (-)"), 2:w1634) -> (0:w1636:string)
                n362 = Concatenate Strings("01" ("string"), w1636, "04" ("string")) -> (w1638:string)
                n363 = Bundle By Name(cluster=w1632, "Data"=w1638) -> (w1639:T52)
                n364 = Build Array(w1639) -> (w1627:T52[])
                n365 = call "Convert Write ERD List to Message.vi"("GEA Inputs"=w1626, "Write ERD List"=w1627, "Error In"=w1635) -> ("GEA Message"=w1641:T12, "Error Out"=w1645:errorcluster)  [unwired: 11 in]
                n366 = call "GEA2MessageFormatter.vi"("Prefix(Send/Recv)"="SEND", "GEA2 Data In"=w1641, "Error In"=w1645) -> ("Output String"=w1643:string, "Error Out"=w1644:errorcluster)  [unwired: 11 in]
                n367 = call "GExplorer_Queue_GEA2.vi"("Output String"=w1643, "error in (no error)"=w1644) -> ("error out"=w1628:errorcluster)  [unwired: 13 in]
                n368 = call "GEA3 Write ERD (Rev 2 API) Multiple Messages.vi"("GEA2 Reference In"=w1625, "GEA Inputs"=w1626, "Write ERD List"=w1627, "Error In"=w1628, "Verify ERD Response?"=FALSE) -> ("GEA2 Reference Out"=w1631:refnum<k24>, "Error Out"=w1630:errorcluster)  [unwired: 8 in, 1 out]
              }
              frame "Select Profile" {
                n369 = property on="Profile Selection" class="DigNum (strict)"(error in=w1655) -> (error out=w1657:errorcluster, "Value"=w1656:u8)  [unwired: 1 in, 1 out]
                n370 = Number To Hexadecimal String(1:i16 2 ("width (-)"), 2:w1656) -> (0:w1658:string)
                n371 = Concatenate Strings("01" ("string"), w1658, "05" ("string")) -> (w1660:string)
                n372 = Bundle By Name(cluster=w1654, "Data"=w1660) -> (w1661:T52)
                n373 = Build Array(w1661) -> (w1648:T52[])
                n374 = call "Convert Write ERD List to Message.vi"("GEA Inputs"=w1649, "Write ERD List"=w1648, "Error In"=w1657) -> ("GEA Message"=w1663:T12, "Error Out"=w1667:errorcluster)  [unwired: 11 in]
                n375 = call "GEA2MessageFormatter.vi"("Prefix(Send/Recv)"="SEND", "GEA2 Data In"=w1663, "Error In"=w1667) -> ("Output String"=w1665:string, "Error Out"=w1666:errorcluster)  [unwired: 11 in]
                n376 = call "GExplorer_Queue_GEA2.vi"("Output String"=w1665, "error in (no error)"=w1666) -> ("error out"=w1647:errorcluster)  [unwired: 13 in]
                n377 = call "GEA3 Write ERD (Rev 2 API) Multiple Messages.vi"("GEA2 Reference In"=w1650, "GEA Inputs"=w1649, "Write ERD List"=w1648, "Error In"=w1647, "Verify ERD Response?"=FALSE) -> ("GEA2 Reference Out"=w1651:refnum<k24>, "Error Out"=w1652:errorcluster)  [unwired: 8 in, 1 out]
              }
            }
          }
          event "Drain Pump.Drain Pump ON", "Drain Pump.Drain Pump OFF", "Drain Pump.Reset Drain Pump": Value Change {
            n378 = event-data() -> ("CtlRef"=w1674:refnum<vi>)  [unwired: 1 in, 5 out]
            n379 = property class="Bool"(reference=w1674, error in=w1673) -> (reference out=w1671:refnum<vi>, error out=w1672:errorcluster, "Label.Text"=w1670:string)
            n380 = Close Reference(reference=w1671, error in (no error)=w1672) -> (error out=w1679:errorcluster)
            n381 = case shown="\"Drain Pump ON\"" w1670 {
              tunnel: w1679 -> [w1697 w1715 w1733]
              tunnel: w1678 -> [w1682 w1700 w1717]
              tunnel: w1677 -> [w1683 w1703 w1718]
              tunnel: [w1686 w1704 w1722] -> w1676
              tunnel: [w1685 w1699 w1721] -> w1675
              tunnel: T52 {"ERD Number"=61560, "Data Type"=enum."string", "Data"=""} ("ERD Read Data In") -> [w1687 w1705 w1723]
              frame "Drain Pump ON" {
                n382 = Concatenate Strings("01" ("string"), "01" ("string")) -> (w1695:string)
                n383 = Bundle By Name(cluster=w1687, "Data"=w1695) -> (w1694:T52)
                n384 = Build Array(w1694) -> (w1681:T52[])
                n385 = call "Convert Write ERD List to Message.vi"("GEA Inputs"=w1682, "Write ERD List"=w1681, "Error In"=w1697) -> ("GEA Message"=w1689:T12, "Error Out"=w1690:errorcluster)  [unwired: 11 in]
                n386 = call "GEA2MessageFormatter.vi"("Prefix(Send/Recv)"="SEND", "GEA2 Data In"=w1689, "Error In"=w1690) -> ("Output String"=w1691:string, "Error Out"=w1692:errorcluster)  [unwired: 11 in]
                n387 = call "GExplorer_Queue_GEA2.vi"("Output String"=w1691, "error in (no error)"=w1692) -> ("error out"=w1684:errorcluster)  [unwired: 13 in]
                n388 = call "GEA3 Write ERD (Rev 2 API) Multiple Messages.vi"("GEA2 Reference In"=w1683, "GEA Inputs"=w1682, "Write ERD List"=w1681, "Error In"=w1684, "Verify ERD Response?"=FALSE) -> ("GEA2 Reference Out"=w1686:refnum<k24>, "Error Out"=w1685:errorcluster)  [unwired: 8 in, 1 out]
              }
              frame "Drain Pump OFF" {
                n389 = Concatenate Strings("01" ("string"), "00" ("string")) -> (w1713:string)
                n390 = Bundle By Name(cluster=w1705, "Data"=w1713) -> (w1712:T52)
                n391 = Build Array(w1712) -> (w1701:T52[])
                n392 = call "Convert Write ERD List to Message.vi"("GEA Inputs"=w1700, "Write ERD List"=w1701, "Error In"=w1715) -> ("GEA Message"=w1707:T12, "Error Out"=w1708:errorcluster)  [unwired: 11 in]
                n393 = call "GEA2MessageFormatter.vi"("Prefix(Send/Recv)"="SEND", "GEA2 Data In"=w1707, "Error In"=w1708) -> ("Output String"=w1709:string, "Error Out"=w1710:errorcluster)  [unwired: 11 in]
                n394 = call "GExplorer_Queue_GEA2.vi"("Output String"=w1709, "error in (no error)"=w1710) -> ("error out"=w1702:errorcluster)  [unwired: 13 in]
                n395 = call "GEA3 Write ERD (Rev 2 API) Multiple Messages.vi"("GEA2 Reference In"=w1703, "GEA Inputs"=w1700, "Write ERD List"=w1701, "Error In"=w1702, "Verify ERD Response?"=FALSE) -> ("GEA2 Reference Out"=w1704:refnum<k24>, "Error Out"=w1699:errorcluster)  [unwired: 8 in, 1 out]
              }
              frame "Reset Drain Pump", Default {
                n396 = Concatenate Strings("00" ("string"), "00" ("string")) -> (w1731:string)
                n397 = Bundle By Name(cluster=w1723, "Data"=w1731) -> (w1730:T52)
                n398 = Build Array(w1730) -> (w1719:T52[])
                n399 = call "Convert Write ERD List to Message.vi"("GEA Inputs"=w1717, "Write ERD List"=w1719, "Error In"=w1733) -> ("GEA Message"=w1725:T12, "Error Out"=w1726:errorcluster)  [unwired: 11 in]
                n400 = call "GEA2MessageFormatter.vi"("Prefix(Send/Recv)"="SEND", "GEA2 Data In"=w1725, "Error In"=w1726) -> ("Output String"=w1727:string, "Error Out"=w1728:errorcluster)  [unwired: 11 in]
                n401 = call "GExplorer_Queue_GEA2.vi"("Output String"=w1727, "error in (no error)"=w1728) -> ("error out"=w1720:errorcluster)  [unwired: 13 in]
                n402 = call "GEA3 Write ERD (Rev 2 API) Multiple Messages.vi"("GEA2 Reference In"=w1718, "GEA Inputs"=w1717, "Write ERD List"=w1719, "Error In"=w1720, "Verify ERD Response?"=FALSE) -> ("GEA2 Reference Out"=w1722:refnum<k24>, "Error Out"=w1721:errorcluster)  [unwired: 8 in, 1 out]
              }
            }
          }
          event "Recirculation Pump.Recirc Pump ON", "Recirculation Pump.Recirc Pump OFF", "Recirculation Pump.Reset Recirc Pump": Value Change {
            n403 = event-data() -> ("CtlRef"=w1739:refnum<vi>)  [unwired: 1 in, 5 out]
            n404 = property class="Bool"(reference=w1739, error in=w1738) -> (reference out=w1736:refnum<vi>, error out=w1737:errorcluster, "Label.Text"=w1735:string)
            n405 = Close Reference(reference=w1736, error in (no error)=w1737) -> (error out=w1744:errorcluster)
            n406 = case shown="\"Reset Recirc Pump\", Default" w1735 {
              tunnel: w1744 -> [w1762 w1780 w1798]
              tunnel: w1743 -> [w1745 w1763 w1782]
              tunnel: w1742 -> [w1747 w1765 w1783]
              tunnel: [w1748 w1769 w1787] -> w1741
              tunnel: [w1751 w1768 w1786] -> w1740
              tunnel: T52 {"ERD Number"=61561, "Data Type"=enum."string", "Data"=""} ("ERD Read Data In") -> [w1752 w1770 w1788]
              frame "Recirc Pump ON" {
                n407 = Concatenate Strings("01" ("string"), "01" ("string")) -> (w1760:string)
                n408 = Bundle By Name(cluster=w1752, "Data"=w1760) -> (w1759:T52)
                n409 = Build Array(w1759) -> (w1746:T52[])
                n410 = call "Convert Write ERD List to Message.vi"("GEA Inputs"=w1745, "Write ERD List"=w1746, "Error In"=w1762) -> ("GEA Message"=w1754:T12, "Error Out"=w1755:errorcluster)  [unwired: 11 in]
                n411 = call "GEA2MessageFormatter.vi"("Prefix(Send/Recv)"="SEND", "GEA2 Data In"=w1754, "Error In"=w1755) -> ("Output String"=w1756:string, "Error Out"=w1757:errorcluster)  [unwired: 11 in]
                n412 = call "GExplorer_Queue_GEA2.vi"("Output String"=w1756, "error in (no error)"=w1757) -> ("error out"=w1750:errorcluster)  [unwired: 13 in]
                n413 = call "GEA3 Write ERD (Rev 2 API) Multiple Messages.vi"("GEA2 Reference In"=w1747, "GEA Inputs"=w1745, "Write ERD List"=w1746, "Error In"=w1750, "Verify ERD Response?"=FALSE) -> ("GEA2 Reference Out"=w1748:refnum<k24>, "Error Out"=w1751:errorcluster)  [unwired: 8 in, 1 out]
              }
              frame "Recirc Pump OFF" {
                n414 = Concatenate Strings("01" ("string"), "00" ("string")) -> (w1778:string)
                n415 = Bundle By Name(cluster=w1770, "Data"=w1778) -> (w1777:T52)
                n416 = Build Array(w1777) -> (w1764:T52[])
                n417 = call "Convert Write ERD List to Message.vi"("GEA Inputs"=w1763, "Write ERD List"=w1764, "Error In"=w1780) -> ("GEA Message"=w1772:T12, "Error Out"=w1773:errorcluster)  [unwired: 11 in]
                n418 = call "GEA2MessageFormatter.vi"("Prefix(Send/Recv)"="SEND", "GEA2 Data In"=w1772, "Error In"=w1773) -> ("Output String"=w1774:string, "Error Out"=w1775:errorcluster)  [unwired: 11 in]
                n419 = call "GExplorer_Queue_GEA2.vi"("Output String"=w1774, "error in (no error)"=w1775) -> ("error out"=w1766:errorcluster)  [unwired: 13 in]
                n420 = call "GEA3 Write ERD (Rev 2 API) Multiple Messages.vi"("GEA2 Reference In"=w1765, "GEA Inputs"=w1763, "Write ERD List"=w1764, "Error In"=w1766, "Verify ERD Response?"=FALSE) -> ("GEA2 Reference Out"=w1769:refnum<k24>, "Error Out"=w1768:errorcluster)  [unwired: 8 in, 1 out]
              }
              frame "Reset Recirc Pump", Default {
                n421 = Concatenate Strings("00" ("string"), "00" ("string")) -> (w1796:string)
                n422 = Bundle By Name(cluster=w1788, "Data"=w1796) -> (w1795:T52)
                n423 = Build Array(w1795) -> (w1781:T52[])
                n424 = call "Convert Write ERD List to Message.vi"("GEA Inputs"=w1782, "Write ERD List"=w1781, "Error In"=w1798) -> ("GEA Message"=w1790:T12, "Error Out"=w1791:errorcluster)  [unwired: 11 in]
                n425 = call "GEA2MessageFormatter.vi"("Prefix(Send/Recv)"="SEND", "GEA2 Data In"=w1790, "Error In"=w1791) -> ("Output String"=w1792:string, "Error Out"=w1793:errorcluster)  [unwired: 11 in]
                n426 = call "GExplorer_Queue_GEA2.vi"("Output String"=w1792, "error in (no error)"=w1793) -> ("error out"=w1785:errorcluster)  [unwired: 13 in]
                n427 = call "GEA3 Write ERD (Rev 2 API) Multiple Messages.vi"("GEA2 Reference In"=w1783, "GEA Inputs"=w1782, "Write ERD List"=w1781, "Error In"=w1785, "Verify ERD Response?"=FALSE) -> ("GEA2 Reference Out"=w1787:refnum<k24>, "Error Out"=w1786:errorcluster)  [unwired: 8 in, 1 out]
              }
            }
          }
          event Value Change {
            n428 = event-data() -> ("CtlRef"=w1802:refnum<vi>)  [unwired: 1 in, 5 out]
            n429 = property class="Bool"(reference=w1802, error in=w1803) -> (reference out=w1807:refnum<vi>, error out=w1808:errorcluster, "Label.Text"=w1806:string)
            n430 = Close Reference(reference=w1807, error in (no error)=w1808) -> (error out=w1809:errorcluster)
            n431 = case shown="\"Select Cycle\"" w1806 {
              tunnel: w1809 -> [w1820 w1842 w1864 w1886 w1908]
              tunnel: w1805 -> [w1810 w1834 w1856 w1879 w1900]
              tunnel: w1804 -> [w1812 w1832 w1857 w1882 w1901]
              tunnel: [w1816 w1838 w1860 w1878 w1904] -> w1800
              tunnel: [w1815 w1837 w1859 w1877 w1903] -> w1801
              tunnel: T52 {"ERD Number"=61557, "Data Type"=enum."string", "Data"=""} ("ERD Read Data In") -> [w1817 w1839 w1861 w1883 w1905]
              frame "Start Cycle" {
                n432 = property on="Cycle Selection" class="DigNum (strict)"(error in=w1820) -> (error out=w1819:errorcluster, "Value"=w1818:u8)  [unwired: 1 in, 1 out]
                n433 = Number To Hexadecimal String(1:i16 2 ("width (-)"), 2:w1818) -> (0:w1831:string)
                n434 = Concatenate Strings("01" ("string"), w1831, "01" ("string")) -> (w1829:string)
                n435 = Bundle By Name(cluster=w1817, "Data"=w1829) -> (w1828:T52)
                n436 = Build Array(w1828) -> (w1811:T52[])
                n437 = call "Convert Write ERD List to Message.vi"("GEA Inputs"=w1810, "Write ERD List"=w1811, "Error In"=w1819) -> ("GEA Message"=w1826:T12, "Error Out"=w1822:errorcluster)  [unwired: 11 in]
                n438 = call "GEA2MessageFormatter.vi"("Prefix(Send/Recv)"="SEND", "GEA2 Data In"=w1826, "Error In"=w1822) -> ("Output String"=w1824:string, "Error Out"=w1823:errorcluster)  [unwired: 11 in]
                n439 = call "GExplorer_Queue_GEA2.vi"("Output String"=w1824, "error in (no error)"=w1823) -> ("error out"=w1813:errorcluster)  [unwired: 13 in]
                n440 = call "GEA3 Write ERD (Rev 2 API) Multiple Messages.vi"("GEA2 Reference In"=w1812, "GEA Inputs"=w1810, "Write ERD List"=w1811, "Error In"=w1813, "Verify ERD Response?"=FALSE) -> ("GEA2 Reference Out"=w1816:refnum<k24>, "Error Out"=w1815:errorcluster)  [unwired: 8 in, 1 out]
              }
              frame "Stop Cycle", Default {
                n441 = property on="Cycle Selection" class="DigNum (strict)"(error in=w1842) -> (error out=w1841:errorcluster, "Value"=w1840:u8)  [unwired: 1 in, 1 out]
                n442 = Number To Hexadecimal String(1:i16 2 ("width (-)"), 2:w1840) -> (0:w1853:string)
                n443 = Concatenate Strings("01" ("string"), w1853, "02" ("string")) -> (w1851:string)
                n444 = Bundle By Name(cluster=w1839, "Data"=w1851) -> (w1850:T52)
                n445 = Build Array(w1850) -> (w1833:T52[])
                n446 = call "Convert Write ERD List to Message.vi"("GEA Inputs"=w1834, "Write ERD List"=w1833, "Error In"=w1841) -> ("GEA Message"=w1848:T12, "Error Out"=w1844:errorcluster)  [unwired: 11 in]
                n447 = call "GEA2MessageFormatter.vi"("Prefix(Send/Recv)"="SEND", "GEA2 Data In"=w1848, "Error In"=w1844) -> ("Output String"=w1846:string, "Error Out"=w1845:errorcluster)  [unwired: 11 in]
                n448 = call "GExplorer_Queue_GEA2.vi"("Output String"=w1846, "error in (no error)"=w1845) -> ("error out"=w1835:errorcluster)  [unwired: 13 in]
                n449 = call "GEA3 Write ERD (Rev 2 API) Multiple Messages.vi"("GEA2 Reference In"=w1832, "GEA Inputs"=w1834, "Write ERD List"=w1833, "Error In"=w1835, "Verify ERD Response?"=FALSE) -> ("GEA2 Reference Out"=w1838:refnum<k24>, "Error Out"=w1837:errorcluster)  [unwired: 8 in, 1 out]
              }
              frame "Pause Cycle" {
                n450 = property on="Cycle Selection" class="DigNum (strict)"(error in=w1864) -> (error out=w1863:errorcluster, "Value"=w1862:u8)  [unwired: 1 in, 1 out]
                n451 = Number To Hexadecimal String(1:i16 2 ("width (-)"), 2:w1862) -> (0:w1875:string)
                n452 = Concatenate Strings("01" ("string"), w1875, "03" ("string")) -> (w1873:string)
                n453 = Bundle By Name(cluster=w1861, "Data"=w1873) -> (w1872:T52)
                n454 = Build Array(w1872) -> (w1855:T52[])
                n455 = call "Convert Write ERD List to Message.vi"("GEA Inputs"=w1856, "Write ERD List"=w1855, "Error In"=w1863) -> ("GEA Message"=w1870:T12, "Error Out"=w1866:errorcluster)  [unwired: 11 in]
                n456 = call "GEA2MessageFormatter.vi"("Prefix(Send/Recv)"="SEND", "GEA2 Data In"=w1870, "Error In"=w1866) -> ("Output String"=w1868:string, "Error Out"=w1867:errorcluster)  [unwired: 11 in]
                n457 = call "GExplorer_Queue_GEA2.vi"("Output String"=w1868, "error in (no error)"=w1867) -> ("error out"=w1858:errorcluster)  [unwired: 13 in]
                n458 = call "GEA3 Write ERD (Rev 2 API) Multiple Messages.vi"("GEA2 Reference In"=w1857, "GEA Inputs"=w1856, "Write ERD List"=w1855, "Error In"=w1858, "Verify ERD Response?"=FALSE) -> ("GEA2 Reference Out"=w1860:refnum<k24>, "Error Out"=w1859:errorcluster)  [unwired: 8 in, 1 out]
              }
              frame "Resume Cycle" {
                n459 = property on="Cycle Selection" class="DigNum (strict)"(error in=w1886) -> (error out=w1885:errorcluster, "Value"=w1884:u8)  [unwired: 1 in, 1 out]
                n460 = Number To Hexadecimal String(1:i16 2 ("width (-)"), 2:w1884) -> (0:w1897:string)
                n461 = Concatenate Strings("01" ("string"), w1897, "04" ("string")) -> (w1895:string)
                n462 = Bundle By Name(cluster=w1883, "Data"=w1895) -> (w1894:T52)
                n463 = Build Array(w1894) -> (w1880:T52[])
                n464 = call "Convert Write ERD List to Message.vi"("GEA Inputs"=w1879, "Write ERD List"=w1880, "Error In"=w1885) -> ("GEA Message"=w1892:T12, "Error Out"=w1888:errorcluster)  [unwired: 11 in]
                n465 = call "GEA2MessageFormatter.vi"("Prefix(Send/Recv)"="SEND", "GEA2 Data In"=w1892, "Error In"=w1888) -> ("Output String"=w1890:string, "Error Out"=w1889:errorcluster)  [unwired: 11 in]
                n466 = call "GExplorer_Queue_GEA2.vi"("Output String"=w1890, "error in (no error)"=w1889) -> ("error out"=w1881:errorcluster)  [unwired: 13 in]
                n467 = call "GEA3 Write ERD (Rev 2 API) Multiple Messages.vi"("GEA2 Reference In"=w1882, "GEA Inputs"=w1879, "Write ERD List"=w1880, "Error In"=w1881, "Verify ERD Response?"=FALSE) -> ("GEA2 Reference Out"=w1878:refnum<k24>, "Error Out"=w1877:errorcluster)  [unwired: 8 in, 1 out]
              }
              frame "Select Cycle" {
                n468 = property on="Cycle Selection" class="DigNum (strict)"(error in=w1908) -> (error out=w1907:errorcluster, "Value"=w1906:u8)  [unwired: 1 in, 1 out]
                n469 = Number To Hexadecimal String(1:i16 2 ("width (-)"), 2:w1906) -> (0:w1919:string)
                n470 = Concatenate Strings("01" ("string"), w1919, "05" ("string")) -> (w1917:string)
                n471 = Bundle By Name(cluster=w1905, "Data"=w1917) -> (w1916:T52)
                n472 = Build Array(w1916) -> (w1899:T52[])
                n473 = call "Convert Write ERD List to Message.vi"("GEA Inputs"=w1900, "Write ERD List"=w1899, "Error In"=w1907) -> ("GEA Message"=w1914:T12, "Error Out"=w1910:errorcluster)  [unwired: 11 in]
                n474 = call "GEA2MessageFormatter.vi"("Prefix(Send/Recv)"="SEND", "GEA2 Data In"=w1914, "Error In"=w1910) -> ("Output String"=w1912:string, "Error Out"=w1911:errorcluster)  [unwired: 11 in]
                n475 = call "GExplorer_Queue_GEA2.vi"("Output String"=w1912, "error in (no error)"=w1911) -> ("error out"=w1902:errorcluster)  [unwired: 13 in]
                n476 = call "GEA3 Write ERD (Rev 2 API) Multiple Messages.vi"("GEA2 Reference In"=w1901, "GEA Inputs"=w1900, "Write ERD List"=w1899, "Error In"=w1902, "Verify ERD Response?"=FALSE) -> ("GEA2 Reference Out"=w1904:refnum<k24>, "Error Out"=w1903:errorcluster)  [unwired: 8 in, 1 out]
              }
            }
          }
          event "LED Control.ALL LEDs ON", "LED Control.ALL LEDs OFF", "LED Control.Reset LEDs": Value Change {
            n477 = event-data() -> ("CtlRef"=w1923:refnum<vi>)  [unwired: 1 in, 5 out]
            n478 = property class="Bool"(reference=w1923, error in=w1924) -> (reference out=w1928:refnum<vi>, error out=w1929:errorcluster, "Label.Text"=w1927:string)
            n479 = Close Reference(reference=w1928, error in (no error)=w1929) -> (error out=w1930:errorcluster)
            n480 = case shown="\"ALL LEDs ON\"" w1927 {
              tunnel: w1930 -> [w1939 w1956 w1974]
              tunnel: w1926 -> [w1933 w1950 w1965]
              tunnel: w1925 -> [w1934 w1949 w1969]
              tunnel: [w1937 w1954 w1972] -> w1921
              tunnel: [w1936 w1953 w1971] -> w1922
              tunnel: T52 {"ERD Number"=61513, "Data Type"=enum."string", "Data"=""} ("ERD Read Data In") -> [w1938 w1955 w1973]
              frame "ALL LEDs ON" {
                n481 = Concatenate Strings("0101FFFFFFFFFFFFFFFFFFFF" ("string")) -> (w1947:string)
                n482 = Bundle By Name(cluster=w1938, "Data"=w1947) -> (w1946:T52)
                n483 = Build Array(w1946) -> (w1932:T52[])
                n484 = call "Convert Write ERD List to Message.vi"("GEA Inputs"=w1933, "Write ERD List"=w1932, "Error In"=w1939) -> ("GEA Message"=w1941:T12, "Error Out"=w1942:errorcluster)  [unwired: 11 in]
                n485 = call "GEA2MessageFormatter.vi"("Prefix(Send/Recv)"="SEND", "GEA2 Data In"=w1941, "Error In"=w1942) -> ("Output String"=w1943:string, "Error Out"=w1944:errorcluster)  [unwired: 11 in]
                n486 = call "GExplorer_Queue_GEA2.vi"("Output String"=w1943, "error in (no error)"=w1944) -> ("error out"=w1935:errorcluster)  [unwired: 13 in]
                n487 = call "GEA3 Write ERD (Rev 2 API) Multiple Messages.vi"("GEA2 Reference In"=w1934, "GEA Inputs"=w1933, "Write ERD List"=w1932, "Error In"=w1935, "Verify ERD Response?"=FALSE) -> ("GEA2 Reference Out"=w1937:refnum<k24>, "Error Out"=w1936:errorcluster)  [unwired: 8 in, 1 out]
              }
              frame "ALL LEDs OFF" {
                n488 = Concatenate Strings("010100000000000000000000" ("string")) -> (w1964:string)
                n489 = Bundle By Name(cluster=w1955, "Data"=w1964) -> (w1963:T52)
                n490 = Build Array(w1963) -> (w1948:T52[])
                n491 = call "Convert Write ERD List to Message.vi"("GEA Inputs"=w1950, "Write ERD List"=w1948, "Error In"=w1956) -> ("GEA Message"=w1958:T12, "Error Out"=w1959:errorcluster)  [unwired: 11 in]
                n492 = call "GEA2MessageFormatter.vi"("Prefix(Send/Recv)"="SEND", "GEA2 Data In"=w1958, "Error In"=w1959) -> ("Output String"=w1960:string, "Error Out"=w1961:errorcluster)  [unwired: 11 in]
                n493 = call "GExplorer_Queue_GEA2.vi"("Output String"=w1960, "error in (no error)"=w1961) -> ("error out"=w1951:errorcluster)  [unwired: 13 in]
                n494 = call "GEA3 Write ERD (Rev 2 API) Multiple Messages.vi"("GEA2 Reference In"=w1949, "GEA Inputs"=w1950, "Write ERD List"=w1948, "Error In"=w1951, "Verify ERD Response?"=FALSE) -> ("GEA2 Reference Out"=w1954:refnum<k24>, "Error Out"=w1953:errorcluster)  [unwired: 8 in, 1 out]
              }
              frame "Reset LEDS", Default {
                (unwired) FALSE ("Verify ERD Response?")
                (unwired) FALSE ("Verify ERD Response?")
                n495 = Concatenate Strings("010100000000000000000000" ("string")) -> (w1982:string)
                n496 = Bundle By Name(cluster=w1973, "Data"=w1982) -> (w1981:T52)
                n497 = Build Array(w1981) -> (w1968:T52[])
                n498 = call "Convert Write ERD List to Message.vi"("GEA Inputs"=w1965, "Write ERD List"=w1968, "Error In"=w1974) -> ("GEA Message"=w1976:T12, "Error Out"=w1977:errorcluster)  [unwired: 11 in]
                n499 = call "GEA2MessageFormatter.vi"("Prefix(Send/Recv)"="SEND", "GEA2 Data In"=w1976, "Error In"=w1977) -> ("Output String"=w1978:string, "Error Out"=w1979:errorcluster)  [unwired: 11 in]
                n500 = call "GExplorer_Queue_GEA2.vi"("Output String"=w1978, "error in (no error)"=w1979) -> ()  [unwired: 13 in, 1 out]
                n501 = call "GEA3 Write ERD (Rev 2 API) Multiple Messages.vi"("GEA2 Reference In"=w1969, "GEA Inputs"=w1965, "Write ERD List"=w1968) -> ("GEA2 Reference Out"=w1970:refnum<k24>, "Error Out"=w1967:errorcluster)  [unwired: 10 in, 1 out]
                n502 = Concatenate Strings("000000000000000000000000" ("string")) -> (w1990:string)
                n503 = Bundle By Name(cluster=w1973, "Data"=w1990) -> (w1989:T52)
                n504 = Build Array(w1989) -> (w1966:T52[])
                n505 = call "Convert Write ERD List to Message.vi"("GEA Inputs"=w1965, "Write ERD List"=w1966, "Error In"=w1967) -> ("GEA Message"=w1984:T12, "Error Out"=w1985:errorcluster)  [unwired: 11 in]
                n506 = call "GEA2MessageFormatter.vi"("Prefix(Send/Recv)"="SEND", "GEA2 Data In"=w1984, "Error In"=w1985) -> ("Output String"=w1986:string, "Error Out"=w1987:errorcluster)  [unwired: 11 in]
                n507 = call "GExplorer_Queue_GEA2.vi"("Output String"=w1986, "error in (no error)"=w1987) -> ()  [unwired: 13 in, 1 out]
                n508 = call "GEA3 Write ERD (Rev 2 API) Multiple Messages.vi"("GEA2 Reference In"=w1970, "GEA Inputs"=w1965, "Write ERD List"=w1966) -> ("GEA2 Reference Out"=w1972:refnum<k24>, "Error Out"=w1971:errorcluster)  [unwired: 10 in, 1 out]
              }
            }
          }
          event Value Change {
            n509 = event-data() -> ("CtlRef"=w1995:refnum<vi>)  [unwired: 1 in, 5 out]
            n510 = property class="Bool"(reference=w1995, error in=w1996) -> (reference out=w2000:refnum<vi>, error out=w2001:errorcluster, "Label.Text"=w1999:string)
            n511 = Close Reference(reference=w2000, error in (no error)=w2001) -> (error out=w2002:errorcluster)
            n512 = case shown="\"Valves ON\"" w1999 {
              tunnel: w2002 -> [w2012 w2041]
              tunnel: w1998 -> [w2005 w2029]
              tunnel: w1997 -> [w2006 w2032]
              tunnel: "Valve Control" -> [w2013 _]
              tunnel: [w2007 w2033] -> w1993
              tunnel: [w2009 w2035] -> w1992
              tunnel: T52 {"ERD Number"=61553, "Data Type"=enum."string", "Data"=""} ("ERD Read Data In") -> [w2011 w2037]
              frame "Valves ON" {
                n513 = Unbundle By Name(w2013) -> ("Hot Valve"=w2026:bool, "Cold Valve"=w2025:bool, "SprayRinse Valve"=w2024:bool, "FabricSoftener Valve"=w2023:bool, "Bulk Dispense Valve"=w2010:bool)
                n514 = Build Array(w2026, w2025, w2024, w2023, w2010) -> (w2022:bool[])
                n515 = Boolean Array To Number(Boolean array=w2022) -> (number=w2020:u32)
                n516 = Number To Hexadecimal String(1:i16 2 ("width (-)"), 2:w2020) -> (0:w2019:string)
                n517 = Bundle By Name(cluster=w2011, "Data"=w2019) -> (w2027:T52)
                n518 = Build Array(w2027) -> (w2004:T52[])
                n519 = call "Convert Write ERD List to Message.vi"("GEA Inputs"=w2005, "Write ERD List"=w2004, "Error In"=w2012) -> ("GEA Message"=w2015:T12, "Error Out"=w2016:errorcluster)  [unwired: 11 in]
                n520 = call "GEA2MessageFormatter.vi"("Prefix(Send/Recv)"="SEND", "GEA2 Data In"=w2015, "Error In"=w2016) -> ("Output String"=w2017:string, "Error Out"=w2018:errorcluster)  [unwired: 11 in]
                n521 = call "GExplorer_Queue_GEA2.vi"("Output String"=w2017, "error in (no error)"=w2018) -> ("error out"=w2008:errorcluster)  [unwired: 13 in]
                n522 = call "GEA3 Write ERD (Rev 2 API) Multiple Messages.vi"("GEA2 Reference In"=w2006, "GEA Inputs"=w2005, "Write ERD List"=w2004, "Error In"=w2008, "Verify ERD Response?"=FALSE) -> ("GEA2 Reference Out"=w2007:refnum<k24>, "Error Out"=w2009:errorcluster)  [unwired: 8 in, 1 out]
              }
              frame "Valves OFF", Default {
                (unwired) FALSE ("Verify ERD Response?")
                w2034 = FALSE ("Value")
                n523 = Bundle By Name(cluster=w2037, "Data"="00" ("string")) -> (w2048:T52)
                n524 = Build Array(w2048) -> (w2030:T52[])
                n525 = call "Convert Write ERD List to Message.vi"("GEA Inputs"=w2029, "Write ERD List"=w2030, "Error In"=w2041) -> ("GEA Message"=w2043:T12, "Error Out"=w2044:errorcluster)  [unwired: 11 in]
                n526 = call "GEA2MessageFormatter.vi"("Prefix(Send/Recv)"="SEND", "GEA2 Data In"=w2043, "Error In"=w2044) -> ("Output String"=w2045:string, "Error Out"=w2046:errorcluster)  [unwired: 11 in]
                n527 = call "GExplorer_Queue_GEA2.vi"("Output String"=w2045, "error in (no error)"=w2046) -> ("error out"=w2031:errorcluster)  [unwired: 13 in]
                n528 = call "GEA3 Write ERD (Rev 2 API) Multiple Messages.vi"("GEA2 Reference In"=w2032, "GEA Inputs"=w2029, "Write ERD List"=w2030, "Error In"=w2031) -> ("GEA2 Reference Out"=w2033:refnum<k24>, "Error Out"=w2028:errorcluster)  [unwired: 9 in, 1 out]
                n529 = property on="Cold" class="Bool (strict)"(error in=w2028, "Value"=w2034) -> (error out=w2040:errorcluster)  [unwired: 1 in, 1 out]
                n530 = property on="Hot" class="Bool (strict)"(error in=w2040, "Value"=w2034) -> (error out=w2039:errorcluster)  [unwired: 1 in, 1 out]
                n531 = property on="Spray" class="Bool (strict)"(error in=w2039, "Value"=w2034) -> (error out=w2038:errorcluster)  [unwired: 1 in, 1 out]
                n532 = property on="FS" class="Bool (strict)"(error in=w2038, "Value"=w2034) -> (error out=w2036:errorcluster)  [unwired: 1 in, 1 out]
                n533 = property on="Bulk" class="Bool (strict)"(error in=w2036, "Value"=w2034) -> (error out=w2035:errorcluster)  [unwired: 1 in, 1 out]
              }
            }
          }
          event Value Change {
            n534 = event-data() -> ("CtlRef"=w2051:refnum<vi>)  [unwired: 1 in, 5 out]
            n535 = property class="Bool"(reference=w2051, error in=w2052) -> (reference out=w2056:refnum<vi>, error out=w2057:errorcluster, "Label.Text"=w2055:string)
            n536 = Close Reference(reference=w2056, error in (no error)=w2057) -> (error out=w2058:errorcluster)
            n537 = case shown="\"Relays OFF\", Default" w2055 {
              tunnel: w2058 -> [w2065 w2077]
              tunnel: w2054 -> [w2060 w2072]
              tunnel: w2053 -> [w2061 w2073]
              tunnel: [w2064 w2076] -> w2050
              tunnel: [w2063 w2075] -> w2049
              frame "Relays ON" {
                w2059 = T52[] [{"ERD Number"=61633, "Data Type"=enum."string", "Data"="00 01"}, {"ERD Number"=61567, "Data Type"=enum."string", "Data"="00 01"}, {"ERD Number"=61891, "Data Type"=enum."string", "Data"="02"}] ("Write ERD List")
                (unwired) FALSE ("Verify ERD Response?")
                n538 = call "Convert Write ERD List to Message.vi"("GEA Inputs"=w2060, "Write ERD List"=w2059, "Error In"=w2065) -> ("GEA Message"=w2067:T12, "Error Out"=w2068:errorcluster)  [unwired: 11 in]
                n539 = call "GEA2MessageFormatter.vi"("Prefix(Send/Recv)"="SEND", "GEA2 Data In"=w2067, "Error In"=w2068) -> ("Output String"=w2069:string, "Error Out"=w2070:errorcluster)  [unwired: 11 in]
                n540 = call "GExplorer_Queue_GEA2.vi"("Output String"=w2069, "error in (no error)"=w2070) -> ("error out"=w2062:errorcluster)  [unwired: 13 in]
                n541 = call "GEA3 Write ERD (Rev 2 API) Multiple Messages.vi"("GEA2 Reference In"=w2061, "GEA Inputs"=w2060, "Write ERD List"=w2059, "Error In"=w2062) -> ("GEA2 Reference Out"=w2064:refnum<k24>, "Error Out"=w2063:errorcluster)  [unwired: 9 in, 1 out]
              }
              frame "Relays OFF", Default {
                w2071 = T52[] [{"ERD Number"=61633, "Data Type"=enum."string", "Data"="00 00"}, {"ERD Number"=61567, "Data Type"=enum."string", "Data"="00 00"}, {"ERD Number"=61891, "Data Type"=enum."string", "Data"="00"}] ("Write ERD List")
                (unwired) FALSE ("Verify ERD Response?")
                n542 = call "Convert Write ERD List to Message.vi"("GEA Inputs"=w2072, "Write ERD List"=w2071, "Error In"=w2077) -> ("GEA Message"=w2079:T12, "Error Out"=w2080:errorcluster)  [unwired: 11 in]
                n543 = call "GEA2MessageFormatter.vi"("Prefix(Send/Recv)"="SEND", "GEA2 Data In"=w2079, "Error In"=w2080) -> ("Output String"=w2081:string, "Error Out"=w2082:errorcluster)  [unwired: 11 in]
                n544 = call "GExplorer_Queue_GEA2.vi"("Output String"=w2081, "error in (no error)"=w2082) -> ("error out"=w2074:errorcluster)  [unwired: 13 in]
                n545 = call "GEA3 Write ERD (Rev 2 API) Multiple Messages.vi"("GEA2 Reference In"=w2073, "GEA Inputs"=w2072, "Write ERD List"=w2071, "Error In"=w2074) -> ("GEA2 Reference Out"=w2076:refnum<k24>, "Error Out"=w2075:errorcluster)  [unwired: 9 in, 1 out]
              }
            }
          }
          event Value Change {
            n546 = event-data() -> ("CtlRef"=w2087:refnum<vi>)  [unwired: 1 in, 5 out]
            n547 = property class="Ctl"(reference=w2087, error in=w2088) -> (reference out=w2092:refnum<vi>, error out=w2093:errorcluster, "Label.Text"=w2091:string)
            n548 = Close Reference(reference=w2092, error in (no error)=w2093) -> (error out=w2094:errorcluster)
            n549 = case shown="\"Start Motor\"" w2091 {
              tunnel: w2094 -> [w2097 w2150 w2175]
              tunnel: w2090 -> [_ w2148 w2165]
              tunnel: w2089 -> [_ w2149 w2172]
              tunnel: [_ w2151 w2173] -> w2086
              tunnel: [w2095 w2152 w2174] -> w2085
              tunnel: "Motor Control" -> [w2096 _ w2171]
              tunnel: T52 {"ERD Number"=61622, "Data Type"=enum."string", "Data"=""} ("ERD Read Data In") -> [_ w2146 w2163]
              frame "Motor Profile Mode", Default {
                n550 = Unbundle By Name(w2096) -> ("Motor Profile Mode"=w2098:u16)
                n551 = case shown="0, Default" w2098 {
                  tunnel: w2097 -> [w2105 w2111 w2117 w2124 w2131 w2138 w2145]
                  tunnel: [w2100 w2107 w2113 w2120 w2126 w2134 w2141] -> w2095
                  frame 0, Default {
                    w2099 = T53."Disabled and Grayed Out" ("Disabled")
                    w2103 = T53."Enabled" ("Disabled")
                    n552 = property on="Speed (RPM)" class="DigNum (strict)"(error in=w2105, "DisabledEnum"=w2103) -> (error out=w2104:errorcluster)  [unwired: 1 in, 1 out]
                    n553 = property on="Acceleration" class="DigNum (strict)"(error in=w2104, "DisabledEnum"=w2103) -> (error out=w2102:errorcluster)  [unwired: 1 in, 1 out]
                    n554 = property on="Angle (Degrees)" class="DigNum (strict)"(error in=w2102, "DisabledEnum"=w2099) -> (error out=w2101:errorcluster)  [unwired: 1 in, 1 out]
                    n555 = property on="Amplitude (%)\n-CCW +CW" class="DigNum (strict)"(error in=w2101, "DisabledEnum"=w2099) -> (error out=w2100:errorcluster)  [unwired: 1 in, 1 out]
                  }
                  frame 1 {
                    w2106 = T53."Disabled and Grayed Out" ("Disabled")
                    n556 = property on="Speed (RPM)" class="DigNum (strict)"(error in=w2111, "DisabledEnum"=w2106) -> (error out=w2110:errorcluster)  [unwired: 1 in, 1 out]
                    n557 = property on="Acceleration" class="DigNum (strict)"(error in=w2110, "DisabledEnum"=w2106) -> (error out=w2109:errorcluster)  [unwired: 1 in, 1 out]
                    n558 = property on="Angle (Degrees)" class="DigNum (strict)"(error in=w2109, "DisabledEnum"=w2106) -> (error out=w2108:errorcluster)  [unwired: 1 in, 1 out]
                    n559 = property on="Amplitude (%)\n-CCW +CW" class="DigNum (strict)"(error in=w2108, "DisabledEnum"=w2106) -> (error out=w2107:errorcluster)  [unwired: 1 in, 1 out]
                  }
                  frame 6 {
                    w2112 = T53."Disabled and Grayed Out" ("Disabled")
                    n560 = property on="Speed (RPM)" class="DigNum (strict)"(error in=w2117, "DisabledEnum"=w2112) -> (error out=w2116:errorcluster)  [unwired: 1 in, 1 out]
                    n561 = property on="Acceleration" class="DigNum (strict)"(error in=w2116, "DisabledEnum"=w2112) -> (error out=w2115:errorcluster)  [unwired: 1 in, 1 out]
                    n562 = property on="Angle (Degrees)" class="DigNum (strict)"(error in=w2115, "DisabledEnum"=w2112) -> (error out=w2114:errorcluster)  [unwired: 1 in, 1 out]
                    n563 = property on="Amplitude (%)\n-CCW +CW" class="DigNum (strict)"(error in=w2114, "DisabledEnum"=w2112) -> (error out=w2113:errorcluster)  [unwired: 1 in, 1 out]
                  }
                  frame 2 {
                    w2119 = T53."Disabled and Grayed Out" ("Disabled")
                    n564 = property on="Speed (RPM)" class="DigNum (strict)"(error in=w2124, "DisabledEnum"=w2119) -> (error out=w2123:errorcluster)  [unwired: 1 in, 1 out]
                    n565 = property on="Acceleration" class="DigNum (strict)"(error in=w2123, "DisabledEnum"=w2119) -> (error out=w2122:errorcluster)  [unwired: 1 in, 1 out]
                    n566 = property on="Angle (Degrees)" class="DigNum (strict)"(error in=w2122, "DisabledEnum"=w2119) -> (error out=w2121:errorcluster)  [unwired: 1 in, 1 out]
                    n567 = property on="Amplitude (%)\n-CCW +CW" class="DigNum (strict)"(error in=w2121, "DisabledEnum"=T53."Enabled" ("Disabled")) -> (error out=w2120:errorcluster)  [unwired: 1 in, 1 out]
                  }
                  frame 3 {
                    w2125 = T53."Enabled" ("Disabled")
                    w2129 = T53."Disabled and Grayed Out" ("Disabled")
                    n568 = property on="Speed (RPM)" class="DigNum (strict)"(error in=w2131, "DisabledEnum"=w2129) -> (error out=w2130:errorcluster)  [unwired: 1 in, 1 out]
                    n569 = property on="Acceleration" class="DigNum (strict)"(error in=w2130, "DisabledEnum"=w2129) -> (error out=w2128:errorcluster)  [unwired: 1 in, 1 out]
                    n570 = property on="Angle (Degrees)" class="DigNum (strict)"(error in=w2128, "DisabledEnum"=w2125) -> (error out=w2127:errorcluster)  [unwired: 1 in, 1 out]
                    n571 = property on="Amplitude (%)\n-CCW +CW" class="DigNum (strict)"(error in=w2127, "DisabledEnum"=w2125) -> (error out=w2126:errorcluster)  [unwired: 1 in, 1 out]
                  }
                  frame 4 {
                    w2132 = T53."Disabled and Grayed Out" ("Disabled")
                    n572 = property on="Speed (RPM)" class="DigNum (strict)"(error in=w2138, "DisabledEnum"=T53."Enabled" ("Disabled")) -> (error out=w2137:errorcluster)  [unwired: 1 in, 1 out]
                    n573 = property on="Acceleration" class="DigNum (strict)"(error in=w2137, "DisabledEnum"=w2132) -> (error out=w2136:errorcluster)  [unwired: 1 in, 1 out]
                    n574 = property on="Angle (Degrees)" class="DigNum (strict)"(error in=w2136, "DisabledEnum"=w2132) -> (error out=w2135:errorcluster)  [unwired: 1 in, 1 out]
                    n575 = property on="Amplitude (%)\n-CCW +CW" class="DigNum (strict)"(error in=w2135, "DisabledEnum"=w2132) -> (error out=w2134:errorcluster)  [unwired: 1 in, 1 out]
                  }
                  frame 5 {
                    w2139 = T53."Disabled and Grayed Out" ("Disabled")
                    n576 = property on="Speed (RPM)" class="DigNum (strict)"(error in=w2145, "DisabledEnum"=T53."Enabled" ("Disabled")) -> (error out=w2144:errorcluster)  [unwired: 1 in, 1 out]
                    n577 = property on="Acceleration" class="DigNum (strict)"(error in=w2144, "DisabledEnum"=w2139) -> (error out=w2143:errorcluster)  [unwired: 1 in, 1 out]
                    n578 = property on="Angle (Degrees)" class="DigNum (strict)"(error in=w2143, "DisabledEnum"=w2139) -> (error out=w2142:errorcluster)  [unwired: 1 in, 1 out]
                    n579 = property on="Amplitude (%)\n-CCW +CW" class="DigNum (strict)"(error in=w2142, "DisabledEnum"=w2139) -> (error out=w2141:errorcluster)  [unwired: 1 in, 1 out]
                  }
                }
              }
              frame "Stop Motor" {
                n580 = Concatenate Strings("06 00 00 00 00 00 00 00 00 00 00 00" ("string")) -> (w2162:string)
                n581 = Bundle By Name(cluster=w2146, "Data"=w2162) -> (w2161:T52)
                n582 = Build Array(w2161) -> (w2155:T52[])
                n583 = call "Convert Write ERD List to Message.vi"("GEA Inputs"=w2148, "Write ERD List"=w2155, "Error In"=w2150) -> ("GEA Message"=w2157:T12, "Error Out"=w2158:errorcluster)  [unwired: 11 in]
                n584 = call "GEA2MessageFormatter.vi"("Prefix(Send/Recv)"="SEND", "GEA2 Data In"=w2157, "Error In"=w2158) -> ("Output String"=w2159:string, "Error Out"=w2160:errorcluster)  [unwired: 11 in]
                n585 = call "GExplorer_Queue_GEA2.vi"("Output String"=w2159, "error in (no error)"=w2160) -> ("error out"=w2156:errorcluster)  [unwired: 13 in]
                n586 = call "GEA2 Write ERD.vi"("GEA2 Reference In"=w2149, "GEA Inputs"=w2148, "Write ERD List"=w2155, "Error In"=w2156, "Verify ERD Response?"=FALSE) -> ("GEA2 Reference Out"=w2151:refnum<k24>, "Error Out"=w2152:errorcluster)  [unwired: 8 in, 1 out]
              }
              frame "Start Motor" {
                n587 = Unbundle By Name(w2171) -> ("Motor Profile Mode"=w2170:u16, "Speed (RPM)"=w2169:i16, "Acceleration"=w2168:i16, "Angle (Degrees)"=w2167:i16, "Amplitude (%)\n-CCW +CW"=w2166:i16)
                n588 = Number To Hexadecimal String(1:i16 2 ("width (-)"), 2:w2170) -> (0:w2186:string)
                n589 = Number To Hexadecimal String(1:i16 4 ("width (-)"), 2:w2169) -> (0:w2185:string)
                n590 = Number To Hexadecimal String(1:i16 4 ("width (-)"), 2:w2168) -> (0:w2180:string)
                n591 = Number To Hexadecimal String(1:i16 4 ("width (-)"), 2:w2167) -> (0:w2179:string)
                n592 = Number To Hexadecimal String(1:i16 4 ("width (-)"), 2:w2166) -> (0:w2178:string)
                n593 = Concatenate Strings(w2186, "00" ("string"), w2185, w2180, w2179, "0000" ("string"), w2178) -> (w2196:string)
                n594 = Bundle By Name(cluster=w2163, "Data"=w2196) -> (w2195:T52)
                n595 = Build Array(w2195) -> (w2189:T52[])
                n596 = call "Convert Write ERD List to Message.vi"("Write ERD List"=w2189, "Error In"=w2175) -> ("GEA Message"=w2191:T12, "Error Out"=w2192:errorcluster)  [unwired: 12 in]
                n597 = call "GEA2MessageFormatter.vi"("Prefix(Send/Recv)"="SEND", "GEA2 Data In"=w2191, "Error In"=w2192) -> ("Output String"=w2193:string, "Error Out"=w2194:errorcluster)  [unwired: 11 in]
                n598 = call "GExplorer_Queue_GEA2.vi"("Output String"=w2193, "error in (no error)"=w2194) -> ("error out"=w2190:errorcluster)  [unwired: 13 in]
                n599 = call "GEA2 Write ERD.vi"("GEA2 Reference In"=w2172, "GEA Inputs"=w2165, "Write ERD List"=w2189, "Error In"=w2190, "Verify ERD Response?"=FALSE) -> ("GEA2 Reference Out"=w2173:refnum<k24>, "Error Out"=w2174:errorcluster)  [unwired: 8 in, 1 out]
              }
            }
          }
          event "Test Mode.Exit Test Mode": Value Change {
            (unwired) FALSE ("Verify ERD Response?")
            n600 = event-data() -> ()  [unwired: 1 in, 6 out]
            n601 = Concatenate Strings("00" ("string")) -> (w2211:string)
            n602 = Bundle By Name(cluster=T52 {"ERD Number"=61461, "Data Type"=enum."string", "Data"=""} ("ERD Read Data In"), "Data"=w2211) -> (w2204:T52)
            n603 = Build Array(w2204) -> (w2197:T52[])
            n604 = call "Convert Write ERD List to Message.vi"("GEA Inputs"=w2199, "Write ERD List"=w2197, "Error In"=w2203) -> ("GEA Message"=w2206:T12, "Error Out"=w2207:errorcluster)  [unwired: 11 in]
            n605 = call "GEA2MessageFormatter.vi"("Prefix(Send/Recv)"="SEND", "GEA2 Data In"=w2206, "Error In"=w2207) -> ("Output String"=w2208:string, "Error Out"=w2209:errorcluster)  [unwired: 11 in]
            n606 = call "GExplorer_Queue_GEA2.vi"("Output String"=w2208, "error in (no error)"=w2209) -> ()  [unwired: 13 in, 1 out]
            n607 = call "GEA3 Write ERD (Rev 2 API) Multiple Messages.vi"("GEA2 Reference In"=w2200, "GEA Inputs"=w2199, "Write ERD List"=w2197) -> ("GEA2 Reference Out"=w2202:refnum<k24>, "Error Out"=w2201:errorcluster)  [unwired: 10 in, 1 out]
          }
          event "Fault ON", "ERD Graphing ON": Value Change {
            n608 = event-data() -> ()  [unwired: 1 in, 6 out]
            n609 = Enqueue Element(queue=w2213, element=T49 {"Data"=variant, "State"=enum."Build ERD Read List"}, error in (no error)=w2215) -> (error out=w2214:errorcluster)  [unwired: 1 in, 2 out]
            n610 = call "Write_Header_FGV.vi"("Write Header ? In"=FALSE, "Action"=enum16{"Get", "Set"}."Set", "Error In"=w2214) -> ("Error Out"=w2217:errorcluster)  [unwired: 11 in, 1 out]
          }
          event "Save Fault Log": Value Change {
            (unwired) FALSE ("Verify ERD Response?")
            # "0-9 Sequence\n10-21 Table"
            n611 = event-data() -> ()  [unwired: 1 in, 6 out]
            n612 = call "GEA3 Read ERD (Rev 2 API) Multiple Messages.vi"("GEA2 Reference In"=w2224, "Read Timeout (ms)"=u32 250, "GEA Inputs"=w2220, "Read ERD List"=T9[] [{"ERD Number"=57615, "Data Type"=enum."string"}, {"ERD Number"=141, "Data Type"=enum."uint32_t"}, {"ERD Number"=57617, "Data Type"=enum."string"}, {"ERD Number"=57618, "Data Type"=enum."string"}, {"ERD Number"=57619, "Data Type"=enum."string"}, {"ERD Number"=57620, "Data Type"=enum."string"}, {"ERD Number"=57621, "Data Type"=enum."string"}, {"ERD Number"=57622, "Data Type"=enum."string"}, {"ERD Number"=57623, "Data Type"=enum."string"}, {"ERD Number"=57624, "Data Type"=enum."string"}, {"ERD Number"=57603, "Data Type"=enum."string"}, {"ERD Number"=57605, "Data Type"=enum."string"}, {"ERD Number"=57606, "Data Type"=enum."string"}, {"ERD Number"=57607, "Data Type"=enum."string"}, {"ERD Number"=57608, "Data Type"=enum."string"}, {"ERD Number"=57609, "Data Type"=enum."string"}, {"ERD Number"=57610, "Data Type"=enum."string"}, {"ERD Number"=57611, "Data Type"=enum."string"}, {"ERD Number"=57612, "Data Type"=enum."string"}, {"ERD Number"=57613, "Data Type"=enum."string"}, {"ERD Number"=57614, "Data Type"=enum."string"}], "Error In"=w2225) -> ("ERD Data Out"=w2223:cluster{"ERD Number":u16, "Data":string}[], "Error Out"=w2226:errorcluster)  [unwired: 7 in, 2 out]
            n613 = Array Subset(array=w2223, index=10, length=11) -> (w2232:cluster{"ERD Number":u16, "Data":string}[])
            n614 = Array Subset(array=w2223, index=0, length=9) -> (w2231:cluster{"ERD Number":u16, "Data":string}[])
            n615 = call "Fault_Seq_Read.vi"("Seq ERD In"=w2231) -> ("String"=w2230:string)  [unwired: 13 in, 1 out]
            n616 = call "Fault_Table_Read.vi"("ERD Data Out"=w2232) -> ("Fault Table String Out"=w2229:string[][])  [unwired: 11 in, 3 out]
            n617 = call "Fault_Logging.vi"("String"=w2230, "Fault Table String Out"=w2229, "Path"=w2219, "error in (no error)"=w2226) -> ("error out"=w2228:errorcluster)  [unwired: 11 in]
          }
          event "Clear Fault Seq Buffer": Value Change {
            w2240 = T52[] [{"ERD Number"=57626, "Data Type"=enum."string", "Data"="01"}] ("Write ERD List")
            n618 = event-data() -> ()  [unwired: 1 in, 6 out]
            n619 = call "Convert Write ERD List to Message.vi"("GEA Inputs"=w2239, "Write ERD List"=w2240, "Error In"=w2243) -> ("GEA Message"=w2245:T12, "Error Out"=w2246:errorcluster)  [unwired: 11 in]
            n620 = call "GEA2MessageFormatter.vi"("Prefix(Send/Recv)"="SEND", "GEA2 Data In"=w2245, "Error In"=w2246) -> ("Output String"=w2247:string, "Error Out"=w2248:errorcluster)  [unwired: 11 in]
            n621 = call "GExplorer_Queue_GEA2.vi"("Output String"=w2247, "error in (no error)"=w2248) -> ("error out"=w2241:errorcluster)  [unwired: 13 in]
            n622 = call "GEA3 Write ERD (Rev 2 API) Multiple Messages.vi"("GEA2 Reference In"=w2238, "GEA Inputs"=w2239, "Write ERD List"=w2240, "Error In"=w2241, "Verify ERD Response?"=FALSE) -> ("GEA2 Reference Out"=w2237:refnum<k24>, "Error Out"=w2242:errorcluster)  [unwired: 8 in, 1 out]
          }
          event "Clear Fault Table Buffer": Value Change {
            (unwired) FALSE ("Verify ERD Response?")
            w2251 = T52[] [{"ERD Number"=57604, "Data Type"=enum."string", "Data"="01"}] ("Write ERD List")
            n623 = event-data() -> ()  [unwired: 1 in, 6 out]
            n624 = call "Convert Write ERD List to Message.vi"("GEA Inputs"=w2250, "Write ERD List"=w2251, "Error In"=w2255) -> ("GEA Message"=w2257:T12, "Error Out"=w2258:errorcluster)  [unwired: 11 in]
            n625 = call "GEA2MessageFormatter.vi"("Prefix(Send/Recv)"="SEND", "GEA2 Data In"=w2257, "Error In"=w2258) -> ("Output String"=w2259:string, "Error Out"=w2260:errorcluster)  [unwired: 11 in]
            n626 = call "GExplorer_Queue_GEA2.vi"("Output String"=w2259, "error in (no error)"=w2260) -> ("error out"=w2252:errorcluster)  [unwired: 13 in]
            n627 = call "GEA3 Write ERD (Rev 2 API) Multiple Messages.vi"("GEA2 Reference In"=w2249, "GEA Inputs"=w2250, "Write ERD List"=w2251, "Error In"=w2252) -> ("GEA2 Reference Out"=w2254:refnum<k24>, "Error Out"=w2253:errorcluster)  [unwired: 9 in, 1 out]
          }
          event "ADC Info Button": Value Change {
            w2287 = T12 {"Source"=228, "Destination"=35, "Command"=240, "Message"="03F0A7F06CF06B"}  # ADC ERDs
            w2267 = u16 0 ("Motor Current ADC")
            w2272 = 2 ("length (rest)")
            # "Ex. 03 50 09 02 DD 0F 40 04 02 E3 0F 40 03 02 E3 0F"
            n628 = event-data() -> ()  [unwired: 1 in, 6 out]
            n629 = call "GEA2MessageFormatter.vi"("Prefix(Send/Recv)"="SEND", "GEA2 Data In"=w2287, "Error In"=w2266) -> ("Output String"=w2286:string, "Error Out"=w2289:errorcluster)  [unwired: 11 in]
            n630 = call "GExplorer_Queue_GEA2.vi"("Output String"=w2286, "error in (no error)"=w2289) -> ("error out"=w2288:errorcluster)  [unwired: 13 in]
            n631 = call "GEA2 Send and Receive Message.vi"("GEA2 Reference In"=w2264, "Input Data"=w2287, "Error In"=w2288) -> ("Converted Data Out"=w2285:T57, "Error Out"=w2265:errorcluster)  [unwired: 9 in, 2 out]
            n632 = Unbundle By Name(w2285) -> ("Message"=w2271:string)
            n633 = String Subset(string=w2271, offset (0)=12, length (rest)=w2272) -> (substring=w2280:string)
            n634 = String Subset(string=w2271, offset (0)=15, length (rest)=w2272) -> (substring=w2279:string)
            n635 = String Subset(string=w2271, offset (0)=27, length (rest)=w2272) -> (substring=w2277:string)
            n636 = String Subset(string=w2271, offset (0)=30, length (rest)=w2272) -> (substring=w2275:string)
            n637 = String Subset(string=w2271, offset (0)=42, length (rest)=w2272) -> (substring=w2269:string)
            n638 = String Subset(string=w2271, offset (0)=45, length (rest)=w2272) -> (substring=w2270:string)
            n639 = Concatenate Strings(w2280, w2279) -> (w2282:string)
            n640 = Concatenate Strings(w2277, w2275) -> (w2278:string)
            n641 = Concatenate Strings(w2269, w2270) -> (w2268:string)
            n642 = Hexadecimal String To Number(string=w2282, default (0uL)=w2267) -> (number=→"Motor Current ADC":u16)  [unwired: 1 in, 1 out]
            n643 = Hexadecimal String To Number(string=w2278, default (0uL)=w2267) -> (number=→"Temp ADC":u16)  [unwired: 1 in, 1 out]
            n644 = Hexadecimal String To Number(string=w2268, default (0uL)=w2267) -> (number=→"Pressure ADC":u16)  [unwired: 1 in, 1 out]
          }
          event "Clear Cycle Buffer": Value Change {
            n645 = event-data() -> ()  [unwired: 1 in, 6 out]
            n646 = Build Array(T52 {"ERD Number"=57634, "Data Type"=enum."string", "Data"="01"} ("ERD Read Data In")) -> (w2306:T52[])
            n647 = call "Convert Write ERD List to Message.vi"("GEA Inputs"=w2301, "Write ERD List"=w2306, "Error In"=w2304) -> ("GEA Message"=w2308:T12, "Error Out"=w2309:errorcluster)  [unwired: 11 in]
            n648 = call "GEA2MessageFormatter.vi"("Prefix(Send/Recv)"="SEND", "GEA2 Data In"=w2308, "Error In"=w2309) -> ("Output String"=w2310:string, "Error Out"=w2311:errorcluster)  [unwired: 11 in]
            n649 = call "GExplorer_Queue_GEA2.vi"("Output String"=w2310, "error in (no error)"=w2311) -> ("error out"=w2307:errorcluster)  [unwired: 13 in]
            n650 = call "GEA2 Write ERD.vi"("GEA2 Reference In"=w2303, "GEA Inputs"=w2301, "Write ERD List"=w2306, "Error In"=w2307, "Verify ERD Response?"=FALSE) -> ("Error Out"=w2300:errorcluster)  [unwired: 8 in, 2 out]
            n651 = call "Time Delay6"("error in (no error)"=w2300, "Delay Time (s)"=1.0) -> ("error out"=w2295:errorcluster)  [unwired: 9 in]
            n652 = property on="Get Cycle History" class="Bool"(error in=w2295, "Val(Sgnl)"=TRUE ("Get Cycle History")) -> (error out=w2299:errorcluster)  [unwired: 1 in, 1 out]
            n653 = call "Time Delay7"("error in (no error)"=w2299, "Delay Time (s)"=1.0) -> ("error out"=w2294:errorcluster)  [unwired: 9 in]
            n654 = property on="Get Cycle History" class="Bool"(error in=w2294, "Val(Sgnl)"=FALSE ("Get Cycle History")) -> (error out=w2298:errorcluster)  [unwired: 1 in, 1 out]
          }
          event "Get Cycle History": Value Change {
            w2313 = T9[] [{"ERD Number"=57637, "Data Type"=enum."string"}, {"ERD Number"=57638, "Data Type"=enum."string"}, {"ERD Number"=57639, "Data Type"=enum."string"}, {"ERD Number"=57640, "Data Type"=enum."string"}, {"ERD Number"=57641, "Data Type"=enum."string"}, {"ERD Number"=57642, "Data Type"=enum."string"}, {"ERD Number"=57643, "Data Type"=enum."string"}, {"ERD Number"=57644, "Data Type"=enum."string"}, {"ERD Number"=57645, "Data Type"=enum."string"}, {"ERD Number"=57646, "Data Type"=enum."string"}] ("Read ERD List")
            n655 = event-data() -> ()  [unwired: 1 in, 6 out]
            n656 = call "Convert Read ERD List to Message.vi"("GEA Inputs"=w2312, "Read ERD List"=w2313, "Error In"=w2324) -> ("GEA Message"=w2328:T12, "Error Out"=w2329:errorcluster)  [unwired: 11 in]
            n657 = call "GEA2MessageFormatter.vi"("Prefix(Send/Recv)"="SEND", "GEA2 Data In"=w2328, "Error In"=w2329) -> ("Output String"=w2327:string, "Error Out"=w2326:errorcluster)  [unwired: 11 in]
            n658 = call "GExplorer_Queue_GEA2.vi"("Output String"=w2327, "error in (no error)"=w2326) -> ("error out"=w2318:errorcluster)  [unwired: 13 in]
            n659 = call "GEA3 Read ERD (Rev 2 API) Multiple Messages.vi"("GEA2 Reference In"=w2317, "Retry Count"=2 ("#ERDs per message"), "Read Timeout (ms)"=u32 500, "GEA Inputs"=w2312, "Read ERD List"=w2313, "Error In"=w2318, "Verify ERD Response?"=TRUE) -> ("ERD Data Out"=w2319:cluster{"ERD Number":u16, "Data":string}[], "Error Out"=w2320:errorcluster)  [unwired: 5 in, 2 out]
            n660 = call "Cycle_Diag_Table_Read_Mio.vi"("ERD Data In"=w2319, "error in (no error)"=w2320) -> ("Cycle Buffer Status"=→"Cycle Buffer Status":T33, "Diag Cycle String Out"=→"Diagnostics Table":string[][], "error out (no error)"=w2321:errorcluster)  [unwired: 11 in]
          }
          event "Save Cycle History Log": Value Change {
            w2330 = T9[] [{"ERD Number"=57633, "Data Type"=enum."string"}, {"ERD Number"=57635, "Data Type"=enum."string"}, {"ERD Number"=57636, "Data Type"=enum."string"}, {"ERD Number"=57637, "Data Type"=enum."string"}, {"ERD Number"=57638, "Data Type"=enum."string"}, {"ERD Number"=57639, "Data Type"=enum."string"}, {"ERD Number"=57640, "Data Type"=enum."string"}, {"ERD Number"=57641, "Data Type"=enum."string"}, {"ERD Number"=57642, "Data Type"=enum."string"}, {"ERD Number"=57643, "Data Type"=enum."string"}, {"ERD Number"=57644, "Data Type"=enum."string"}] ("Read ERD List")
            n661 = event-data() -> ()  [unwired: 1 in, 6 out]
            n662 = call "Convert Read ERD List to Message.vi"("GEA Inputs"=w2337, "Read ERD List"=w2330, "Error In"=w2336) -> ("GEA Message"=w2343:T12, "Error Out"=w2344:errorcluster)  [unwired: 11 in]
            n663 = call "GEA2MessageFormatter.vi"("Prefix(Send/Recv)"="SEND", "GEA2 Data In"=w2343, "Error In"=w2344) -> ("Output String"=w2342:string, "Error Out"=w2341:errorcluster)  [unwired: 11 in]
            n664 = call "GExplorer_Queue_GEA2.vi"("Output String"=w2342, "error in (no error)"=w2341) -> ("error out"=w2339:errorcluster)  [unwired: 13 in]
            n665 = call "GEA2 Read ERD Multiple Messages.vi"("GEA2 Reference In"=w2335, "Read Timeout (ms)"=u32 500, "GEA Inputs"=w2337, "Read ERD List"=w2330, "Error In"=w2339, "#ERDs per message"=2, "Verify ERD Response?"=TRUE) -> ("ERD Data Out"=w2334:cluster{"ERD Number":u16, "Data":string}[], "Error Out"=w2338:errorcluster)  [unwired: 5 in, 2 out]
            n666 = call "Cycle_Diag_Table_Read.vi"("ERD Data In"=w2334, "error in (no error)"=w2338) -> ("Diag Cycle String Out"=w2333:string[][], "error out"=w2332:errorcluster)  [unwired: 10 in, 2 out]
            n667 = call "Cycle_History_Logging.vi"("error in (no error)"=w2332, "Diag Cycle String Out"=w2333) -> ("error out"=w2331:errorcluster)  [unwired: 9 in]
          }
          event "Set Accel Reg": Value Change {
            n668 = event-data() -> ()  [unwired: 1 in, 6 out]
            n669 = Concatenate Strings("Register", "Value") -> (w2356:string)
            n670 = Bundle By Name(cluster=T52 {"ERD Number"=61645, "Data Type"=enum."string", "Data"=""} ("ERD Read Data In"), "Data"=w2356) -> (w2357:T52)
            n671 = Build Array(w2357) -> (w2351:T52[])
            n672 = call "Convert Write ERD List to Message.vi"("GEA Inputs"=w2350, "Write ERD List"=w2351, "Error In"=w2359) -> ("GEA Message"=w2361:T12, "Error Out"=w2362:errorcluster)  [unwired: 11 in]
            n673 = call "GEA2MessageFormatter.vi"("Prefix(Send/Recv)"="SEND", "GEA2 Data In"=w2361, "Error In"=w2362) -> ("Output String"=w2363:string, "Error Out"=w2364:errorcluster)  [unwired: 11 in]
            n674 = call "GExplorer_Queue_GEA2.vi"("Output String"=w2363, "error in (no error)"=w2364) -> ("error out"=w2352:errorcluster)  [unwired: 13 in]
            n675 = call "GEA3 Write ERD (Rev 2 API) Multiple Messages.vi"("GEA2 Reference In"=w2349, "GEA Inputs"=w2350, "Write ERD List"=w2351, "Error In"=w2352, "Verify ERD Response?"=FALSE) -> ("Error Out"=w2353:errorcluster)  [unwired: 8 in, 2 out]
          }
          event "Get Accel Reg": Value Change {
            w2372 = T9[] [{"ERD Number"=61646, "Data Type"=enum."string"}] ("Read ERD List")
            n676 = event-data() -> ()  [unwired: 1 in, 6 out]
            n677 = Concatenate Strings("Register", "FF" ("string")) -> (w2380:string)
            n678 = Bundle By Name(cluster=T52 {"ERD Number"=61646, "Data Type"=enum."string", "Data"=""} ("ERD Read Data In"), "Data"=w2380) -> (w2381:T52)
            n679 = Build Array(w2381) -> (w2368:T52[])
            n680 = call "Convert Write ERD List to Message.vi"("GEA Inputs"=w2366, "Write ERD List"=w2368, "Error In"=w2379) -> ("GEA Message"=w2384:T12, "Error Out"=w2385:errorcluster)  [unwired: 11 in]
            n681 = call "GEA2MessageFormatter.vi"("Prefix(Send/Recv)"="SEND", "GEA2 Data In"=w2384, "Error In"=w2385) -> ("Output String"=w2386:string, "Error Out"=w2387:errorcluster)  [unwired: 11 in]
            n682 = call "GExplorer_Queue_GEA2.vi"("Output String"=w2386, "error in (no error)"=w2387) -> ("error out"=w2369:errorcluster)  [unwired: 13 in]
            n683 = call "GEA3 Write ERD (Rev 2 API) Multiple Messages.vi"("GEA2 Reference In"=w2367, "GEA Inputs"=w2366, "Write ERD List"=w2368, "Error In"=w2369, "Verify ERD Response?"=FALSE) -> ("GEA2 Reference Out"=w2365:refnum<k24>)  [unwired: 8 in, 2 out]
            n684 = call "Convert Read ERD List to Message.vi"("GEA Inputs"=w2366, "Read ERD List"=w2372) -> ("GEA Message"=w2394:T12, "Error Out"=w2390:errorcluster)  [unwired: 12 in]
            n685 = call "GEA2MessageFormatter.vi"("Prefix(Send/Recv)"="SEND", "GEA2 Data In"=w2394, "Error In"=w2390) -> ("Output String"=w2392:string, "Error Out"=w2391:errorcluster)  [unwired: 11 in]
            n686 = call "GExplorer_Queue_GEA2.vi"("Output String"=w2392, "error in (no error)"=w2391) -> ("error out"=w2375:errorcluster)  [unwired: 13 in]
            n687 = call "GEA3 Read ERD (Rev 2 API) Multiple Messages.vi"("GEA2 Reference In"=w2365, "GEA Inputs"=w2366, "Read ERD List"=w2372, "Error In"=w2375, "Verify ERD Response?"=FALSE) -> ("GEA2 Reference Out"=w2371:refnum<k24>, "ERD Data Out"=w2373:cluster{"ERD Number":u16, "Data":string}[], "Error Out"=w2376:errorcluster)  [unwired: 7 in, 1 out]
            n688 = Index Array(array=w2373) -> (element=w2389:cluster{"ERD Number":u16, "Data":string})  [unwired: 1 in]
            n689 = Unbundle By Name(w2389) -> ("Data"=→"Value":string)
          }
          event "Data ON": Value Change {
            n690 = event-data() -> ()  [unwired: 1 in, 6 out]
            n691 = case shown="False" "Data ON" {
              tunnel: w2398 -> [w2401 w2405]
              tunnel: [w2400 w2404] -> w2397
              tunnel: w2395 -> [w2399 w2403]
              frame True {
                n692 = Enqueue Element(queue=w2399, element=T49 {"Data"=variant, "State"=enum."Init"} ("Data"), error in (no error)=w2401) -> (error out=w2400:errorcluster)  [unwired: 1 in, 2 out]
              }
              frame False {
                n693 = Enqueue Element(queue=w2403, element=T49 {"Data"=variant, "State"=enum."Pause"} ("Data"), error in (no error)=w2405) -> (error out=w2404:errorcluster)  [unwired: 1 in, 2 out]
              }
            }
          }
          event "Stop": Value Change; User Event; Panel Close {
            n694 = event-data() -> ()  [unwired: 1 in, 3 out]
            n695 = call "Control_ERD_Loop.vi"("Command (ERD Loop Control)"=ERD_Loop_Control_Command."Shutdown", "Error In"=w2415) -> ("Error Out"=w2414:errorcluster)  [unwired: 13 in]
            n696 = call "Control_GEA2_Loop.vi"("Command (ERD Loop Control)"=GEA2_Control_Command."Shutdown", "Error In"=w2414) -> ("Error Out"=w2416:errorcluster)  [unwired: 13 in]
            n697 = call "Control_DAQ_Loop.vi"("Command (DAQ Control)"=DAQ_Control_Command."Shutdown", "Error In"=w2416) -> ("Error Out"=w2419:errorcluster)  [unwired: 13 in]
            n698 = call "Control_Cont_Send.vi"("Command (ERD Loop Control)"=GEA2_Control_Command."Shutdown", "Error In"=w2419) -> ("Error Out"=w2409:errorcluster)  [unwired: 13 in]
            n699 = call "Time Delay8"("error in (no error)"=w2409, "Delay Time (s)"=2.0) -> ("error out"=w2408:errorcluster)  [unwired: 9 in]
          }
          event "Get Board SKU and Serial": Value Change {
            w2422 = T9[] [{"ERD Number"=61730, "Data Type"=enum."string"}, {"ERD Number"=61731, "Data Type"=enum."string"}] ("Read ERD List")
            n700 = event-data() -> ()  [unwired: 1 in, 6 out]
            n701 = call "Convert Read ERD List to Message.vi"("GEA Inputs"=w2423, "Read ERD List"=w2422, "Error In"=w2434) -> ("GEA Message"=w2439:T12, "Error Out"=w2435:errorcluster)  [unwired: 11 in]
            n702 = call "GEA2MessageFormatter.vi"("Prefix(Send/Recv)"="SEND", "GEA2 Data In"=w2439, "Error In"=w2435) -> ("Output String"=w2437:string, "Error Out"=w2436:errorcluster)  [unwired: 11 in]
            n703 = call "GExplorer_Queue_GEA2.vi"("Output String"=w2437, "error in (no error)"=w2436) -> ("error out"=w2421:errorcluster)  [unwired: 13 in]
            n704 = call "GEA3 Read ERD (Rev 2 API) Multiple Messages.vi"("GEA2 Reference In"=w2424, "Retry Count"=2, "Read Timeout (ms)"=u32 200, "GEA Inputs"=w2423, "Read ERD List"=w2422, "Error In"=w2421, "Verify ERD Response?"=FALSE) -> ("GEA2 Reference Out"=w2420:refnum<k24>, "ERD Data Out"=w2425:cluster{"ERD Number":u16, "Data":string}[], "Error Out"=w2427:errorcluster)  [unwired: 5 in, 1 out]
            n705 = Array To Cluster(array=w2425) -> (cluster=w2433:T58)
            n706 = Unbundle By Name(w2433) -> ("ERD Data Out[0].Data"=w2432:string)
            n707 = Unbundle By Name(w2433) -> ("ERD Data Out[0].Data"=w2431:string)
            n708 = call "String Remove All Spaces.vi"("Input String"=w2432) -> ("Spaces Removed"=w2458:string)  [unwired: 13 in, 1 out]
            n709 = call "String Remove All Spaces.vi"("Input String"=w2431) -> ("Spaces Removed"=w2449:string)  [unwired: 13 in, 1 out]
            n710 = call "HexString to AsciiString.vi"("Hex String"=w2458) -> ("ASCII String"=w2454:string)  [unwired: 13 in, 1 out]
            n711 = call "HexString to AsciiString.vi"("Hex String"=w2449) -> ("ASCII String"=w2445:string)  [unwired: 13 in, 1 out]
            n712 = Search and Replace String(replace all?=TRUE ("replace all? (F)"), input string=w2454, search string="ÿ", replace string="") -> (result string=w2451:string)  [unwired: 4 in, 3 out]
            n713 = Search and Replace String(replace all?=TRUE ("replace all? (F)"), input string=w2445, search string="ÿ", replace string="") -> (result string=w2442:string)  [unwired: 4 in, 3 out]
            n714 = Search and Replace String(replace all?=TRUE ("replace all? (F)"), input string=w2451, search string="r", replace string="") -> (result string=→"Board SKU":string)  [unwired: 4 in, 3 out]
            n715 = Search and Replace String(replace all?=TRUE ("replace all? (F)"), input string=w2442, search string="r", replace string="") -> (result string=→"Board Serial":string)  [unwired: 4 in, 3 out]
          }
          event "Get Wifi Data": Value Change {
            n716 = event-data() -> ()  [unwired: 1 in, 6 out]
            n717 = call "Wifi_Data.vi"("GEA2 Reference In"=w2466, "Error In"=w2465) -> ("Wifi Network State"=→"Wifi Network State":string, "GEA2 Reference Out"=w2464:refnum<k24>, "Mac Address"=→"Mac Address":string, "Wifi Network Name"=→"Wifi Network Name":string, "Wifi Password"=→"Wifi Password":string, "Error Out"=w2463:errorcluster)  [unwired: 8 in]
          }
          event "Turn on Wifi", "Turn off Wifi": Value Change {
            w2473 = T52 {"ERD Number"=61717, "Data Type"=enum."string", "Data"=""} ("ERD Read Data In")
            n718 = event-data() -> ()  [unwired: 1 in, 6 out]
            n719 = case shown="True" "Turn on Wifi" {
              tunnel: w2477 -> [w2498 w2505]
              tunnel: w2476 -> [w2499 w2504]
              tunnel: w2473 -> [_ w2503]
              tunnel: [w2499 w2501] -> w2472
              tunnel: [w2498 w2502] -> w2471
              tunnel: w2468 -> [w2497 w2500]
              tunnel: [w2497 w2500] -> w2467
              frame False {
              }
              frame True {
                n720 = Concatenate Strings("01" ("string")) -> (w2516:string)
                n721 = Bundle By Name(cluster=w2503, "Data"=w2516) -> (w2515:T52)
                n722 = Build Array(w2515) -> (w2506:T52[])
                n723 = call "Convert Write ERD List to Message.vi"("GEA Inputs"=w2500, "Write ERD List"=w2506, "Error In"=w2504) -> ("GEA Message"=w2510:T12, "Error Out"=w2511:errorcluster)  [unwired: 11 in]
                n724 = call "GEA2MessageFormatter.vi"("Prefix(Send/Recv)"="SEND", "GEA2 Data In"=w2510, "Error In"=w2511) -> ("Output String"=w2512:string, "Error Out"=w2513:errorcluster)  [unwired: 11 in]
                n725 = call "GExplorer_Queue_GEA2.vi"("Output String"=w2512, "error in (no error)"=w2513) -> ("error out"=w2509:errorcluster)  [unwired: 13 in]
                n726 = call "GEA2 Write ERD.vi"("GEA2 Reference In"=w2505, "GEA Inputs"=w2500, "Write ERD List"=w2506, "Error In"=w2509, "Verify ERD Response?"=FALSE) -> ("GEA2 Reference Out"=w2502:refnum<k24>, "Error Out"=w2501:errorcluster)  [unwired: 8 in, 1 out]
              }
            }
            n727 = case shown="True" "Turn off Wifi" {
              tunnel: w2471 -> [w2478 w2485]
              tunnel: w2472 -> [w2479 w2484]
              tunnel: w2473 -> [_ w2483]
              tunnel: [w2479 w2481] -> w2469
              tunnel: [w2478 w2482] -> w2470
              tunnel: w2467 -> [_ w2480]
              frame False {
              }
              frame True {
                n728 = Concatenate Strings("02" ("string")) -> (w2496:string)
                n729 = Bundle By Name(cluster=w2483, "Data"=w2496) -> (w2495:T52)
                n730 = Build Array(w2495) -> (w2486:T52[])
                n731 = call "Convert Write ERD List to Message.vi"("GEA Inputs"=w2480, "Write ERD List"=w2486, "Error In"=w2484) -> ("GEA Message"=w2490:T12, "Error Out"=w2491:errorcluster)  [unwired: 11 in]
                n732 = call "GEA2MessageFormatter.vi"("Prefix(Send/Recv)"="SEND", "GEA2 Data In"=w2490, "Error In"=w2491) -> ("Output String"=w2492:string, "Error Out"=w2493:errorcluster)  [unwired: 11 in]
                n733 = call "GExplorer_Queue_GEA2.vi"("Output String"=w2492, "error in (no error)"=w2493) -> ("error out"=w2489:errorcluster)  [unwired: 13 in]
                n734 = call "GEA2 Write ERD.vi"("GEA2 Reference In"=w2485, "GEA Inputs"=w2480, "Write ERD List"=w2486, "Error In"=w2489, "Verify ERD Response?"=FALSE) -> ("GEA2 Reference Out"=w2482:refnum<k24>, "Error Out"=w2481:errorcluster)  [unwired: 8 in, 1 out]
              }
            }
          }
          event "Get Snapshot": Value Change {
            n735 = event-data() -> ()  [unwired: 1 in, 6 out]
            n736 = call "TL27_Get_Single_Fault_Snapshot.vi"("GEA2 Reference In"=w2520, "Snapshot Selection"="Select Snapshot", "Error In"=w2521) -> ("GEA2 Reference Out"=w2518:refnum<k24>, "Fault Snapshots"=→"Fault Snapshots":T22, "Error Out"=w2519:errorcluster)  [unwired: 10 in]
          }
          event "Get Snapshot Status": Value Change {
            n737 = event-data() -> ()  [unwired: 1 in, 6 out]
            n738 = call "TL27_Snapshot_Status.vi"("GEA2 Reference In"=w2529, "Error In"=w2528) -> ("GEA2 Reference Out"=w2527:refnum<k24>, "Current Index"=→"Current Index":u16, "Count"=→"Count":u16, "Overwrite Count"=→"Overwrite Count":u16, "Error Out"=w2526:errorcluster)  [unwired: 9 in]
          }
          event "Clear Snapshots": Value Change {
            w2530 = T52[] [{"ERD Number"=61772, "Data Type"=enum."string", "Data"="01"}] ("Write ERD List")
            n739 = event-data() -> ()  [unwired: 1 in, 6 out]
            n740 = call "Convert Write ERD List to Message.vi"("GEA Inputs"=w2534, "Write ERD List"=w2530, "Error In"=w2536) -> ("GEA Message"=w2538:T12, "Error Out"=w2539:errorcluster)  [unwired: 11 in]
            n741 = call "GEA2MessageFormatter.vi"("Prefix(Send/Recv)"="SEND", "GEA2 Data In"=w2538, "Error In"=w2539) -> ("Output String"=w2540:string, "Error Out"=w2541:errorcluster)  [unwired: 11 in]
            n742 = call "GExplorer_Queue_GEA2.vi"("Output String"=w2540, "error in (no error)"=w2541) -> ("error out"=w2535:errorcluster)  [unwired: 13 in]
            n743 = call "GEA2 Write ERD.vi"("GEA2 Reference In"=w2533, "GEA Inputs"=w2534, "Write ERD List"=w2530, "Error In"=w2535) -> ("GEA2 Reference Out"=w2532:refnum<k24>, "Error Out"=w2531:errorcluster)  [unwired: 9 in, 1 out]
          }
          event "Set Wifi State(ERD 6003)", "Wifi State": Value Change {
            n744 = event-data() -> ()  [unwired: 1 in, 6 out]
            n745 = case shown="\"255 - Invalid\"" "Wifi State" {
              tunnel: ["00" "01" "02" "03" "04" "05" "06" "FF"] -> w2545
              frame "0 - OFF", Default {
              }
              frame "1 - App Mode" {
              }
              frame "2 - Connecting" {
              }
              frame "3 - Connected" {
              }
              frame "4 - Connected Off" {
              }
              frame "5 - Scanning" {
              }
              frame "6 - Reconnecting" {
              }
              frame "255 - Invalid" {
              }
            }
            n746 = case shown="False" "Set Wifi State(ERD 6003)" {
              tunnel: w2543 -> [w2547 w2552]
              tunnel: w2542 -> [w2548 w2556]
              tunnel: [w2548 w2554] -> _
              tunnel: [w2547 w2555] -> _
              tunnel: w2545 -> [_ w2553]
              frame False {
              }
              frame True {
                w2549 = T10 {"Source"=228, "Destination"=191} ("GEA Inputs")
                n747 = Concatenate Strings(w2553) -> (w2565:string)
                n748 = Bundle By Name(cluster=T52 {"ERD Number"=24579, "Data Type"=enum."string", "Data"=""} ("ERD Write Data In"), "Data"=w2565) -> (w2564:T52)
                n749 = Build Array(w2564) -> (w2550:T52[])
                n750 = call "Convert Write ERD List to Message.vi"("GEA Inputs"=w2549, "Write ERD List"=w2550, "Error In"=w2556) -> ("GEA Message"=w2560:T12, "Error Out"=w2561:errorcluster)  [unwired: 11 in]
                n751 = call "GEA2MessageFormatter.vi"("Prefix(Send/Recv)"="SEND", "GEA2 Data In"=w2560, "Error In"=w2561) -> ("Output String"=w2562:string, "Error Out"=w2563:errorcluster)  [unwired: 11 in]
                n752 = call "GExplorer_Queue_GEA2.vi"("Output String"=w2562, "error in (no error)"=w2563) -> ("error out"=w2559:errorcluster)  [unwired: 13 in]
                n753 = call "GEA2 Write ERD.vi"("GEA2 Reference In"=w2552, "GEA Inputs"=w2549, "Write ERD List"=w2550, "Error In"=w2559, "Verify ERD Response?"=FALSE) -> ("GEA2 Reference Out"=w2555:refnum<k24>, "Error Out"=w2554:errorcluster)  [unwired: 8 in, 1 out]
              }
            }
          }
          event "Set Price": Value Change {
            (unwired) T52 {"ERD Number"=65363, "Data Type"=enum."string", "Data"=""} ("ERD Read Data In")
            n754 = event-data() -> ()  [unwired: 1 in, 6 out]
            n755 = call "SetBasePrices_Washer.vi"("error in"=w2582, "BasePrices"="BasePrices") -> ("error out"=w2583:errorcluster, "PriceData"=w2576:string)  [unwired: 8 in]
            n756 = Bundle By Name(cluster=T52 {"ERD Number"=65384, "Data Type"=enum."string", "Data"=""} ("ERD Read Data In"), "Data"=w2576) -> (w2579:T52)
            n757 = Build Array(w2579) -> (w2578:T52[])
            n758 = call "GEA3 Write ERD (Rev 2 API) Multiple Messages.vi"("GEA2 Reference In"=w2584, "GEA Inputs"=w2577, "Write ERD List"=w2578, "Error In"=w2583) -> ("GEA2 Reference Out"=w2575:refnum<k24>, "Error Out"=w2574:errorcluster)  [unwired: 9 in, 1 out]
          }
          event "SetIncrementPrices": Value Change {
            (unwired) T52 {"ERD Number"=65364, "Data Type"=enum."string", "Data"=""} ("ERD Read Data In")
            n759 = event-data() -> ()  [unwired: 1 in, 6 out]
            n760 = call "SetBasePrices_Washer.vi"("error in"=w2588, "BasePrices"="IncrementPrice") -> ("error out"=w2595:errorcluster, "PriceData"=w2591:string)  [unwired: 8 in]
            n761 = Bundle By Name(cluster=T52 {"ERD Number"=65385, "Data Type"=enum."string", "Data"=""} ("ERD Read Data In"), "Data"=w2591) -> (w2593:T52)
            n762 = Build Array(w2593) -> (w2592:T52[])
            n763 = call "GEA3 Write ERD (Rev 2 API) Multiple Messages.vi"("GEA2 Reference In"=w2589, "GEA Inputs"=w2587, "Write ERD List"=w2592, "Error In"=w2595) -> ("GEA2 Reference Out"=w2586:refnum<k24>, "Error Out"=w2585:errorcluster)  [unwired: 9 in, 1 out]
          }
          event "Phase.Idle": Value Change {
            n764 = event-data() -> ()  [unwired: 1 in, 1 out]
            n765 = Bundle By Name(cluster=T52 {"ERD Number"=8350, "Data Type"=enum."string", "Data"=""} ("ERD Write Data In"), "Data"="FF FF FF FF 00 02 00 03 FF FF FF FF FF FF FF FF FF FF FF FF FF FF FF FF FF FF FF FF 83 FF FF FF") -> (w2603:T52)
            n766 = Build Array(w2603) -> (w2602:T52[])
            n767 = call "GEA3 Write ERD (Rev 2 API) Multiple Messages.vi"("GEA2 Reference In"=w2599, "GEA Inputs"=w2598, "Write ERD List"=w2602, "Error In"=w2600) -> ("GEA2 Reference Out"=w2597:refnum<k24>, "Error Out"=w2596:errorcluster)  [unwired: 9 in, 1 out]
          }
          event "Phase.Reserved": Value Change {
            n768 = event-data() -> ()  [unwired: 1 in, 1 out]
            n769 = Bundle By Name(cluster=T52 {"ERD Number"=8350, "Data Type"=enum."string", "Data"=""} ("ERD Write Data In"), "Data"="FF FF FF FF 01 02 00 03 FF FF FF FF FF FF FF FF FF FF FF FF FF FF FF FF FF FF FF FF 83 FF FF FF") -> (w2612:T52)
            n770 = Build Array(w2612) -> (w2611:T52[])
            n771 = call "GEA3 Write ERD (Rev 2 API) Multiple Messages.vi"("GEA2 Reference In"=w2610, "GEA Inputs"=w2608, "Write ERD List"=w2611, "Error In"=w2609) -> ("GEA2 Reference Out"=w2607:refnum<k24>, "Error Out"=w2606:errorcluster)  [unwired: 9 in, 1 out]
          }
          event "Phase.Authorized": Value Change {
            n772 = event-data() -> ()  [unwired: 1 in, 1 out]
            n773 = call "GEA3 Read ERD (Rev 2 API) Multiple Messages.vi"("GEA2 Reference In"=w2621, "Retry Count"=2, "GEA Inputs"=w2617, "Read ERD List"=cluster{"ERD Number":u16, "Data Type":T7}[] [{"ERD Number"=8351, "Data Type"=enum."string"}], "Error In"=w2620, "Verify ERD Response?"=TRUE) -> ("GEA2 Reference Out"=w2616:refnum<k24>, "ERD Data Out"=w2630:cluster{"ERD Number":u16, "Data":string}[], "Error Out"=w2619:errorcluster)  [unwired: 6 in, 1 out]
            n774 = Array To Cluster(array=w2630) -> (cluster=w2629:T58)
            n775 = Unbundle By Name(w2629) -> ("ERD Data Out[0].Data"=w2628:string)
            n776 = Search and Replace String(input string=w2628, search string="02", replace string="06" ("replace string (\"\")"), offset=4 ("offset (0)")) -> (result string=w2624:string)  [unwired: 4 in, 3 out]
            n777 = Bundle By Name(cluster=T52 {"ERD Number"=8350, "Data Type"=enum."string", "Data"=""} ("ERD Write Data In"), "Data"=w2624) -> (w2623:T52)
            n778 = Build Array(w2623) -> (w2618:T52[])
            n779 = call "GEA3 Write ERD (Rev 2 API) Multiple Messages.vi"("GEA2 Reference In"=w2616, "GEA Inputs"=w2617, "Write ERD List"=w2618, "Error In"=w2619) -> ("GEA2 Reference Out"=w2615:refnum<k24>, "Error Out"=w2614:errorcluster)  [unwired: 9 in, 1 out]
          }
          event "EndofCycle": Value Change {
            n780 = event-data() -> ()  [unwired: 1 in, 1 out]
            n781 = call "GEA3 Write ERD (Rev 2 API) Multiple Messages.vi"("GEA2 Reference In"=w2647, "GEA Inputs"=w2634, "Write ERD List"=T52[] [{"ERD Number"=61895, "Data Type"=enum."string", "Data"="02"}], "Error In"=w2646) -> ("GEA2 Reference Out"=w2635:refnum<k24>, "Error Out"=w2637:errorcluster)  [unwired: 9 in, 1 out]
            n782 = call "Time Delay11"("error in (no error)"=w2637, "Delay Time (s)"=3.0) -> ("error out"=w2636:errorcluster)  [unwired: 9 in]
            n783 = Bundle By Name(cluster=T52 {"ERD Number"=8350, "Data Type"=enum."string", "Data"=""} ("ERD Write Data In"), "Data"="FF FF FF FF 00 02 00 03 FF FF FF FF FF FF FF FF FF FF FF FF FF FF FF FF FF FF FF FF 83 FF FF FF") -> (w2643:T52)
            n784 = Build Array(w2643) -> (w2642:T52[])
            n785 = call "GEA3 Write ERD (Rev 2 API) Multiple Messages.vi"("GEA2 Reference In"=w2635, "GEA Inputs"=w2634, "Write ERD List"=w2642, "Error In"=w2636) -> ("GEA2 Reference Out"=w2640:refnum<k24>, "Error Out"=w2639:errorcluster)  [unwired: 9 in, 1 out]
          }
        }
        n786 = call "Error_Control.vi"("Error In"=w1097) -> ("Error Out"=w1099:errorcluster)  [unwired: 14 in]
      }
      n787 = while "DAQ Loop" {
        shift-right: [w571] -> w104
        shift-left: w29 -> [w569]
        shift-right: [w548] -> _
        shift-left: DAQ_States."Wait for Init" ("States") -> [w566]
        shift-right: [w549] -> _
        shift-left: "Wait for Init" ("Report Text") -> [w564]
        tunnel: w65 -> [w565]
        shift-right: [w547] -> _
        shift-left: _ -> [w506]
        shift-right: [w546] -> _
        shift-left: FALSE -> [w545]
        shift-right: [w536] -> _
        shift-left: w57 -> [w535]
        shift-right: [w534] -> _
        shift-left: w57 -> [w533]
        shift-right: [w532] -> _
        shift-left: w57 -> [w531]
        shift-right: [w530] -> _
        shift-left: w57 -> [w529]
        shift-right: [w528] -> _
        shift-left: w57 -> [w527]
        shift-right: [w526] -> _
        shift-left: w57 -> [w525]
        shift-right: [w524] -> _
        shift-left: w57 -> [w523]
        shift-right: [w501] -> _
        shift-left: 1.0 -> [w507]
        shift-right: [w510] -> _
        shift-left: 1.0 -> [w513]
        shift-right: [w509] -> _
        shift-left: 0.0 -> [w512]
        shift-right: [w505] -> _
        shift-left: w57 -> [w504]
        shift-right: [w503] -> _
        shift-left: FALSE -> [w537]
        stop <- w561 stop-if-true
        # "Automatic Modeshift Feedback"
        # "DAQ Loop"
        n788 = Greater?(x=w513, y=5.0 ("x")) -> (0:w515:bool)
        n789 = Dequeue Element(queue=w565, timeout in ms (-1)=0, error in (no error)=w569) -> (element=w567:T48, timed out?=w568:bool, error out=w560:errorcluster)  [unwired: 1 out]
        n790 = Wait (ms)(milliseconds to wait=u32 250) -> ()  [unwired: 1 out]
        n791 = Select(t="Basket RPM", s=w515, f=w507) -> (s? t:f=w501:dbl)
        n792 = Select(t=w566, s=w568, f=w567) -> (s? t:f=w563:T48)
        n793 = Multiply(x=0.40625 ("y"), y=w501) -> (x*y=w541:dbl)
        n794 = Less?(x=w501, y=1.0) -> (x < y?=w539:bool)
        n795 = Equal?(x=w507, y=w501) -> (x = y?=w538:bool)
        n796 = case shown="\"Run\"" w563 {
          selector: w563 -> [_ _ _ _ _ _ w1050]
          tunnel: [_ _ _ w763 w883 _ _] -> w505
          tunnel: [w603 w627 w659 w764 w881 w988 w1053] -> w557
          tunnel: w523 -> [w618 w642 w667 _ w880 w982 w999]
          tunnel: [w618 w642 w667 w768 w879 _ _] -> w524
          tunnel: w525 -> [w617 w641 w668 _ w878 w979 w1026]
          tunnel: [w617 w641 w668 w772 w877 _ _] -> w526
          tunnel: [w601 w625 w651 w771 w876 w942 w1016] -> w555
          tunnel: [w602 w626 w652 w767 w875 w949 w1028] -> w556
          tunnel: [w612 DAQ_States."Verify Hardware" ("t") w664 DAQ_States."Run" ("t") w853 DAQ_States."Wait for Init" ("States") w1050] -> w548
          tunnel: [FALSE FALSE FALSE TRUE TRUE FALSE FALSE] -> w547
          tunnel: w531 -> [w616 w640 w671 _ w838 w986 w1055]
          tunnel: [w598 w622 w648 w760 w872 w935 w1013] -> w552
          tunnel: [w616 w640 w671 w761 w873 _ _] -> w532
          tunnel: [w599 w623 w649 w724 w863 w974 w1054] -> w553
          tunnel: w529 -> [w615 w639 w670 _ w862 w985 w1049]
          tunnel: [w615 w639 w670 w729 w864 _ _] -> w530
          tunnel: [_ _ _ _ _ FALSE TRUE] -> w561
          tunnel: [_ _ _ _ w871 _ _] -> w522
          tunnel: [_ _ _ _ w865 _ _] -> w508
          tunnel: [_ _ _ _ w870 _ _] -> w521
          tunnel: [_ _ _ _ w869 _ _] -> w520
          tunnel: [_ _ _ _ w868 _ _] -> w519
          tunnel: [_ _ _ _ w867 _ _] -> w518
          tunnel: [_ _ _ _ w866 _ _] -> w517
          tunnel: [w600 w624 w650 w721 w861 w972 w1047] -> w554
          tunnel: [w614 w638 w669 w718 w859 _ _] -> w528
          tunnel: w527 -> [w614 w638 w669 _ w860 w973 w1048]
          tunnel: [_ _ _ _ w858 _ _] -> w544
          tunnel: [_ _ _ _ w857 _ _] -> w543
          tunnel: [w613 w637 w661 "Initialize" ("Report Text") "Running" ("Report Text") "Wait for Init" ("Report Text") "Exit" ("Report Text")] -> w549
          tunnel: w564 -> [w613 w637 _ _ _ _ _]
          tunnel: [w597 w621 w647 w702 w845 w966 w1044] -> w551
          tunnel: [w608 w635 w657 w699 w844 _ _] -> w534
          tunnel: [w607 w634 w656 w697 w842 _ _] -> w536
          tunnel: [w596 w620 w646 w696 w843 w965 w991] -> w550
          tunnel: w533 -> [w608 w635 w657 _ w846 w967 w1045]
          tunnel: w535 -> [w607 w634 w656 _ w841 w963 w1011]
          tunnel: [w595 w619 w645 w676 w840 FALSE FALSE] -> w546
          tunnel: [FALSE FALSE FALSE FALSE w830 FALSE FALSE] -> w503
          tunnel: [w604 w630 w654 w683 w829 w958 w1041] -> w558
          tunnel: "Turn On DAQ" -> [w605 _ _ _ w805 _ _]
          tunnel: w560 -> [w603 w627 w653 w685 w828 w957 w1040]
          tunnel: w560 -> [w602 w626 w652 w684 w823 w955 w1002]
          tunnel: w560 -> [w604 w629 w654 w683 w829 w958 w1041]
          tunnel: w560 -> [w601 w625 w651 w682 w821 w940 w1025]
          tunnel: w560 -> [w600 w624 w650 w681 w820 w939 w1039]
          tunnel: w560 -> [w599 w623 w649 w680 w817 w938 w1038]
          tunnel: w560 -> [w598 w622 w648 w679 w816 w937 w1037]
          tunnel: w560 -> [w597 w621 w647 w678 w810 w933 w1036]
          tunnel: w560 -> [w596 w620 w646 w677 w806 w932 w1010]
          tunnel: w545 -> [w595 w619 w645 w676 w809 _ _]
          tunnel: w541 -> [_ _ _ _ w815 _ _]
          tunnel: 0.5 ("Duty Cycle") -> [_ _ _ _ w814 _ _]
          tunnel: w539 -> [_ _ _ _ w812 _ _]
          tunnel: w538 -> [_ _ _ _ w813 _ _]
          tunnel: w537 -> [_ _ _ _ w811 _ _]
          tunnel: w506 -> [_ _ _ _ _ _ w1035]
          tunnel: w504 -> [_ _ _ _ w804 w931 w1034]
          frame "Wait for Init", Default {
            # "Hall Sensor"
            # "Motor TRIAC CCW"
            # "Motor TRIAC CW"
            # "Relay Controls"
            # "TRIAC Outputs"
            # "AO for ADC"
            n797 = Select(t=DAQ_States."Rename Devices", s=w605, f=DAQ_States."Wait for Init" ("States")) -> (s? t:f=w612:T48)
          }
          frame "Rename Devices" {
            # "Hall Sensor"
            # "Motor TRIAC CCW"
            # "Motor TRIAC CW"
            # "Relay Controls"
            # "TRIAC Outputs"
            n798 = case shown="\"LE\"" "HE/LE ?" {
              tunnel: ["VALEW_HE" "VALEW_LE"] -> w631
              frame "HE", Default {
              }
              frame "LE" {
              }
            }
            n799 = call "VALEW_Rename DAQmx Devices.vi"("cDAQ Name"=w631, "Error In"=w629) -> ("Error Out"=w630:errorcluster)  [unwired: 13 in]
          }
          frame "Verify Hardware" {
            n800 = call "DeviceListCheck.vi"("Device List"=string[] ["9481_1", "9435_1", "9435_2", "9401_1", "9269_1"], "Error In"=w653) -> ("Devices Present?"=w658:bool, "Report Text"=w661:string, "Error Out"=w660:errorcluster)  [unwired: 11 in]
            n801 = case shown="False" w658 {
              selector: w658 -> [w673 _]
              tunnel: w660 -> [w674 w675]
              tunnel: [w672 w675] -> w659
              frame False {
                n802 = property on="Turn On DAQ" class="Bool (strict)"(error in=w674, "Value"=w673) -> (error out=w672:errorcluster)  [unwired: 1 in, 1 out]
              }
              frame True {
              }
            }
            n803 = Select(t=DAQ_States."Initialize" ("f"), s=w658, f=DAQ_States."Wait for Init") -> (s? t:f=w664:T48)
          }
          frame "Initialize" {
            w690 = 4 items=["verify"=2, "reserve"=4, "commit"=3, "unreserve"=5, "abort"=6] ("action")
            w706 = 10123 items=["Finite Samples"=10178, "Continuous Samples"=10123, "Hardware Timed Single Point"=12522] ("sample mode")
            w709 = 4 items=["verify"=2, "reserve"=4, "commit"=3, "unreserve"=5, "abort"=6] ("action")
            w742 = 4 items=["verify"=2, "reserve"=4, "commit"=3, "unreserve"=5, "abort"=6] ("action")
            w743 = 4 items=["verify"=2, "reserve"=4, "commit"=3, "unreserve"=5, "abort"=6] ("action")
            w757 = 10123 items=["Finite Samples"=10178, "Continuous Samples"=10123, "Hardware Timed Single Point"=12522] ("sample mode")
            w765 = 0 items=["one channel for each line", "one channel for all lines"] ("line grouping")
            w770 = 0 items=["one channel for each line", "one channel for all lines"] ("line grouping")
            w773 = 0.0  # minimum value
            w774 = 5.0  # maximum value
            # "Hall Sensor"
            # "Motor TRIAC CCW"
            # "Motor TRIAC CW"
            # "Relay Controls"
            # "TRIAC Outputs"
            # "AO for ADC"
            n804 = call <vilib>:"DAQmx Create Task.vi"("auto cleanup"=TRUE, "error in"=w679) -> ("task out"=w731:refnum<k21>, "error out"=w732:errorcluster)  [unwired: 12 in]
            n805 = call <vilib>:"DAQmx Create Task.vi"("auto cleanup"=TRUE, "error in"=w678) -> ("task out"=w705:refnum<k21>, "error out"=w704:errorcluster)  [unwired: 12 in]
            n806 = call <vilib>:"DAQmx Create Task.vi"("auto cleanup"=TRUE, "error in"=w681) -> ("task out"=w739:refnum<k21>, "error out"=w740:errorcluster)  [unwired: 12 in]
            n807 = call <vilib>:"DAQmx Create Task.vi"("auto cleanup"=TRUE, "error in"=w680) -> ("task out"=w737:refnum<k21>, "error out"=w738:errorcluster)  [unwired: 12 in]
            n808 = call-poly <vilib>:"DAQmx Create Virtual Channel.vi"("task in"=w731, "counter"=tag "9401_1/ctr2", "error in"=w732) -> ("task out"=w734:refnum<k21>, "error out"=w762:errorcluster)  [unwired: 11 in]
            n809 = call-poly <vilib>:"DAQmx Create Virtual Channel.vi"("task in"=w739, "counter"=tag "9401_1/ctr0", "error in"=w740) -> ("task out"=w752:refnum<k21>, "error out"=w748:errorcluster)  [unwired: 11 in]
            n810 = call-poly <vilib>:"DAQmx Create Virtual Channel.vi"("task in"=w737, "counter"=tag "9401_1/ctr1", "error in"=w738) -> ("task out"=w751:refnum<k21>, "error out"=w750:errorcluster)  [unwired: 11 in]
            n811 = call-poly <vilib>:"DAQmx Create Virtual Channel.vi"("task in"=w705, "lines"=tag "9401_1/port0/line2", "error in"=w704) -> ("task out"=w711:refnum<k21>, "error out"=w712:errorcluster)  [unwired: 11 in]
            n812 = property class="DAQmx Channel"(reference=w734, error in=w762, "CO.Pulse.Term"=tag "/9401_1/PFI4") -> (reference out=w759:refnum<k21>, error out=w758:errorcluster)
            n813 = call-poly <vilib>:"DAQmx Create Virtual Channel.vi"("lines"=tag "9481_1/port0/line3", "error in"=w677) -> ("task out"=w697:refnum<k21>, "error out"=w696:errorcluster)  [unwired: 12 in]
            n814 = property class="DAQmx Channel"(reference=w752, error in=w748, "CI.CountEdges.Term"=tag "/9401_1/PFI0") -> (reference out=w747:refnum<k21>, error out=w746:errorcluster)
            n815 = property class="DAQmx Channel"(reference=w751, error in=w750, "CI.CountEdges.Term"=tag "/9401_1/PFI1") -> (reference out=w745:refnum<k21>, error out=w744:errorcluster)
            n816 = call-poly <vilib>:"DAQmx Create Virtual Channel.vi"("lines"=tag "9481_1/port0/line0:2", "name to assign"="Relay Outputs", "line grouping"=w770, "error in"=w684) -> ("task out"=w768:refnum<k21>, "error out"=w767:errorcluster)  [unwired: 10 in]
            n817 = call-poly <vilib>:"DAQmx Create Virtual Channel.vi"("lines"=tag "9435_1/port0/line0:2, 9435_2/port0/line0:3", "name to assign"="Outputs", "line grouping"=w765, "error in"=w685) -> ("task out"=w763:refnum<k21>, "error out"=w764:errorcluster)  [unwired: 10 in]
            n818 = call-poly <vilib>:"DAQmx Create Virtual Channel.vi"("maximum value"=w774, "minimum value"=w773, "physical channels"=tag "9269_1/ao0:2" ("lines"), "name to assign"="AO for ADC", "error in"=w682) -> ("task out"=w772:refnum<k21>, "error out"=w771:errorcluster)  [unwired: 9 in]
            n819 = call-poly <vilib>:"DAQmx Timing.vi"("task/channels in"=w711, "sample mode"=w706, "rate"=1000.0, "error in"=w712) -> ("task out"=w707:refnum<k21>, "error out"=w708:errorcluster)  [unwired: 10 in]
            n820 = call-poly <vilib>:"DAQmx Timing.vi"("task/channels in"=w759, "sample mode"=w757, "error in"=w758) -> ("task out"=w689:refnum<k21>, "error out"=w686:errorcluster)  [unwired: 11 in]
            n821 = call <vilib>:"DAQmx Control Task.vi"("task/channels in"=w747, "action"=w742, "error in"=w746) -> ("task out"=w720:refnum<k21>, "error out"=w723:errorcluster)  [unwired: 11 in]
            n822 = call <vilib>:"DAQmx Control Task.vi"("task/channels in"=w745, "action"=w743, "error in"=w744) -> ("task out"=w728:refnum<k21>, "error out"=w726:errorcluster)  [unwired: 11 in]
            n823 = call <vilib>:"DAQmx Control Task.vi"("task/channels in"=w689, "action"=w690, "error in"=w686) -> ("task out"=w688:refnum<k21>, "error out"=w687:errorcluster)  [unwired: 11 in]
            n824 = call <vilib>:"DAQmx Control Task.vi"("task/channels in"=w707, "action"=w709, "error in"=w708) -> ("task out"=w700:refnum<k21>, "error out"=w701:errorcluster)  [unwired: 11 in]
            n825 = flat-sequence {
              tunnel: w688 -> [w778]
              tunnel: w687 -> [w777]
              tunnel: w728 -> [w786]
              tunnel: [w786] -> w727
              tunnel: w726 -> [w785]
              tunnel: [w785] -> w725
              tunnel: w723 -> [w784]
              tunnel: [w784] -> w722
              tunnel: w720 -> [w783]
              tunnel: [w783] -> w719
              tunnel: w701 -> [w781]
              tunnel: w700 -> [w782]
              tunnel: [w780] -> w694
              tunnel: [w779] -> w693
              tunnel: [w778] -> w692
              tunnel: [w777] -> w691
              tunnel: [w790] -> w760
              tunnel: [w789] -> w761
              tunnel: [w800] -> w729
              tunnel: w727 -> [w799]
              tunnel: w725 -> [w798]
              tunnel: [w797] -> w724
              tunnel: w722 -> [w796]
              tunnel: [w795] -> w721
              tunnel: w719 -> [w794]
              tunnel: [w793] -> w718
              tunnel: [w792] -> w702
              tunnel: [w791] -> w699
              tunnel: w694 -> [w792]
              tunnel: w693 -> [w791]
              tunnel: w692 -> [w788]
              tunnel: w691 -> [w787]
              frame #0 {
                n826 = call <vilib>:"DAQmx Start Task.vi"("task/channels in"=w782, "error in"=w781) -> ("task out"=w779:refnum<k21>, "error out"=w780:errorcluster)  [unwired: 12 in]
              }
              frame #1 {
                n827 = call <vilib>:"DAQmx Start Task.vi"("task/channels in"=w794, "error in"=w796) -> ("task out"=w793:refnum<k21>, "error out"=w795:errorcluster)  [unwired: 12 in]
                n828 = call <vilib>:"DAQmx Start Task.vi"("task/channels in"=w799, "error in"=w798) -> ("task out"=w800:refnum<k21>, "error out"=w797:errorcluster)  [unwired: 12 in]
                n829 = call <vilib>:"DAQmx Start Task.vi"("task/channels in"=w788, "error in"=w787) -> ("task out"=w789:refnum<k21>, "error out"=w790:errorcluster)  [unwired: 12 in]
              }
            }
          }
          frame "Run" {
            # "Lid Lock Feedback"
            # "Is the task stopped?"
            # "Hall Sensor"
            # "Motor TRIAC CCW"
            # "Motor TRIAC CW"
            # "AO for ADC"
            # "Relay Controls"
            # "TRIAC Outputs"
            n830 = case shown="True" w812 {
              tunnel: w838 -> [w917 w922]
              tunnel: [w917 w921] -> w836
              tunnel: [w916 w920] -> w837
              tunnel: [w915 TRUE] -> w831
              tunnel: w816 -> [w916 w918]
              tunnel: w811 -> [w915 _]
              frame False {
              }
              frame True {
                n831 = call <vilib>:"DAQmx Stop Task.vi"("task/channels in"=w922, "error in"=w918) -> ("task out"=w921:refnum<k21>, "error out"=w920:errorcluster)  [unwired: 12 in]
              }
            }
            n832 = call-poly <vilib>:"DAQmx Read.vi"("task/channels in"=w846, "number of samples per channel"=-1, "timeout"=10.0, "error in"=w810) -> ("task out"=w844:refnum<k21>, "data"=w850:u8[], "error out"=w845:errorcluster)  [unwired: 9 in]
            n833 = Compound Arithmetic op=AND(w831, invert w812) -> (w833:bool)
            n834 = case shown="False" w833 {
              tunnel: w837 -> [w907 w911]
              tunnel: w836 -> [w908 w910]
              tunnel: [w908 w914] -> w835
              tunnel: [w907 w913] -> w834
              tunnel: w831 -> [w906 _]
              tunnel: [w906 FALSE] -> w830
              frame False {
              }
              frame True {
                n835 = call <vilib>:"DAQmx Start Task.vi"("task/channels in"=w910, "error in"=w911) -> ("task out"=w914:refnum<k21>, "error out"=w913:errorcluster)  [unwired: 12 in]
                n836 = Wait (ms)(milliseconds to wait=u32 1200) -> ()  [unwired: 1 out]
              }
            }
            n837 = Build Array("AC Power", "Mode Shift FB", "Lid Status") -> (w824:bool[])
            n838 = Build Array("Pressure", "Motor Current", "Temperature") -> (w822:dbl[])
            n839 = Search 1D Array(1D array=w850, element=u8 4) -> (index of element=w848:i32)  [unwired: 1 in]
            n840 = Equal?(x=w848, y=-1) -> (x = y?=w839:bool)
            n841 = Compound Arithmetic op=OR(w812, w813) -> (w832:bool)
            n842 = call-poly <vilib>:"DAQmx Read.vi"("task/channels in"=w804, "error in"=w828) -> ("task out"=w883:refnum<k21>, "data"=w882:bool[], "error out"=w881:errorcluster)  [unwired: 11 in]
            n843 = call-poly <vilib>:"DAQmx Write.vi"("task/channels in"=w880, "data"=w824, "error in"=w823) -> ("task out"=w879:refnum<k21>, "error out"=w875:errorcluster)  [unwired: 10 in, 1 out]
            n844 = call-poly <vilib>:"DAQmx Write.vi"("task/channels in"=w878, "data"=w822, "error in"=w821) -> ("task out"=w877:refnum<k21>, "error out"=w876:errorcluster)  [unwired: 10 in, 1 out]
            n845 = call-poly <vilib>:"DAQmx Read.vi"("task/channels in"=w860, "error in"=w820) -> ("task out"=w859:refnum<k21>, "data"=w819:u32, "error out"=w861:errorcluster)  [unwired: 11 in]
            "CW" <- w819
            n846 = call-poly <vilib>:"DAQmx Read.vi"("task/channels in"=w862, "error in"=w817) -> ("task out"=w864:refnum<k21>, "data"=w818:u32, "error out"=w863:errorcluster)  [unwired: 11 in]
            "CCW" <- w818
            n847 = case shown="True" "LL (M - A)" {
              tunnel: [w886 w896] -> w843
              tunnel: [w887 w895] -> w842
              tunnel: w841 -> [w889 w894]
              tunnel: [w885 w893] -> w840
              tunnel: w839 -> [_ w892]
              tunnel: "Lid Lock Feedback" -> [w888 _]
              tunnel: w809 -> [w885 w891]
              tunnel: w806 -> [w884 w890]
              frame False {
                n848 = call-poly <vilib>:"DAQmx Write.vi"("task/channels in"=w889, "data"=w888, "error in"=w884) -> ("task out"=w887:refnum<k21>, "error out"=w886:errorcluster)  [unwired: 10 in, 1 out]
              }
              frame True {
                # "Automatic Lid Lock feedback"
                n849 = case shown="True" w892 {
                  tunnel: w894 -> [w902 w905]
                  tunnel: [w901 w904] -> w896
                  tunnel: [w900 w905] -> w895
                  tunnel: [w899 w903] -> w893
                  tunnel: w891 -> [w898 w903]
                  tunnel: w890 -> [w897 w904]
                  frame False {
                    n850 = Not(x=w898) -> (.not. x?=w899:bool)
                    n851 = call-poly <vilib>:"DAQmx Write.vi"("task/channels in"=w902, "data"=w899, "error in"=w897) -> ("task out"=w900:refnum<k21>, "error out"=w901:errorcluster)  [unwired: 10 in, 1 out]
                  }
                  frame True {
                  }
                }
              }
            }
            n852 = Index Array(array=w882) -> (element #1=w871:bool, element #2=w865:bool, element #3=w870:bool, element #4=w869:bool, element #5=w868:bool, element #6=w867:bool, element #7=w866:bool)  [unwired: 7 in]
            n853 = call "Counts to Triac Direction.vi"("CCW ctr"=w818, "CW ctr"=w819) -> ("CW"=w857:bool, "CCW"=w858:bool)  [unwired: 8 in]
            n854 = case shown="False" w832 {
              tunnel: w835 -> [w928 w930]
              tunnel: w834 -> [w927 w929]
              tunnel: [w926 w930] -> w873
              tunnel: [w925 w929] -> w872
              tunnel: w815 -> [w924 _]
              tunnel: w814 -> [w923 _]
              frame False {
                n855 = property class="DAQmx Channel"(reference=w928, error in=w927, "CO.Pulse.Freq"=w924, "CO.Pulse.DutyCyc"=w923) -> (reference out=w926:refnum<k21>, error out=w925:errorcluster)
              }
              frame True {
              }
            }
            n856 = Select(t=DAQ_States."Run" ("States"), s=w805, f=DAQ_States."Shutdown" ("States")) -> (s? t:f=w853:T48)
          }
          frame "Shutdown" {
            w971 = 0.0
            w968 = FALSE ("element")
            # "Hall Sensor"
            # "Motor TRIAC CCW"
            # "Motor TRIAC CW"
            # "Relay Controls"
            # "TRIAC Outputs"
            # "AO for ADC"
            n857 = local read "AC Power"() -> (w956:bool)
            n858 = Build Array(w956, w968, w968) -> (w983:bool[])
            n859 = Build Array(w971, w971, w971) -> (w970:dbl[])
            n860 = call-poly <vilib>:"DAQmx Write.vi"("task/channels in"=w982, "data"=w983, "error in"=w955) -> ("task out"=w976:refnum<k21>, "error out"=w977:errorcluster)  [unwired: 10 in, 1 out]
            n861 = call-poly <vilib>:"DAQmx Write.vi"("task/channels in"=w963, "data"=FALSE, "error in"=w932) -> ("task out"=w962:refnum<k21>, "error out"=w961:errorcluster)  [unwired: 10 in, 1 out]
            n862 = call-poly <vilib>:"DAQmx Write.vi"("task/channels in"=w979, "data"=w970, "error in"=w940) -> ("task out"=w981:refnum<k21>, "error out"=w980:errorcluster)  [unwired: 10 in, 1 out]
            n863 = call "Time Delay4"("error in (no error)"=w977, "Delay Time (s)"=2.0) -> ("error out"=w975:errorcluster)  [unwired: 9 in]
            n864 = call <vilib>:"DAQmx Clear Task.vi"("task in"=w967, "error in"=w933) -> ("error out"=w966:errorcluster)  [unwired: 13 in]
            n865 = call <vilib>:"DAQmx Clear Task.vi"("task in"=w931, "error in"=w957) -> ("error out"=w988:errorcluster)  [unwired: 13 in]
            n866 = call <vilib>:"DAQmx Clear Task.vi"("task in"=w976, "error in"=w975) -> ("error out"=w954:errorcluster)  [unwired: 13 in]
            n867 = call <vilib>:"DAQmx Clear Task.vi"("task in"=w981, "error in"=w980) -> ("error out"=w947:errorcluster)  [unwired: 13 in]
            n868 = call <vilib>:"DAQmx Clear Task.vi"("task in"=w973, "error in"=w939) -> ("error out"=w972:errorcluster)  [unwired: 13 in]
            n869 = call <vilib>:"DAQmx Clear Task.vi"("task in"=w985, "error in"=w938) -> ("error out"=w974:errorcluster)  [unwired: 13 in]
            n870 = call <vilib>:"DAQmx Clear Task.vi"("task in"=w986, "error in"=w937) -> ("error out"=w936:errorcluster)  [unwired: 13 in]
            n871 = call <vilib>:"DAQmx Clear Task.vi"("task in"=w962, "error in"=w961) -> ("error out"=w965:errorcluster)  [unwired: 13 in]
            n872 = property on="Motor Current" class="Slide (strict)"(error in=w947, "Value"=2.5 ("Motor Current")) -> (error out=w945:errorcluster)  [unwired: 1 in, 1 out]
            n873 = property on="Turn On DAQ" class="Bool (strict)"(error in=w954, "Value"=FALSE ("Turn On DAQ")) -> (error out=w952:errorcluster)  [unwired: 1 in, 1 out]
            n874 = property on="Basket RPM" class="DigNum (strict)"(error in=w936, "Value"=1.0 ("Basket RPM")) -> (error out=w935:errorcluster)  [unwired: 1 in, 1 out]
            n875 = property on="Temperature" class="Slide (strict)"(error in=w945, "Value"=2.5 ("Temperature")) -> (error out=w943:errorcluster)  [unwired: 1 in, 1 out]
            n876 = property on="Mode Shift FB" class="Bool (strict)"(error in=w952, "Value"=FALSE ("Mode Shift FB")) -> (error out=w950:errorcluster)  [unwired: 1 in, 1 out]
            n877 = property on="Lid Status" class="Bool (strict)"(error in=w950, "Value"=FALSE ("Lid Status")) -> (error out=w949:errorcluster)  [unwired: 1 in, 1 out]
            n878 = property on="Pressure" class="Slide (strict)"(error in=w943, "Value"=0.0 ("Pressure")) -> (error out=w942:errorcluster)  [unwired: 1 in, 1 out]
          }
          frame "Exit" {
            w1006 = FALSE ("element")
            w1024 = 0.0
            n879 = local read "AC Power"() -> (w1007:bool)
            n880 = Build Array(w1007, w1006, w1006) -> (w1003:bool[])
            n881 = call-poly <vilib>:"DAQmx Write.vi"("task/channels in"=w999, "data"=w1003, "error in"=w1002) -> ("task out"=w1000:refnum<k21>, "error out"=w1005:errorcluster)  [unwired: 10 in, 1 out]
            n882 = Build Array(w1024, w1024, w1024) -> (w1027:dbl[])
            n883 = call-poly <vilib>:"DAQmx Write.vi"("task/channels in"=w1011, "data"=FALSE, "error in"=w1010) -> ("task out"=w1009:refnum<k21>, "error out"=w1008:errorcluster)  [unwired: 10 in, 1 out]
            n884 = call-poly <vilib>:"DAQmx Write.vi"("task/channels in"=w1026, "data"=w1027, "error in"=w1025) -> ("task out"=w1023:refnum<k21>, "error out"=w1022:errorcluster)  [unwired: 10 in, 1 out]
            n885 = call "Time Delay"("error in (no error)"=w1005, "Delay Time (s)"=2.0) -> ("error out"=w1001:errorcluster)  [unwired: 9 in]
            n886 = case shown="True" w1035 {
              tunnel: w1000 -> [_ w1087]
              tunnel: w1055 -> [_ w1086]
              tunnel: [w1059 w1085] -> w1014
              tunnel: [w1060 w1084] -> w1054
              tunnel: [w1056 w1083] -> w994
              tunnel: [w1062 w1082] -> w997
              tunnel: [w1063 w1081] -> w1053
              tunnel: w1049 -> [_ w1080]
              tunnel: w1048 -> [_ w1079]
              tunnel: [w1061 w1078] -> w1047
              tunnel: w1045 -> [_ w1077]
              tunnel: [w1058 w1076] -> w1044
              tunnel: w1009 -> [_ w1075]
              tunnel: [w1057 w1074] -> w992
              tunnel: w1040 -> [w1063 w1073]
              tunnel: w1001 -> [w1062 w1072]
              tunnel: w1039 -> [w1061 w1071]
              tunnel: w1038 -> [w1060 w1070]
              tunnel: w1037 -> [w1059 w1069]
              tunnel: w1036 -> [w1058 w1068]
              tunnel: w1008 -> [w1057 w1067]
              tunnel: w1034 -> [_ w1066]
              tunnel: w1023 -> [_ w1065]
              tunnel: w1022 -> [w1056 w1064]
              frame False {
              }
              frame True {
                # "Hall Sensor"
                # "Motor TRIAC CCW"
                # "Motor TRIAC CW"
                # "Relay Controls"
                # "TRIAC Outputs"
                # "AO for ADC"
                n887 = call <vilib>:"DAQmx Clear Task.vi"("task in"=w1077, "error in"=w1068) -> ("error out"=w1076:errorcluster)  [unwired: 13 in]
                n888 = call <vilib>:"DAQmx Clear Task.vi"("task in"=w1075, "error in"=w1067) -> ("error out"=w1074:errorcluster)  [unwired: 13 in]
                n889 = call <vilib>:"DAQmx Clear Task.vi"("task in"=w1066, "error in"=w1073) -> ("error out"=w1081:errorcluster)  [unwired: 13 in]
                n890 = call <vilib>:"DAQmx Clear Task.vi"("task in"=w1087, "error in"=w1072) -> ("error out"=w1082:errorcluster)  [unwired: 13 in]
                n891 = call <vilib>:"DAQmx Clear Task.vi"("task in"=w1065, "error in"=w1064) -> ("error out"=w1083:errorcluster)  [unwired: 13 in]
                n892 = call <vilib>:"DAQmx Clear Task.vi"("task in"=w1079, "error in"=w1071) -> ("error out"=w1078:errorcluster)  [unwired: 13 in]
                n893 = call <vilib>:"DAQmx Clear Task.vi"("task in"=w1080, "error in"=w1070) -> ("error out"=w1084:errorcluster)  [unwired: 13 in]
                n894 = call <vilib>:"DAQmx Clear Task.vi"("task in"=w1086, "error in"=w1069) -> ("error out"=w1085:errorcluster)  [unwired: 13 in]
              }
            }
            n895 = call <vilib>:"Clear Errors.vi"("error in (no error)"=w994, "specific error code to clear (0: all)"=-200088) -> ("error out"=w993:errorcluster)  [unwired: 4 in, 1 out]
            n896 = call <vilib>:"Clear Errors.vi"("error in (no error)"=w997, "specific error code to clear (0: all)"=-200088) -> ("error out"=w996:errorcluster)  [unwired: 4 in, 1 out]
            n897 = call <vilib>:"Clear Errors.vi"("error in (no error)"=w992, "specific error code to clear (0: all)"=-200088) -> ("error out"=w991:errorcluster)  [unwired: 4 in, 1 out]
            n898 = property on="Turn On DAQ" class="Bool (strict)"(error in=w996, "Value"=FALSE ("Turn On DAQ")) -> (error out=w1032:errorcluster)  [unwired: 1 in, 1 out]
            n899 = property on="Motor Current" class="Slide (strict)"(error in=w993, "Value"=2.5 ("Motor Current")) -> (error out=w1020:errorcluster)  [unwired: 1 in, 1 out]
            n900 = property on="Basket RPM" class="DigNum (strict)"(error in=w1014, "Value"=1.0 ("Basket RPM")) -> (error out=w1013:errorcluster)  [unwired: 1 in, 1 out]
            n901 = property on="Mode Shift FB" class="Bool (strict)"(error in=w1032, "Value"=FALSE ("Mode Shift FB")) -> (error out=w1030:errorcluster)  [unwired: 1 in, 1 out]
            n902 = property on="Temperature" class="Slide (strict)"(error in=w1020, "Value"=2.5 ("Temperature")) -> (error out=w1018:errorcluster)  [unwired: 1 in, 1 out]
            n903 = property on="Lid Status" class="Bool (strict)"(error in=w1030, "Value"=FALSE ("Lid Status")) -> (error out=w1028:errorcluster)  [unwired: 1 in, 1 out]
            n904 = property on="Pressure" class="Slide (strict)"(error in=w1018, "Value"=0.0 ("Pressure")) -> (error out=w1016:errorcluster)  [unwired: 1 in, 1 out]
          }
        }
        "DAQ Status" <- w549
        "DAQ On?" <- w547
        "Triac CW" <- w544
        "Traic CCW" <- w543
        "Cold Valve" <- w520
        "Recirc Pump" <- w521
        "Mode Shift" <- w508
        "Drain Pump" <- w522
        "Fabric SoftValve" <- w517
        "Spray/Rinse Valve" <- w518
        "Hot Valve" <- w519
        n905 = case shown="True" "MS (M - A)" {
          tunnel: w512 -> [w573 w584]
          tunnel: [w573 w583] -> w509
          tunnel: w508 -> [_ w574]
          frame False {
          }
          frame True {
            n906 = Equal?(x=w574, y=TRUE) -> (x = y?=w581:bool)
            n907 = case shown="True" w581 {
              tunnel: w584 -> [w589 w591]
              tunnel: [w589 w590] -> w576
              frame False {
              }
              frame True {
                n908 = Increment(x=w591) -> (x+1=w590:dbl)
              }
            }
            n909 = In Range and Coerce(upper limit=24.0, x=w576, lower limit=15.0) -> (In Range?=w578:bool)  [unwired: 1 out]
            n910 = case shown="True" w578 {
              frame False {
                n911 = property on="Mode Shift FB" class="Bool (strict)"("Value"=FALSE ("Mode Shift FB")) -> ()  [unwired: 2 in, 2 out]
              }
              frame True {
                n912 = property on="Mode Shift FB" class="Bool (strict)"("Value"=TRUE ("Mode Shift FB")) -> ()  [unwired: 2 in, 2 out]
              }
            }
            n913 = Greater Or Equal?(x=w576, y=24.0) -> (x >= y?=w575:bool)
            n914 = case shown="True" w575 {
              tunnel: w576 -> [w585 _]
              tunnel: [w585 0.0] -> w583
              frame False {
              }
              frame True {
              }
            }
          }
        }
        n915 = case shown="False" w515 {
          tunnel: w513 -> [w593 _]
          tunnel: [w592 0.0] -> w510
          frame False {
            n916 = Increment(x=w593) -> (x+1=w592:dbl)
          }
          frame True {
          }
        }
        n917 = Merge Errors(w558, w557, w556, w555, w554, w553, w552, w551, w550) -> (w559:errorcluster)
        n918 = call "Error_Control.vi"("Error In"=w559) -> ("Error Out"=w571:errorcluster)  [unwired: 14 in]
      }
      n919 = Close File(refnum=w35, error in=w105) -> (error out=w36:errorcluster)  [unwired: 1 out]
      n920 = call "GEA2 Stop.vi"("GEA2 Reference In"=w129, "Error In"=w130) -> ("Error Out"=w117:errorcluster)  [unwired: 13 in]
      n921 = Close File(refnum=w53, error in=w55) -> (error out=w54:errorcluster)  [unwired: 1 out]
      n922 = Merge Errors(w54, w36, w47, w131, w117, w104) -> (w31:errorcluster)
      n923 = Obtain Queue(name (unnamed)="Continuous Send", element data type=Cont_Send_States."Run" ("State"), error in (no error)=w31) -> (queue out=w52:refnum<queue>, error out=w51:errorcluster)  [unwired: 2 in, 1 out]
      n924 = Obtain Queue(name (unnamed)="ERD Loop", element data type=T49 {"Data"=variant, "State"=enum."Read ERDs"} ("Data"), error in (no error)=w31) -> (queue out=w112:refnum<queue>, error out=w111:errorcluster)  [unwired: 2 in, 1 out]
      n925 = Obtain Queue(name (unnamed)="GEA2", element data type=T47 {"Data"=variant, "State"=enum."Add to Log"} ("Data"), error in (no error)=w31) -> (queue out=w121:refnum<queue>, error out=w120:errorcluster)  [unwired: 2 in, 1 out]
      n926 = Obtain Queue(name (unnamed)="DAQ", element data type=DAQ_States."Wait for Init" ("States"), error in (no error)=w31) -> (queue out=w107:refnum<queue>, error out=w108:errorcluster)  [unwired: 2 in, 1 out]
      n927 = Release Queue(queue=w52, error in (no error)=w51) -> (error out=w50:errorcluster)  [unwired: 1 in, 2 out]
      n928 = Release Queue(queue=w112, error in (no error)=w111) -> (error out=w100:errorcluster)  [unwired: 1 in, 2 out]
      n929 = Release Queue(queue=w121, error in (no error)=w120) -> (error out=w101:errorcluster)  [unwired: 1 in, 2 out]
      n930 = Release Queue(queue=w107, error in (no error)=w108) -> (error out=w102:errorcluster)  [unwired: 1 in, 2 out]
      n931 = Merge Errors(w50, w100, w101, w102) -> (w99:errorcluster)
      n932 = call "Error_Control.vi"("Command (Handle Errors)"=Error_Command."Report Errors", "Error In"=w99) -> ("Error Out"=w92:errorcluster)  [unwired: 13 in]
    }
    frame Error {
    }
  }
  n933 = call <vilib>:"Simple Error Handler.vi"("error in (no error)"=w3) -> ("error out"=→"Error Out":errorcluster)  [unwired: 4 in, 4 out]
